vi "ZController.vi"() -> ()   [LabVIEW 2016]
uses:
  controls/FPGAVIreferenceTypeDef.ctl
  controls/Enum.ctl
  <vilib>/event_ctls.llb/lveventtype.ctl
  controls/EnumSM.ctl
  Course Project/support/Message Queue/Message Cluster.ctl
  <vilib>/FPGAPlugInAG/USB-7856R OEM/niLvFpga_Close_USB-7856R OEM.vi
  <vilib>/FPGAPlugInAG/USB-7856R OEM/niLvFpga_Reset_USB-7856R OEM.vi
  <vilib>/rvi/errors/niLvFpgaAdjustHostInterfaceError.vi
  <vilib>/RVI Host/nirviSupport.llb/nirviErrorClusterFromErrorCode.vi
  <vilib>/Utility/config.llb/Read Key (Boolean).vi
  <vilib>/Utility/config.llb/Read Key (Double).vi
  <vilib>/Utility/config.llb/Read Key (String).vi
  <vilib>/Utility/config.llb/Read Key (U32).vi
  <vilib>/Utility/config.llb/Write Key (String).vi
  <vilib>/Utility/config.llb/Write Key (U32).vi
  <vilib>/Utility/config.llb/Write Key (Double).vi
  <vilib>/Utility/config.llb/Write Key (Boolean).vi
  <vilib>/rvi/interface/nirviCloseFPGA/nirviCloseFPGA.xnode
  FPGA Bitfiles/qnmController797_usbRIO_controllerFPGAmu.lvbitx
  <vilib>/rvi/interface/nirviMethod/nirviMethod.xnode
  <vilib>/rvi/interface/nirviReadWriteControl/nirviReadWriteControl.xnode
  controls/FPGAVIreferenceTypeDefScanEngine.ctl
  <vilib>/regexp/Match Regular Expression.xnode
  Course Project/support/Message Queue/Message Queue.lvlib
  Course Project/support/User Event - Stop/User Event - Stop.lvlib
  NiFpgaLv.dll
  <vilib>/Utility/config.llb/NI_LVConfig.lvlib
  <vilib>/FPGAPlugInAG/USB-7856R OEM/niLvFpga_AcknowledgeIrq_USB-7856R OEM.vi
  <vilib>/rvi/interface/nirviMethod/StockFPGA_InlinedMethodWaitForSingleIRQ.vi
  <vilib>/FPGAPlugInAG/USB-7856R OEM/niLvFpga_WaitOnIrq_USB-7856R OEM.vi
panel:
  in  "ms":u32=50 format="%.0fms"
  in  "ZControllerThumbnail":enum32{"Z controller", "Other Config"}(tab)
  out "Surface reached":bool
  in  "Steps":u32=16 format="%#.0p"
  out "Approaching?":bool
  in  "Mode":enum16{"Contact", "OR Tapping", "Aux"}(ring)
  in  "Feedback On":bool caption="Enable"
  in  "liftHeight":dbl=1e-07 format="%.2pm"
  in  "Lift":bool
  in  "Motor":cluster{"Up":bool, "Down":bool}
  in  "Z (m)":dbl(slide) scale=1.75e-06..-1.75e-06 scale format="%#.2p"
  in  "PID":T1={"Setpoint"=0.05, "P Gain"=0.0001, "I Gain"=0.0003} {"I Gain" max=20.0 format="%.3p"; "P Gain" format="%.3p"; "Setpoint" format="%_4pV"}
  in  "Withdraw":bool
  in  "AutoApproach":cluster{"Stop":bool, "Start":bool}
  in  "Wait":u32=1 format="%.0fms"
  in  "DCVoltage":sgl=1.2 format="%#_3pV"
  in  "IO Frequency":u32=1000000 format="%.1p"
  in  "Relative Setpoint":bool
  in  "SafeTip":T2 {"SafeTipSignal" items=["AI0", "AI1", "AI2", "AI3", "AI4", "AI5", "AI6", "AI7"]; "SafeTipValue" format="%_3p"}
  in  "Slow":bool
  in  "Beep when finished":bool=TRUE
  in  "Withdraw/landed":bool=TRUE
  in  "Ztreshold":dbl=0.949999988079071
  in  "zMoveTresh":fxp<+/-,29,2>=0.009999997913837433 format="%#_4g"
  in  "InvertHeight":bool=TRUE
  in  "Type":T3(ring)
  in  "Decimations":cluster{"Withdraw":u16, "ManualMove":u16}={"Withdraw"=5, "ManualMove"=5}
  in  "Step Up":enum16{"Z+", "Z-"}(ring)=enum."Z-"
  out "Display Z":bool=TRUE
  in  "WaveSize":u16=101
  out "Zstep":i32
  # "Mode"
  # "Z (m)"
  # "Motor"
  # "Feedback"
  # "Approach"
  # "Motor"
  # "SetPoint"
  # "Manual PID"
  # "Auto approach"
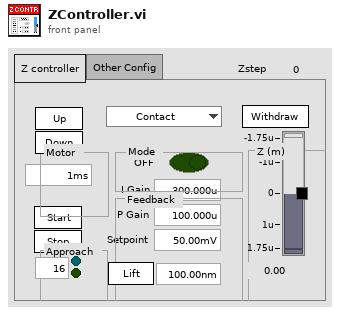
[diagram p1: front panel]
types:
  T1 = cluster{"Setpoint":dbl, "P Gain":dbl, "I Gain":dbl}
  T2 = cluster{"SafeTipValue":dbl, ">/<":enum16{">", "<"}, "SafeTipOn":bool, "SafeTipSignal":u16}
  T3 = enum16{"Step motor", "DC motor", "Stepper Motor Driver", "Stick-Slip"}
  T4 = typedef "FPGAVIreferenceTypeDef.ctl" = refnum<k20>
  T5 = typedef "Enum.ctl" = enum16{"Init", "Read", "Write"}
  T6 = enum16{"fractional", "engineering", "exponential"}
  T7 = enum16{"Vert. Deflection", "Horiz. Deflection", "Amplitude", "..."}
  T8 = cluster{"inverseDecimation":fxp<+,22,0>, "decimation":u16, "waveSize":u16, "pixelDecimation":u16}
  T9 = cluster{"enableManualMotion":bool, "doMove":bool, "integratorTarget":fxp<+/-,22,2>, "clocks":cluster{"inverseDecimation":fxp<+,22,0>, "decimation":u16, "waveSize":u16, "pixelDecimation":u16}}
  T10 = typedef "EnumSM.ctl" = enum16{"Init.Calibrations", "Init.Excitation", "Init.StepMotor", "Init.FeedbackMotion", "Init.Scan", "Init.Signals", "Init.System", "Init.Waveform", "Init.ZController", "Send.Waveform", "Correct.Hysteresis"}
  T11 = cluster{"Width":dbl, "Height":dbl, "X Offset":dbl, "Y Offset":dbl, "Angle":dbl, "Pixels/Line":u16, "Lines":u16, "Time/Line":dbl, "Scan Rate":dbl}
  T12 = enum8{"Enabled", "Disabled", "Disabled and Grayed Out"}
  T13 = cluster{"setPoint":fxp<+/-,17,1>, "pGain":dbl, "iGain":dbl, "setPointAlt":fxp<+/-,17,1>}
  T14 = enum16{"Contact", "OR Tapping", "Aux", "Intermittent Contact"}
  T15 = cluster{"enableManualMotion":bool, "doMove":bool, "liftHeight":dbl}
  T16 = typedef "Message Queue.lvlib/Message Cluster.ctl" = cluster{"Message":string, "Données de message":variant}
  T17 = enum32{"Invalid", "Standard", "Closed", "Hidden", "Minimized", "Maximized"}
  T18 = enum32{"Bad", "Idle", "Run top level", "Running"}
  T19 = typedef "lveventtype.ctl" = enum32{"Null", "Timeout", "Annotation Menu Selection", "Annotation Menu Selection?", "App Instance Close", "App Instance Close?", "Autoscale Range Change", "Bookmark Info Change", "Cell Edit", "Cell Edit?", "Cursor Grab", "Cursor Grab?", "Cursor Menu Selection", "Cursor Menu Selection?", "Cursor Move", "Cursor Release", "Data Change", "Direction Change", "Display State Change", "Drag Ended", "Drag Enter", "Drag Leave", "Drag Over", "Drag Source Update", "Drag Starting", "Drag Starting?", "Drop", "Exec State Change", "Key Down", "Key Down?", "Key Repeat", "Key Repeat?", "Key Up", "Listbox Double Click", "Menu Activation?", "Menu Selection (App)", "Menu Selection? (App)", "Menu Selection (User)", "Mouse Down", "Mouse Down?", "Mouse Enter", "Mouse Leave", "Mouse Move", "Mouse Up", "Mouse Wheel", "NI Security User Change (App)", "Pane Size", "Panel Close", "Panel Close?", "Panel Resize", "Plot Attribute Change", "Scale Range Change", "Shortcut Menu Activation?", "Shortcut Menu Selection (App)", "Shortcut Menu Selection? (App)", "Shortcut Menu Selection (User)", "Tree Double Click", "Tree Drag", "Tree Drag?", "Tree Drop", "Tree Drop?", "Tree Item Close", "Tree Item Close?", "Tree Item Open", "Tree Item Open?", "User Event", "Value Change"}
  T20 = typedef "Message Queue.lvlib/All Message Queues.ctl" = cluster{"IU":refnum<queue>}
  T21 = typedef "NI_LVConfig.lvlib/Config Data RefNum.ctl" = refnum<k1>
  T22 = cluster{"calibName":string[], "calibParameters":cluster{"Sensitivity":cluster{"Sens X":dbl, "Sens Y":dbl, "Sens Z":dbl}, "Range":cluster{"Range X":dbl, "Range Y":dbl, "Range Z":dbl}, "HV gain":cluster{"HV gain X":dbl, "HV gain Y":dbl, "HV gain Z":dbl}}[], "calibIndex":i32}
  T23 = cluster{"Sensitivity":cluster{"Sens X":dbl, "Sens Y":dbl, "Sens Z":dbl}, "Range":cluster{"Range X":dbl, "Range Y":dbl, "Range Z":dbl}, "HV gain":cluster{"HV gain X":dbl, "HV gain Y":dbl, "HV gain Z":dbl}}[]
  T24 = cluster{"Sensitivity":cluster{"Sens X":dbl, "Sens Y":dbl, "Sens Z":dbl}, "Range":cluster{"Range X":dbl, "Range Y":dbl, "Range Z":dbl}, "HV gain":cluster{"HV gain X":dbl, "HV gain Y":dbl, "HV gain Z":dbl}}
  T25 = typedef "FPGAVIreferenceTypeDefScanEngine.ctl" = refnum<k20>
  T26 = cluster{"liftHeight":fxp<+/-,15,4>, "disengagePos":fxp<+/-,22,1>}
  T27 = cluster{"upperLimit":fxp<+/-,28,4>, "lowerLimit":fxp<+/-,28,4>}
  T28 = cluster{"Width":bool, "Height":bool, "X Offset":bool, "Y Offset":bool, "Angle":bool, "Pixels/Line":bool, "Lines":bool, "Time/Line":bool, "Scan Rate":bool}
  T29 = cluster{"target ":i16, "increment":i16, "ClockDivider":i16, "axis":enum16{"none", "x", "y", "z"}}
  T30 = cluster{"sicm.p.enable":bool, "sicm.p.adaptiveStepDown":bool, "sicm.p.relSetpoint":bool}
  T31 = cluster{"ort.p.winSizeP2":u16, "ort.p.syncPoint":u16, "ort.p.useSyncPoint":bool, "ort.p.bypassAvg":bool, "ort.p.searchBounds":cluster{"maxSearchLower":u16, "maxSearchUpper":u16}}
  T32 = cluster{"scanEngineHz":u32, "feedbackHz":u32, "sicmHz":u32, "rampHz":u32}
  T33 = cluster{"SafeTipValue":dbl, ">/<":enum16{">", "<"}, "SafeTipSignal":u16}
  T34 = cluster{"enableManualMotion":bool, "doMove":bool, "HeightTarget(0-2)":dbl}
  T35 = cluster{"enableManualMotion":bool, "doMove":bool, "Height Lift":dbl, "Caption.Text":string}
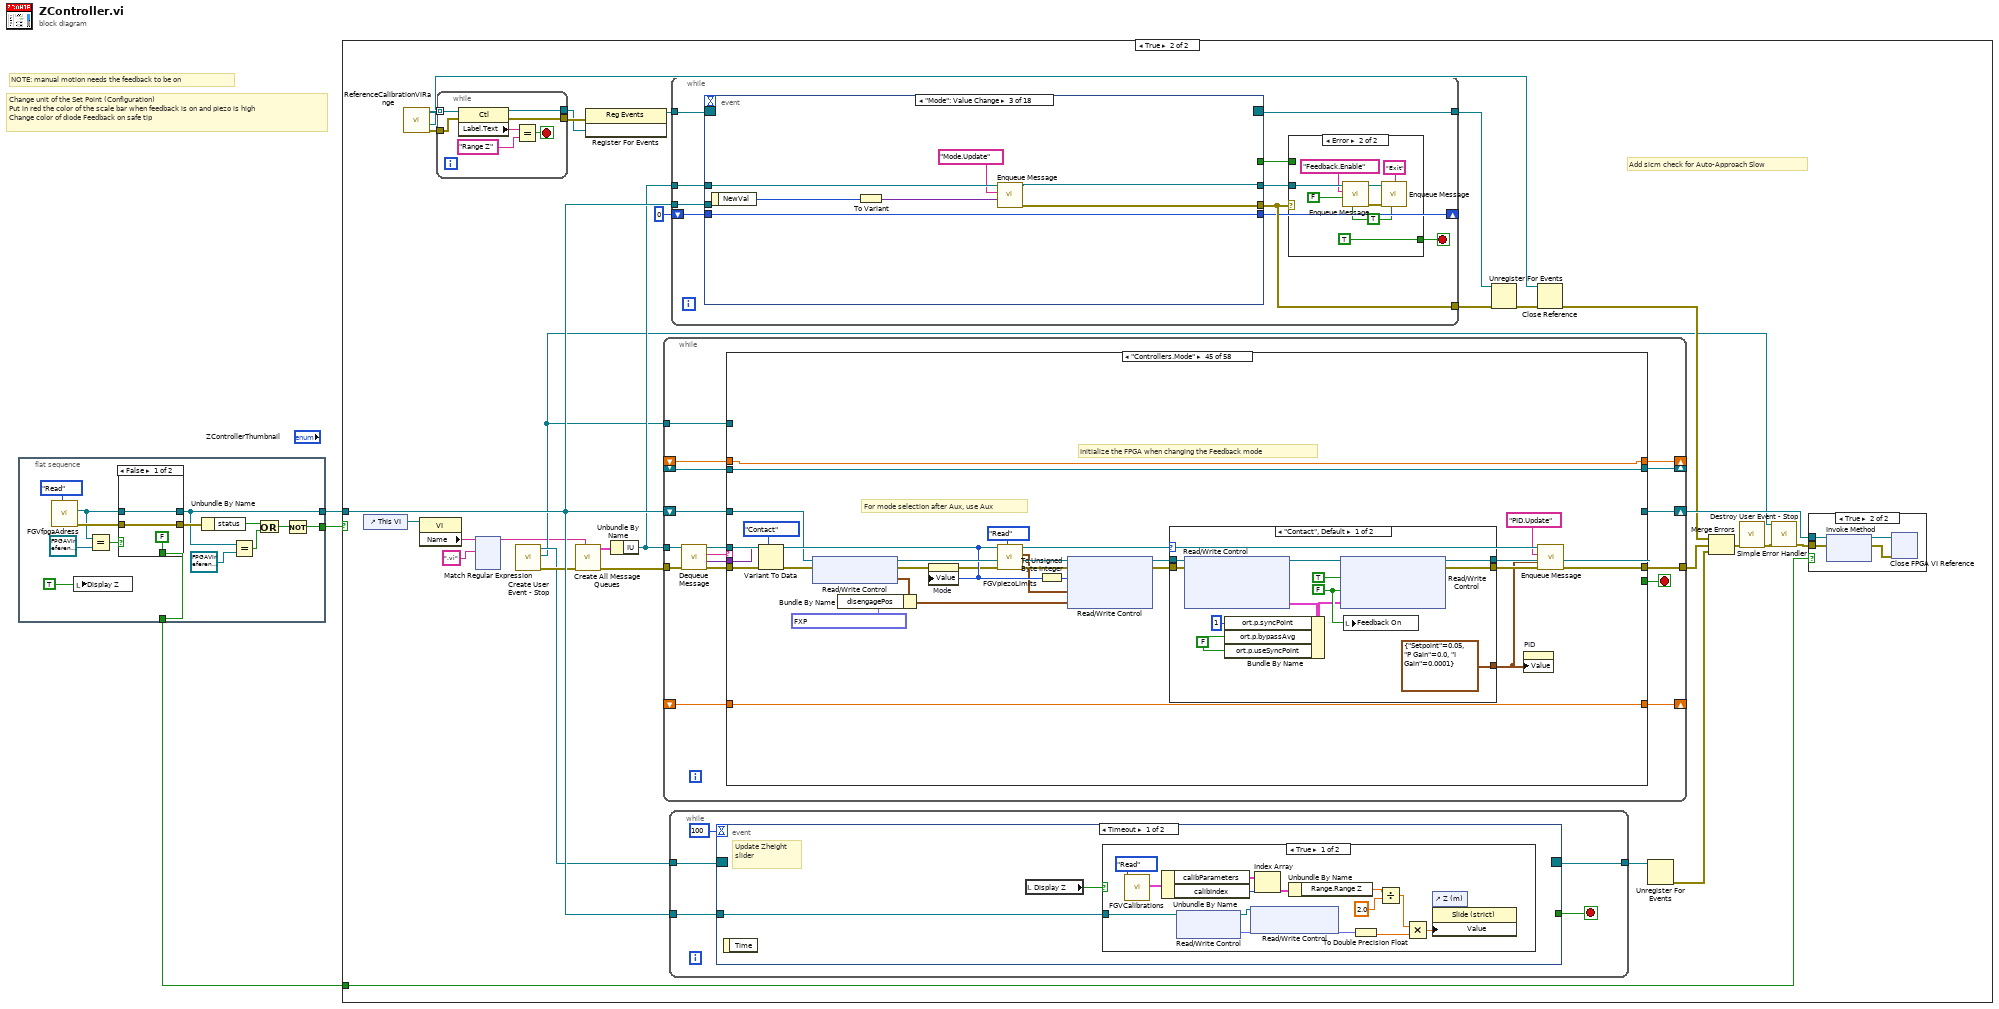
[diagram p0: block diagram]
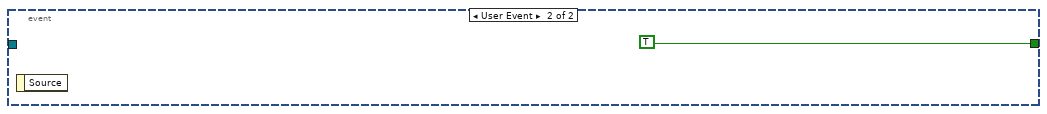
[diagram p5: hidden frame]
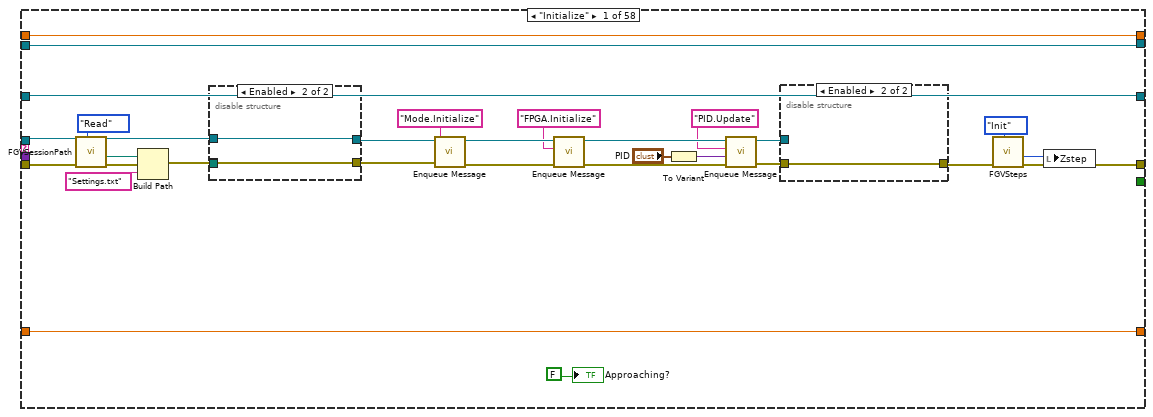
[diagram p6: hidden frame]
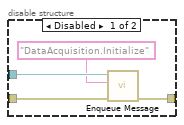
[diagram p7: hidden frame]
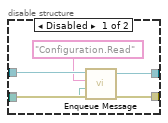
[diagram p8: hidden frame]
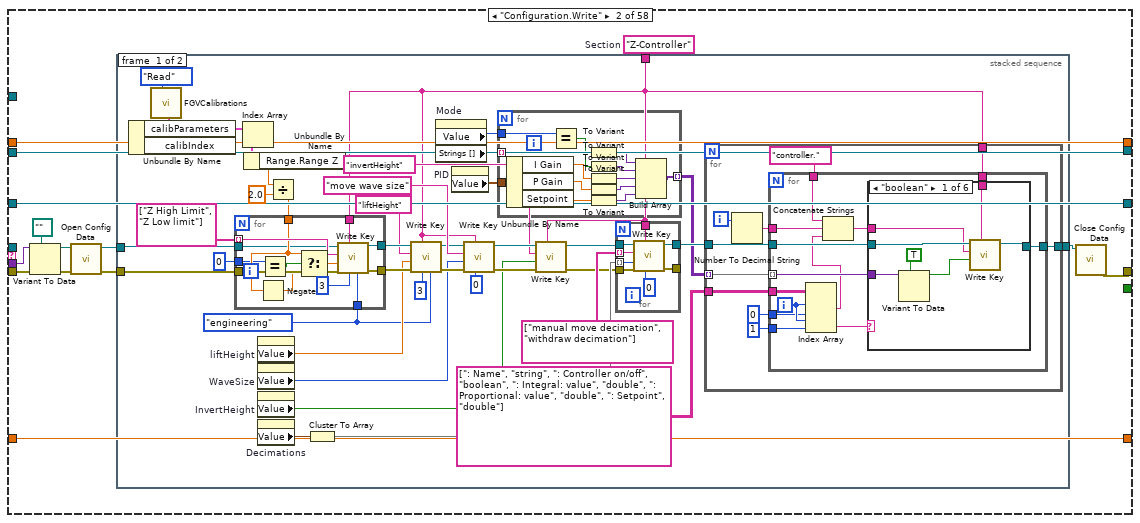
[diagram p9: hidden frame]
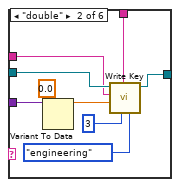
[diagram p10: hidden frame]
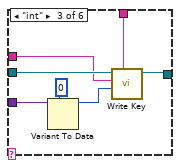
[diagram p11: hidden frame]
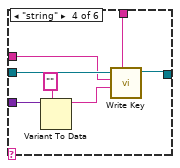
[diagram p12: hidden frame]
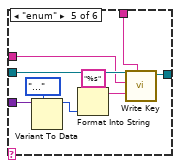
[diagram p13: hidden frame]
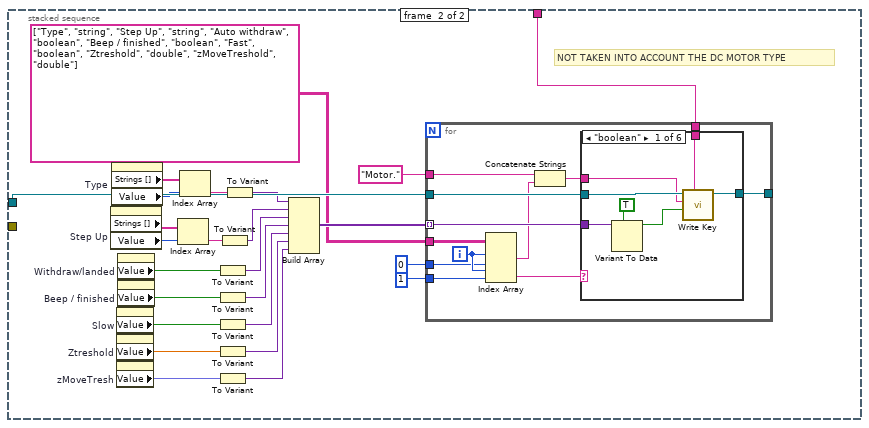
[diagram p15: hidden frame]
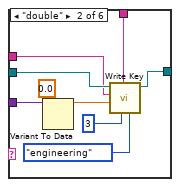
[diagram p16: hidden frame]
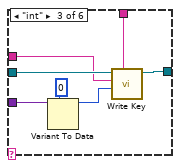
[diagram p17: hidden frame]
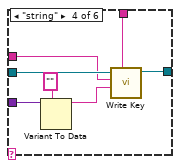
[diagram p18: hidden frame]
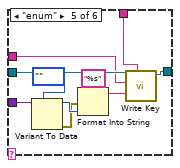
[diagram p19: hidden frame]
diagram:
  # "Change unit of the Set Point (Configuration)\nPut in red the color of the scale bar when feedback is on and piezo is high\nChange color of diode Feedback on safe tip"
  # "NOTE: manual motion needs the feedback to be on"
  n1 = flat-sequence {
    tunnel: [w6] -> w3
    tunnel: [w5] -> w2
    tunnel: [w4] -> _
    tunnel: [w4] -> w1
    frame #0 {
      n2 = call "FGVfpgaAdress.vi"("Enum"=Enum."Read") -> ("error out"=w17:errorcluster, "FPGA VI Reference Out"=w10:T4)  [unwired: 5 in, 4 out]
      n3 = local write "Display Z"(TRUE ("display height")) -> ()
      n4 = Equal?(x=w10, y=T4 refnum ("FPGA VI Reference Out")) -> (x = y?=w15:bool)
      n5 = case shown="False" w15 {
        tunnel: [w20 w26] -> w6
        tunnel: [w19 w25] -> w7
        tunnel: w17 -> [w19 w24]
        tunnel: w10 -> [w20 w23]
        tunnel: [FALSE TRUE] -> w4
        frame False {
        }
        frame True {
          n6 = call "FGVfpgaAdress.vi"("Enum"=Enum."Init", "error in"=w24, "FPGA VI Reference In"=w23) -> ("error out"=w25:errorcluster, "FPGA VI Reference Out"=w26:T4)  [unwired: 3 in, 4 out]
        }
      }
      n7 = Unbundle By Name(w7) -> ("status"=w12:bool)
      n8 = Equal?(x=w6, y=T4 refnum ("FPGA VI Reference Out")) -> (x = y?=w13:bool)
      n9 = Or(x=w12, y=w13) -> (x .or. y?=w14:bool)
      n10 = Not(x=w14) -> (.not. x?=w5:bool)
    }
  }
  n11 = case shown="True" w2 {
    tunnel: w3 -> [_ w55]
    tunnel: w1 -> [_ w41]
    frame False {
    }
    frame True {
      # "Add sicm check for Auto-Approach Slow"
      n12 = control-ref of="This VI"() -> (w31:refnum<vi>)
      n13 = call "ReferenceCalibrationViRange.vi"() -> ("error out"=w45:errorcluster, "vi reference"=w39:refnum<vi>, "Ranges"=w46:refnum<vi>[])  [unwired: 8 in, 1 out]
      n14 = property class="VI"(reference=w31) -> ("Name"=w30:string)  [unwired: 1 in, 2 out]
      n15 = while {
        tunnel: w46 -> [w180] mode=indexing
        tunnel: [w181] -> w44
        tunnel: w45 -> [w179]
        tunnel: [w175] -> w43
        stop <- w176 stop-if-true
        n16 = property class="Ctl"(reference=w180, error in=w179) -> (reference out=w175:refnum<vi>, error out=w181:errorcluster, "Label.Text"=w178:string)
        n17 = Equal?(x=w178, y="Range Z") -> (x = y?=w176:bool)
      }
      n18 = xnode "Match Regular Expression"("input string"=w30, "regular expression"=".vi") -> ("before match"=w28:string)  [unwired: 4 in, 4 out]
      n19 = call "Create User Event - Stop.vi"() -> ("sortie d'erreur"=w38:errorcluster, "Événement utilisateur - Arrêt"=w32:refnum<user-event>, "Refnum Enregistrement à l'événement Arrêt"=w37:refnum<event-registration>)  [unwired: 9 in]
      n20 = call "Create All Message Queues.vi"("QueueName"=w28, "ErrorIn"=w38) -> ("ErrorOut"=w49:errorcluster, "MessageQueueOut"=w51:T20)  [unwired: 8 in]
      n21 = register-events(error in=w44, w43) -> (reference out=w47:refnum<event-registration>)  [unwired: 1 in, 1 out]
      n22 = Unbundle By Name(w51) -> ("IU"=w50:refnum<queue>)
      n23 = while {
        tunnel: w50 -> [w214]
        tunnel: w49 -> [w218]
        tunnel: [w219] -> w48
        shift-right: [w213] -> w56
        shift-left: w55 -> [w212]
        shift-right: [w210] -> _
        shift-left: _ -> [w209]
        shift-right: [w207] -> _
        shift-left: _ -> [w208]
        tunnel: w32 -> [w206]
        shift-right: [w204] -> _
        shift-left: _ -> [w205]
        stop <- w220 stop-if-true
        n24 = call "Dequeue Message.vi"("entrée d'erreur (pas d'erreur)"=w218, "File d'attente de messages"=w214) -> ("sortie d'erreur"=w217:errorcluster, "Données de message"=w216:variant, "Message"=w211:string, "File d'attente de message dup."=w215:refnum<queue>)  [unwired: 6 in]
        n25 = case "Conditions des messages" shown="\"Controllers.Mode\"" w211 {
          selector: w211 -> [_ _ _ _ _ _ _ _ _ _ _ _ _ _ _ _ _ _ _ _ _ _ _ _ _ _ _ _ _ _ _ _ _ _ _ _ _ _ _ _ _ _ _ _ _ _ _ _ _ _ _ _ _ _ _ _ _ w2503]
          tunnel: w215 -> [w248 _ _ w682 _ _ _ _ w811 w833 w923 _ w937 _ _ w1103 _ _ w1163 _ _ _ _ w1354 _ _ _ w1486 _ _ w1563 _ w1612 w1653 w1733 w1796 _ w1828 w1861 w1962 w2042 w2110 _ w2162 w2187 w2227 _ _ _ _ w2363 _ _ _ w2468 _ w2495 _]
          tunnel: w217 -> [w225 w266 w501 w659 w698 w735 w766 w781 w808 w831 w925 w930 w958 w1045 w1064 w1092 w1147 w1156 w1185 w1258 w1265 w1285 w1320 w1355 w1387 w1400 w1459 w1481 w1528 w1546 w1551 w1593 w1608 w1650 w1725 w1794 w1818 w1829 w1859 w1960 w2041 w2108 w2142 w2144 w2184 w2216 w2242 w2261 w2317 w2341 w2361 w2378 w2386 w2396 w2469 w2477 w2492 _]
          tunnel: [w241 w269 w503 w676 w698 w725 w767 w781 w803 w824 w910 w930 w944 w1053 w1064 w1079 w1146 w1156 w1159 w1257 w1265 w1270 w1322 w1348 w1373 w1418 w1433 w1485 w1521 w1546 w1555 w1590 w1607 w1648 w1728 w1797 w1818 w1830 w1853 w1954 w2038 w2111 w2142 w2145 w2168 w2212 w2242 w2256 w2316 w2342 w2351 w2367 w2386 w2394 w2463 w2478 w2493 w2501] -> w219
          tunnel: [_ _ _ _ _ _ _ _ _ _ _ _ _ _ _ _ _ _ _ _ _ _ _ _ _ _ _ _ _ _ _ _ _ _ _ _ _ _ _ _ _ _ _ _ _ _ _ _ _ _ _ _ _ _ _ _ TRUE _] -> w220
          tunnel: w216 -> [_ w265 w500 _ _ _ _ _ w809 w832 _ _ w957 _ _ w1090 _ _ w1184 _ _ w1284 w1318 _ w1386 w1426 _ _ w1527 _ _ _ _ _ _ _ _ _ _ _ w2040 _ _ w2143 w2185 w2214 _ w2260 _ w2340 _ w2377 _ w2388 _ _ _ _]
          tunnel: w212 -> [w235 w275 w507 w671 w697 w737 w764 w780 w804 w814 w922 w929 w965 w1059 w1063 w1100 w1149 w1155 w1198 w1260 w1264 w1283 w1302 w1349 w1382 w1406 w1458 w1484 w1530 w1545 w1547 w1592 w1602 w1649 w1724 w1791 w1817 w1827 w1858 w1959 w2035 w2109 w2141 w2158 w2181 w2220 w2241 w2278 w2330 w2334 w2360 w2380 w2385 w2398 w2472 w2483 w2491 w2499]
          tunnel: [w235 w275 w507 w681 w697 w726 w763 w780 w804 w814 w922 w929 w965 w1059 w1063 w1100 w1149 w1155 w1198 w1260 w1264 w1287 w1317 w1349 w1375 w1412 w1460 w1484 w1529 w1545 w1552 w1591 w1609 w1647 w1721 w1790 w1817 w1827 w1850 w1951 w2035 w2107 w2141 w2158 w2175 w2211 w2241 w2278 w2330 w2334 w2360 w2380 w2385 w2397 w2472 w2483 w2491 w2499] -> w213
          tunnel: [w232 w274 w506 w664 w683 w751 w776 w779 w784 w816 w907 w928 w964 w1058 w1062 w1099 w1151 w1154 w1197 w1259 w1263 w1273 w1311 w1345 w1364 w1397 w1445 w1483 w1531 w1544 w1561 w1595 w1611 w1652 w1732 w1800 w1816 w1825 w1836 w1938 w2034 w2104 w2140 w2157 w2174 w2226 w2240 w2277 w2329 w2333 w2355 w2366 w2384 w2417 w2471 w2482 w2489 w2498] -> w210
          tunnel: w209 -> [w232 w274 w506 _ _ w751 w776 w779 w784 w816 w907 w928 w964 w1058 w1062 w1099 w1151 w1154 w1197 w1259 w1263 w1273 w1311 w1345 w1364 w1397 w1445 w1483 w1531 w1544 w1561 w1595 w1611 w1652 w1732 w1800 w1816 w1825 w1836 w1938 w2034 w2104 w2140 w2157 w2174 w2226 w2240 w2277 w2329 w2333 w2355 _ w2384 w2417 w2471 w2482 w2489 w2498]
          tunnel: w208 -> [w231 w273 w505 w651 w696 w721 w775 w778 w783 w815 w906 w927 w950 w1052 w1061 w1097 w1145 w1153 w1166 w1256 w1262 w1272 w1301 w1344 w1363 w1395 w1444 w1482 w1525 w1543 w1560 w1594 w1610 w1651 w1731 w1799 w1815 w1824 w1835 w1937 w2033 w2103 w2139 w2156 w2172 w2225 w2239 w2276 w2328 w2332 w2354 w2365 w2383 w2416 w2470 w2481 w2488 w2497]
          tunnel: [w231 w273 w505 w661 w696 w721 w775 w778 w783 w813 w906 w927 w945 w1051 w1061 w1102 w1144 w1153 w1165 w1255 w1262 w1272 w1300 w1344 w1363 w1395 w1444 w1482 w1525 w1543 w1560 w1594 w1610 w1651 w1731 w1799 w1815 w1824 w1835 w1937 w2033 w2103 w2139 w2156 w2172 w2225 w2239 w2276 w2328 w2332 w2354 w2365 w2383 w2416 w2470 w2481 w2488 w2497] -> w207
          tunnel: w206 -> [_ _ _ _ _ _ _ _ _ _ _ _ _ _ _ _ _ _ _ _ _ _ _ _ _ _ _ _ _ _ _ _ _ _ _ _ _ _ _ _ _ _ _ _ _ _ _ _ _ _ _ _ _ _ _ _ w2487 _]
          tunnel: w205 -> [w221 w263 w494 _ w695 w701 w760 w777 w782 w812 w905 w926 w940 w1047 w1060 w1098 w1150 w1152 w1158 w1253 w1261 w1266 w1327 w1343 w1356 w1391 w1437 w1476 w1524 w1542 w1553 w1581 w1603 w1630 w1726 w1795 w1814 w1819 w1833 w1963 w2032 w2102 w2138 w2155 w2171 w2217 w2238 w2275 w2327 w2331 w2353 w2364 w2382 w2387 w2461 w2480 w2485 w2496]
          tunnel: [w221 w263 w494 w648 w695 w701 w760 w777 w782 w812 w905 w926 w940 w1047 w1060 w1098 w1150 w1152 w1158 w1253 w1261 w1266 w1327 w1343 w1356 w1391 w1437 w1476 w1524 w1542 w1553 w1581 w1603 w1630 w1726 w1795 w1814 w1819 w1833 w1963 w2032 w2102 w2138 w2155 w2171 w2217 w2238 w2275 w2327 w2331 w2353 w2364 w2382 w2387 w2461 w2480 w2485 w2496] -> w204
          frame "Initialize" {
            n26 = call "FGVSessionPath.vi"("Enum"=Enum."Read", "error in"=w225) -> ("error out"=w249:errorcluster, "sessionPathOut"=w229:path)  [unwired: 8 in]
            n27 = Build Path(base path=w229, name or relative path="Settings.txt") -> (appended path=w227:path)
            n28 = disable-structure shown="Enabled" {
              disable-tunnel: w249 -> [w260 w261]
              disable-tunnel: w248 -> [w259 w262]
              disable-tunnel: [w258 w262] -> w247
              disable-tunnel: [w257 w261] -> w230
              disable-tunnel: w227 -> [w255 _]
              frame Disabled {
                n29 = call "Enqueue Message.vi"("error in"=w260, "Data"=w255, "Message"="Configuration.Read", "Queue"=w259) -> ("error out"=w257:errorcluster, "Queue dup."=w258:refnum<queue>)  [unwired: 6 in]
              }
              frame Enabled {
              }
            }
            n30 = call "Enqueue Message.vi"("error in"=w230, "Message"="Mode.Initialize", "Queue"=w247) -> ("error out"=w243:errorcluster, "Queue dup."=w245:refnum<queue>)  [unwired: 7 in]
            n31 = call "Enqueue Message.vi"("error in"=w243, "Message"="FPGA.Initialize", "Queue"=w245) -> ("error out"=w237:errorcluster, "Queue dup."=w246:refnum<queue>)  [unwired: 7 in]
            n32 = To Variant(anything="PID") -> (Variant=w233:variant)
            n33 = call "Enqueue Message.vi"("error in"=w237, "Data"=w233, "Message"="PID.Update", "Queue"=w246) -> ("error out"=w223:errorcluster, "Queue dup."=w224:refnum<queue>)  [unwired: 6 in]
            n34 = disable-structure shown="Enabled" {
              disable-tunnel: w224 -> [w253 _]
              disable-tunnel: w223 -> [w252 w254]
              disable-tunnel: [w251 w254] -> w222
              frame Disabled {
                n35 = call "Enqueue Message.vi"("error in"=w252, "Message"="DataAcquisition.Initialize", "Queue"=w253) -> ("error out"=w251:errorcluster)  [unwired: 7 in, 1 out]
              }
              frame Enabled {
              }
            }
            n36 = call "FGVSteps.vi"("Enum"=Enum."Init", "error in"=w222) -> ("error out"=w241:errorcluster, "stepglobalCounterOut"=w239:i32)  [unwired: 6 in, 2 out]
            n37 = local write "Zstep"(w239) -> ()
            "Approaching?" <- FALSE ("Approaching?")
          }
          frame "Configuration.Write" {
            w272 = "Z-Controller"  # Section
            n38 = Variant To Data(error in=w266, type=path "" ("appended path"), Variant=w265) -> (data=w268:path, error out=w267:errorcluster)
            n39 = call <vilib>:"Open Config Data.vi"("error in (no error)"=w267, "configuration file path"=w268) -> ("error out"=w276:errorcluster, "refnum"=w271:T21)  [unwired: 1 in, 7 out]
            n40 = stacked-sequence {
              tunnel: w276 -> [w316 _]
              tunnel: w272 -> [w277 w431]
              tunnel: w271 -> [w293 w440]
              tunnel: [w292 _] -> w270
              frame #0 {
                w308 = T6."engineering" ("format (fractional)")
                n41 = call "FGVCalibrations.vi"("Enum"=Enum."Read") -> ("calibOut"=w297:T22)  [unwired: 9 in, 1 out]
                n42 = Unbundle By Name(w297) -> ("calibParameters"=w296:T23, "calibIndex"=w295:i32)
                n43 = Index Array(array=w296, index=w295) -> (element=w305:T24)
                n44 = Unbundle By Name(w305) -> ("Range.Range Z"=w306:dbl)
                n45 = property on="liftHeight" class="DigNum (strict)"() -> ("Value"=w313:dbl)  [unwired: 2 in, 2 out]
                n46 = property on="WaveSize" class="DigNum (strict)"() -> ("Value"=w286:u16)  [unwired: 2 in, 2 out]
                n47 = property on="InvertHeight" class="Bool (strict)"() -> ("Value"=w278:bool)  [unwired: 2 in, 2 out]
                n48 = property on="Decimations" class="Clust (strict)"() -> ("Value"=w310:cluster{"Withdraw":u16, "ManualMove":u16})  [unwired: 2 in, 2 out]
                n49 = Divide(x=w306, y=2.0) -> (x/y=w294:dbl)
                n50 = for {
                  tunnel: string[] ["Z High Limit", "Z Low limit"] -> [w411] mode=indexing
                  tunnel: w294 -> [w409]
                  tunnel: w277 -> [w408]
                  tunnel: [w407] -> w301
                  tunnel: w293 -> [w406]
                  tunnel: [w405] -> w315
                  tunnel: w308 -> [w404]
                  tunnel: 0 ("x") -> [w403]
                  tunnel: w316 -> [w415]
                  i -> [w412]
                  n51 = Negate(x=w409) -> (-x=w410:dbl)
                  n52 = Equal?(x=w403, y=w412) -> (x = y?=w413:bool)
                  n53 = Select(t=w409, s=w413, f=w410) -> (s? t:f=w414:dbl)
                  n54 = call-poly <vilib>:"Write Key.vi"("format (fractional)"=w404, "precision (6)"=i16 3, "section"=w408, "error in (no error)"=w415, "value"=w414, "key"=w411, "refnum"=w406) -> ("error out"=w405:errorcluster, "refnum out"=w407:T21)  [unwired: 1 in, 2 out]
                }
                n55 = Cluster To Array(cluster=w310) -> (array=w289:u16[])
                n56 = call-poly <vilib>:"Write Key.vi"("format (fractional)"=w308, "precision (6)"=i16 3, "section"=w277, "error in (no error)"=w315, "value"=w313, "key"="liftHeight", "refnum"=w301) -> ("error out"=w288:errorcluster, "refnum out"=w285:T21)  [unwired: 1 in, 2 out]
                n57 = property on="Mode" class="Enum (strict)"() -> ("Value"=w309:enum16{"Contact", "OR Tapping", "Aux"}, "Strings []"=w311:string[])  [unwired: 2 in, 2 out]
                n58 = property on="PID" class="Clust (strict)"() -> ("Value"=w312:T1)  [unwired: 2 in, 2 out]
                n59 = call-poly <vilib>:"Write Key.vi"("precision (6)"=i16 0, "section"=w277, "error in (no error)"=w288, "value"=w286, "key"="move wave size", "refnum"=w285) -> ("error out"=w283:errorcluster, "refnum out"=w281:T21)  [unwired: 2 in, 2 out]
                n60 = for {
                  tunnel: w309 -> [w322]
                  tunnel: [w319] -> w299 mode=indexing
                  tunnel: w311 -> [w318] mode=indexing
                  tunnel: w312 -> [w317]
                  i -> [w323]
                  n61 = Unbundle By Name(w317) -> ("I Gain"=w330:dbl, "P Gain"=w329:dbl, "Setpoint"=w328:dbl)
                  n62 = Equal?(x=w322, y=w323) -> (x = y?=w321:bool)
                  n63 = To Variant(anything=w318) -> (Variant=w327:variant)
                  n64 = To Variant(anything=w321) -> (Variant=w320:variant)
                  n65 = To Variant(anything=w330) -> (Variant=w326:variant)
                  n66 = To Variant(anything=w329) -> (Variant=w325:variant)
                  n67 = To Variant(anything=w328) -> (Variant=w324:variant)
                  n68 = Build Array(w327, w320, w326, w325, w324) -> (w319:variant[])
                }
                n69 = call-poly <vilib>:"Write Key.vi"("section"=w277, "error in (no error)"=w283, "value"=w278, "key"="invertHeight", "refnum"=w281) -> ("error out"=w282:errorcluster, "refnum out"=w280:T21)  [unwired: 5 out]
                n70 = for {
                  tunnel: w277 -> [w338]
                  tunnel: w280 -> [w337]
                  tunnel: w282 -> [w336]
                  tunnel: string[] ["manual move decimation", "withdraw decimation"] -> [w335] mode=indexing
                  tunnel: w289 -> [w334] mode=indexing
                  tunnel: [w333] -> _
                  tunnel: [w332] -> w307
                  n71 = call-poly <vilib>:"Write Key.vi"("precision (6)"=i16 0, "section"=w338, "error in (no error)"=w336, "value"=w334, "key"=w335, "refnum"=w337) -> ("error out"=w333:errorcluster, "refnum out"=w332:T21)  [unwired: 2 in, 2 out]
                }
                n72 = for {
                  tunnel: string[][] [[": Name", "string"], [": Controller on/off", "boolean"], [": Integral: value", "double"], [": Proportional: value", "double"], [": Setpoint", "double"]] ("appended array") -> [w341]
                  tunnel: w299 -> [w347] mode=indexing
                  tunnel: w277 -> [w348]
                  tunnel: w307 -> [w346]
                  tunnel: [w345] -> w292
                  i -> [w344]
                  n73 = Number To Decimal String(number=w344) -> (decimal integer string=w342:string)  [unwired: 1 in]
                  n74 = for {
                    tunnel: w348 -> [w361]
                    tunnel: w347 -> [w360] mode=indexing
                    tunnel: w346 -> [w359]
                    tunnel: [w358] -> w345
                    tunnel: "controller." -> [w357]
                    tunnel: w342 -> [w356]
                    tunnel: w341 -> [w355]
                    tunnel: 0 ("disabled index (col)") -> [w352]
                    tunnel: 1 ("disabled index (col)") -> [w351]
                    i -> [w354]
                    n75 = Index Array(array=w355, index (row) #1=w354, index (col) #1=w352, index (row) #2=w354, index (col) #2=w351) -> (element #1=w350:string, element #2=w353:string)
                    n76 = Concatenate Strings(w357, w356, w350) -> (w349:string)
                    n77 = case shown="\"boolean\"" w353 {
                      tunnel: w361 -> [w365 w374 w381 w391 w400 _]
                      tunnel: w349 -> [w362 w370 w378 w385 w392 _]
                      tunnel: w360 -> [w368 w376 w383 w388 w399 _]
                      tunnel: w359 -> [w364 w373 w380 w387 w395 w401]
                      tunnel: [w363 w371 w379 w386 w394 w401] -> w358
                      frame "boolean" {
                        n78 = Variant To Data(type=TRUE, Variant=w368) -> (data=w366:bool)  [unwired: 1 in, 1 out]
                        n79 = call-poly <vilib>:"Write Key.vi"("section"=w365, "value"=w366, "key"=w362, "refnum"=w364) -> ("refnum out"=w363:T21)  [unwired: 1 in, 6 out]
                      }
                      frame "double" {
                        n80 = Variant To Data(type=0.0 ("Signal"), Variant=w376) -> (data=w375:dbl)  [unwired: 1 in, 1 out]
                        n81 = call-poly <vilib>:"Write Key.vi"("format (fractional)"=T6."engineering", "precision (6)"=i16 3, "section"=w374, "value"=w375, "key"=w370, "refnum"=w373) -> ("refnum out"=w371:T21)  [unwired: 2 in, 3 out]
                      }
                      frame "int" {
                        n82 = Variant To Data(type=u16 0 ("Signal"), Variant=w383) -> (data=w382:u16)  [unwired: 1 in, 1 out]
                        n83 = call-poly <vilib>:"Write Key.vi"("section"=w381, "value"=w382, "key"=w378, "refnum"=w380) -> ("refnum out"=w379:T21)  [unwired: 1 in, 6 out]
                      }
                      frame "string" {
                        n84 = Variant To Data(type="", Variant=w388) -> (data=w389:string)  [unwired: 1 in, 1 out]
                        n85 = call-poly <vilib>:"Write Key.vi"("section"=w391, "value"=w389, "key"=w385, "refnum"=w387) -> ("refnum out"=w386:T21)  [unwired: 2 in, 5 out]
                      }
                      frame "enum" {
                        n86 = Variant To Data(type=T7."..." ("Signal"), Variant=w399) -> (data=w397:T7)  [unwired: 1 in, 1 out]
                        n87 = Format Into String(format string="%s", w397) -> (resulting string=w393:string)  [unwired: 2 in, 1 out]
                        n88 = call-poly <vilib>:"Write Key.vi"("section"=w400, "value"=w393, "key"=w392, "refnum"=w395) -> ("refnum out"=w394:T21)  [unwired: 2 in, 5 out]
                      }
                      frame Default {
                      }
                    }
                  }
                }
              }
              frame #1 {
                # "NOT TAKEN INTO ACCOUNT THE DC MOTOR TYPE"
                n89 = property on="Step Up" class="Enum (strict)"() -> ("Strings []"=w418:string[], "Value"=w417:enum16{"Z+", "Z-"})  [unwired: 2 in, 2 out]
                n90 = property on="Type" class="Enum (strict)"() -> ("Strings []"=w420:string[], "Value"=w421:T3)  [unwired: 2 in, 2 out]
                n91 = property on="Slow" class="Bool (strict)"() -> ("Value"=w430:bool)  [unwired: 2 in, 2 out]
                n92 = property on="Ztreshold" class="DigNum (strict)"() -> ("Value"=w428:dbl)  [unwired: 2 in, 2 out]
                n93 = property on="zMoveTresh" class="DigNum (strict)"() -> ("Value"=w429:fxp<+/-,29,2>)  [unwired: 2 in, 2 out]
                n94 = property on="Withdraw/landed" class="Bool (strict)"() -> ("Value"=w435:bool)  [unwired: 2 in, 2 out]
                n95 = property on="Beep / finished" class="Bool (strict)"() -> ("Value"=w434:bool)  [unwired: 2 in, 2 out]
                n96 = Index Array(array=w418, index=w417) -> (element=w416:string)
                n97 = Index Array(array=w420, index=w421) -> (element=w419:string)
                n98 = To Variant(anything=w435) -> (Variant=w438:variant)
                n99 = To Variant(anything=w434) -> (Variant=w437:variant)
                n100 = To Variant(anything=w430) -> (Variant=w427:variant)
                n101 = To Variant(anything=w428) -> (Variant=w425:variant)
                n102 = To Variant(anything=w429) -> (Variant=w426:variant)
                n103 = To Variant(anything=w416) -> (Variant=w436:variant)
                n104 = To Variant(anything=w419) -> (Variant=w439:variant)
                n105 = Build Array(w439, w436, w438, w437, w427, w425, w426) -> (w433:variant[])
                n106 = for {
                  tunnel: w431 -> [w452]
                  tunnel: w433 -> [w451] mode=indexing
                  tunnel: w440 -> [w450]
                  tunnel: [w449] -> _
                  tunnel: "Motor." -> [w448]
                  tunnel: string[][] [["Type", "string"], ["Step Up", "string"], ["Auto withdraw", "boolean"], ["Beep / finished", "boolean"], ["Fast", "boolean"], ["Ztreshold", "double"], ["zMoveTreshold", "double"]] ("appended array") -> [w447]
                  tunnel: 0 ("disabled index (col)") -> [w444]
                  tunnel: 1 ("disabled index (col)") -> [w443]
                  i -> [w446]
                  n107 = Index Array(array=w447, index (row) #1=w446, index (col) #1=w444, index (row) #2=w446, index (col) #2=w443) -> (element #1=w442:string, element #2=w445:string)
                  n108 = Concatenate Strings(w448, w442) -> (w441:string)
                  n109 = case shown="\"boolean\"" w445 {
                    tunnel: w452 -> [w456 w465 w472 w482 w492 _]
                    tunnel: w441 -> [w453 w461 w469 w476 w485 _]
                    tunnel: w451 -> [w459 w467 w474 w479 w491 _]
                    tunnel: w450 -> [w455 w464 w471 w478 w488 w493]
                    tunnel: [w454 w462 w470 w477 w487 w493] -> w449
                    frame "boolean" {
                      n110 = Variant To Data(type=TRUE, Variant=w459) -> (data=w457:bool)  [unwired: 1 in, 1 out]
                      n111 = call-poly <vilib>:"Write Key.vi"("section"=w456, "value"=w457, "key"=w453, "refnum"=w455) -> ("refnum out"=w454:T21)  [unwired: 1 in, 6 out]
                    }
                    frame "double" {
                      n112 = Variant To Data(type=0.0 ("Signal"), Variant=w467) -> (data=w466:dbl)  [unwired: 1 in, 1 out]
                      n113 = call-poly <vilib>:"Write Key.vi"("format (fractional)"=T6."engineering", "precision (6)"=i16 3, "section"=w465, "value"=w466, "key"=w461, "refnum"=w464) -> ("refnum out"=w462:T21)  [unwired: 2 in, 3 out]
                    }
                    frame "int" {
                      n114 = Variant To Data(type=u16 0 ("Signal"), Variant=w474) -> (data=w473:u16)  [unwired: 1 in, 1 out]
                      n115 = call-poly <vilib>:"Write Key.vi"("section"=w472, "value"=w473, "key"=w469, "refnum"=w471) -> ("refnum out"=w470:T21)  [unwired: 1 in, 6 out]
                    }
                    frame "string" {
                      n116 = Variant To Data(type="", Variant=w479) -> (data=w480:string)  [unwired: 1 in, 1 out]
                      n117 = call-poly <vilib>:"Write Key.vi"("section"=w482, "value"=w480, "key"=w476, "refnum"=w478) -> ("refnum out"=w477:T21)  [unwired: 2 in, 5 out]
                    }
                    frame "enum" {
                      n118 = Variant To Data(type=enum16{""}."" ("Type"), Variant=w491) -> (data=w490:enum16{""}, error out=w483:errorcluster)  [unwired: 1 in]
                      n119 = Format Into String(format string="%s", error in=w483, w490) -> (resulting string=w486:string)  [unwired: 1 in, 1 out]
                      n120 = call-poly <vilib>:"Write Key.vi"("section"=w492, "value"=w486, "key"=w485, "refnum"=w488) -> ("refnum out"=w487:T21)  [unwired: 2 in, 5 out]
                    }
                    frame Default {
                    }
                  }
                }
              }
            }
            n121 = call <vilib>:"Close Config Data.vi"("refnum"=w270) -> ("error out"=w269:errorcluster)  [unwired: 2 in, 8 out]
          }
          frame "Configuration.Read" {
            w499 = "Z-Controller"  # Section
            n122 = Variant To Data(error in=w501, type=path "" ("appended path"), Variant=w500) -> (data=w498:path, error out=w495:errorcluster)
            n123 = call <vilib>:"Open Config Data.vi"("error in (no error)"=w495, "configuration file path"=w498) -> ("error out"=w496:errorcluster, "refnum"=w497:T21)  [unwired: 1 in, 7 out]
            n124 = stacked-sequence {
              tunnel: [w524 _] -> w504
              tunnel: w496 -> [w508 _]
              tunnel: w497 -> [w531 w616]
              tunnel: w499 -> [w512 w615]
              frame #0 {
                w517 = 3  # Nomber of modes
                n125 = call-poly <vilib>:"Read Key.vi"("section"=w512, "error in (no error)"=w508, "key"="liftHeight", "refnum"=w531) -> ("error out"=w514:errorcluster, "value"=w523:dbl, "refnum out"=w527:T21)  [unwired: 4 in, 1 out]
                n126 = call-poly <vilib>:"Read Key.vi"("section"=w512, "error in (no error)"=w514, "key"="move wave size", "refnum"=w527) -> ("error out"=w510:errorcluster, "value"=w515:u32, "refnum out"=w530:T21)  [unwired: 4 in, 1 out]
                n127 = call-poly <vilib>:"Read Key.vi"("section"=w512, "error in (no error)"=w510, "key"="invertHeight", "refnum"=w530) -> ("error out"=w528:errorcluster, "value"=w511:bool, "refnum out"=w529:T21)  [unwired: 4 in, 1 out]
                n128 = property on="InvertHeight" class="Bool (strict)"("Value"=w511) -> ()  [unwired: 2 in, 2 out]
                n129 = property on="WaveSize" class="DigNum (strict)"("Value"=w515) -> ()  [unwired: 2 in, 2 out]
                n130 = property on="liftHeight" class="DigNum (strict)"("Value"=w523) -> ()  [unwired: 2 in, 2 out]
                n131 = for {
                  tunnel: w512 -> [w538]
                  tunnel: w529 -> [w537]
                  tunnel: w528 -> [w536]
                  tunnel: string[] ["manual move decimation", "withdraw decimation"] -> [w535] mode=indexing
                  tunnel: [w534] -> _
                  tunnel: [w533] -> w509
                  tunnel: [w532] -> w521 mode=indexing
                  n132 = call-poly <vilib>:"Read Key.vi"("section"=w538, "error in (no error)"=w536, "key"=w535, "refnum"=w537) -> ("error out"=w534:errorcluster, "value"=w532:u32, "refnum out"=w533:T21)  [unwired: 4 in, 1 out]
                }
                n133 = Index Array(array=w521) -> (element #1=w519:u32, element #2=w518:u32)  [unwired: 2 in]
                n134 = for {
                  N: w517 -> [w547]
                  tunnel: string[][] [[": Name", "string"], [": Controller on/off", "boolean"], [": Integral: value", "double"], [": Proportional: value", "double"], [": Setpoint", "double"]] ("appended array") -> [w553]
                  tunnel: w512 -> [w549]
                  tunnel: w509 -> [w554]
                  tunnel: [w552] -> w524
                  i -> [w548]
                  stop <- w544 stop-if-true
                  w543 = "controller."
                  n135 = Number To Decimal String(number=w548) -> (decimal integer string=w542:string)  [unwired: 1 in]
                  n136 = Index Array(array=w553, index (row)=1 ("y"), index (col)=0 ("disabled index (col)")) -> (element=w546:string)
                  n137 = Concatenate Strings(w543, w542, w546) -> (w545:string)
                  n138 = call-poly <vilib>:"Read Key.vi"("section"=w549, "key"=w545, "refnum"=w554) -> ("value"=w540:bool, "refnum out"=w555:T21)  [unwired: 5 in, 2 out]
                  n139 = Equal?(x=w540, y=TRUE) -> (x = y?=w544:bool)
                  n140 = case shown="True" w544 {
                    tunnel: [w556 w571] -> w552
                    tunnel: w549 -> [_ w570]
                    tunnel: w555 -> [w556 w569]
                    tunnel: w548 -> [_ w568]
                    tunnel: w547 -> [_ w566]
                    tunnel: w543 -> [_ w565]
                    tunnel: w542 -> [_ w564]
                    tunnel: w553 -> [_ w563]
                    tunnel: 2 ("y") -> [_ w562]
                    frame False {
                    }
                    frame True {
                      n141 = property on="Mode" class="Enum (strict)"("Value"=w568) -> ()  [unwired: 2 in, 2 out]
                      n142 = for {
                        N: w566 -> [_]
                        tunnel: w570 -> [w584]
                        tunnel: w569 -> [w583]
                        tunnel: [w582] -> w571
                        tunnel: [w581] -> w567 mode=indexing
                        tunnel: w565 -> [w580]
                        tunnel: w564 -> [w579]
                        tunnel: w563 -> [w577]
                        tunnel: w562 -> [w576]
                        i -> [w575]
                        n143 = Add(x=w575, y=w576) -> (x+y=w574:i32)
                        n144 = Index Array(array=w577, index (row)=w574, index (col)=0 ("disabled index (col)")) -> (element=w578:string)
                        n145 = Concatenate Strings(w580, w579, w578) -> (w572:string)
                        n146 = call-poly <vilib>:"Read Key.vi"("section"=w584, "key"=w572, "refnum"=w583) -> ("value"=w581:dbl, "refnum out"=w582:T21)  [unwired: 5 in, 2 out]
                      }
                      n147 = Index Array(array=w567) -> (element #1=w560:dbl, element #2=w558:dbl, element #3=w557:dbl)  [unwired: 3 in]
                      n148 = property on="PID" class="Clust (strict)"() -> ("Value"=w561:T1)  [unwired: 2 in, 2 out]
                      n149 = Bundle By Name(cluster=w561, "I Gain"=w560, "P Gain"=w558, "Setpoint"=w557) -> (w559:T1)
                      n150 = property on="PID" class="Clust (strict)"("Value"=w559) -> ()  [unwired: 2 in, 2 out]
                    }
                  }
                }
                n151 = Bundle("value"=w519, "value"=w518) -> (w520:cluster{"value":u32, "value":u32})  [unwired: 1 in]
                n152 = property on="Decimations" class="Clust (strict)"("Value"=w520) -> ()  [unwired: 2 in, 2 out]
              }
              frame #1 {
                w602 = TRUE
                w612 = ""
                w587 = string[][] [["Type", "string"], ["Step Up", "string"], ["Auto withdraw", "boolean"], ["Beep / finished", "boolean"], ["Fast", "boolean"], ["Ztreshold", "double"], ["zMoveTreshold", "double"]] ("appended array")
                n153 = Array Size(array=w587) -> (size(s)=w586:i32[])
                n154 = Index Array(array=w586) -> (element=w585:i32)  [unwired: 1 in]
                n155 = for {
                  N: w585 -> [_]
                  tunnel: w615 -> [w620]
                  tunnel: w616 -> [w624]
                  tunnel: "Motor." -> [w630]
                  tunnel: w587 -> [w629]
                  tunnel: 0 ("disabled index (col)") -> [w627]
                  tunnel: 1 ("disabled index (col)") -> [w626]
                  tunnel: [w621] -> w594 mode=indexing
                  i -> [w628]
                  n156 = Index Array(array=w629, index (row) #1=w628, index (col) #1=w627, index (row) #2=w628, index (col) #2=w626) -> (element #1=w625:string, element #2=w622:string)
                  n157 = Concatenate Strings(w630, w625) -> (w623:string)
                  n158 = case shown="\"boolean\"" w622 {
                    tunnel: w624 -> [w635 w640 w645]
                    tunnel: w623 -> [w634 w639 w644]
                    tunnel: [w632 w636 w641] -> w621
                    tunnel: w620 -> [w631 w638 w643]
                    frame "string", Default {
                      n159 = call-poly <vilib>:"Read Key.vi"("section"=w631, "key"=w634, "refnum"=w635) -> ("value"=w633:string)  [unwired: 5 in, 3 out]
                      n160 = To Variant(anything=w633) -> (Variant=w632:variant)
                    }
                    frame "double" {
                      n161 = call-poly <vilib>:"Read Key.vi"("section"=w638, "key"=w639, "refnum"=w640) -> ("value"=w637:dbl)  [unwired: 5 in, 3 out]
                      n162 = To Variant(anything=w637) -> (Variant=w636:variant)
                    }
                    frame "boolean" {
                      n163 = call-poly <vilib>:"Read Key.vi"("section"=w643, "key"=w644, "refnum"=w645) -> ("value"=w642:bool)  [unwired: 5 in, 3 out]
                      n164 = To Variant(anything=w642) -> (Variant=w641:variant)
                    }
                  }
                }
                n165 = Index Array(array=w594) -> (element #1=w614:variant, element #2=w613:variant)  [unwired: 2 in]
                n166 = Index Array(array=w594, index #1=2 ("index"), index #2=3 ("index"), index #3=4 ("index")) -> (element #1=w603:variant, element #2=w601:variant, element #3=w600:variant)
                n167 = Index Array(array=w594, index #1=5 ("index"), index #2=6 ("index")) -> (element #1=w590:variant, element #2=w591:variant)
                n168 = property on="Type" class="Enum (strict)"() -> ("Strings []"=w609:string[])  [unwired: 2 in, 2 out]
                n169 = Variant To Data(type=w612, Variant=w614) -> (data=w611:string)  [unwired: 1 in, 1 out]
                n170 = Variant To Data(type=w612, Variant=w613) -> (data=w608:string)  [unwired: 1 in, 1 out]
                n171 = Variant To Data(type=w602, Variant=w603) -> (data=w599:bool)  [unwired: 1 in, 1 out]
                n172 = Variant To Data(type=w602, Variant=w601) -> (data=w598:bool)  [unwired: 1 in, 1 out]
                n173 = Variant To Data(type=w602, Variant=w600) -> (data=w597:bool)  [unwired: 1 in, 1 out]
                n174 = Variant To Data(type=fxp<+/-,29,2> 0.0 ("zMoveTresh"), Variant=w591) -> (data=w589:fxp<+/-,29,2>)  [unwired: 1 in, 1 out]
                n175 = Variant To Data(type=0.0 ("Ztreshold"), Variant=w590) -> (data=w588:dbl)  [unwired: 1 in, 1 out]
                n176 = Search 1D Array(1D array=w609, element=w611) -> (index of element=w610:i32)  [unwired: 1 in]
                n177 = Search 1D Array(1D array=w609, element=w608) -> (index of element=w607:i32)  [unwired: 1 in]
                n178 = property on="Step Up" class="Enum (strict)"("Value"=w607) -> ()  [unwired: 2 in, 2 out]
                n179 = property on="Withdraw/landed" class="Bool (strict)"("Value"=w599) -> ()  [unwired: 2 in, 2 out]
                n180 = property on="Beep / finished" class="Bool (strict)"("Value"=w598) -> ()  [unwired: 2 in, 2 out]
                n181 = property on="Slow" class="Bool (strict)"("Value"=w597) -> ()  [unwired: 2 in, 2 out]
                n182 = property on="Ztreshold" class="DigNum (strict)"("Value"=w588) -> ()  [unwired: 2 in, 2 out]
                n183 = property on="zMoveTresh" class="DigNum (strict)"("Value"=w589) -> ()  [unwired: 2 in, 2 out]
                n184 = property on="Type" class="Enum (strict)"("Value"=w610) -> ()  [unwired: 2 in, 2 out]
              }
            }
            n185 = call <vilib>:"Close Config Data.vi"("refnum"=w504) -> ("error out"=w503:errorcluster)  [unwired: 2 in, 8 out]
          }
          frame "FPGA.Initialize" {
            # "Withdraw"
            # "Scanner Time constant Init"
            # "Initializes the memories for the step Motor Drive"
            n186 = local read "IO Frequency"() -> (w647:u32)
            n187 = To Variant(anything=w647) -> (Variant=w646:variant)
            n188 = call "Enqueue Message.vi"("error in"=w659, "Data"=w646, "Message"="Controllers.IOFrequency", "Queue"=w682) -> ("error out"=w650:errorcluster)  [unwired: 6 in, 1 out]
            n189 = call "FGVfpgaAdressScanEngine.vi"("Enum"=Enum."Read", "error in"=w650, "FPGA.SEin"=w651) -> ("error out"=w649:errorcluster, "FPGA.SEout"=w652:T25, "voltageRange(+/-)Out"=w648:dbl)  [unwired: 4 in, 2 out]
            n190 = call "FGVCalibrations.vi"("Enum"=Enum."Read") -> ("calibOut"=w668:T22)  [unwired: 9 in, 1 out]
            n191 = Unbundle(w668) -> ("calibParameters"=w666:T23, "calibIndex"=w665:i32)  [unwired: 1 out]
            n192 = Index Array(array=w666, index=w665) -> (element=w669:T24)
            n193 = Unbundle By Name(w669) -> ("Range.Range Z"=w664:dbl)
            n194 = call "StateMachineInit.vi"("Enum"=EnumSM."Init.StepMotor", "Error In"=w649, "FPGA.SEin"=w652, "FPGA.FBin"=w671) -> ("error out"=w673:errorcluster, "FPGA.SEout"=w661:T25, "FPGA.FBout"=w670:T4)  [unwired: 5 in]
            n195 = Bundle By Name(cluster=T9 {"enableManualMotion"=FALSE, "doMove"=FALSE, "integratorTarget"=-1.0, "clocks"={"inverseDecimation"=0.0009999275207519531, "decimation"=100, "waveSize"=100, "pixelDecimation"=0}} ("fb.mot.p.params"), "enableManualMotion"=TRUE, "doMove"=TRUE, "clocks"=T8 {"inverseDecimation"=0.09999990463256836, "decimation"=1, "waveSize"=50, "pixelDecimation"=0}) -> (w657:T9)
            n196 = xnode "Read/Write Control"("FPGA VI Reference In"=w670, "error in"=w673, "fb.mot.p.params"=w657, "fb.p.enable"=TRUE, "flt.bypass1"=bool[] [TRUE, TRUE, TRUE, TRUE, TRUE, TRUE, TRUE, TRUE] ("sosBypass"), "flt.bypass2"=bool[] [TRUE, TRUE, TRUE, TRUE], "aio.o.invertHeight"="InvertHeight", "flt.bypassPI"=FALSE, "flt.i.bypassSource"=u8 0) -> ("FPGA VI Reference Out"=w681:T4, "error out"=w677:errorcluster)
            n197 = call "FGVScannerConfig.vi"("Enum"=Enum."Init", "error in"=w677) -> ("error out"=w676:errorcluster)  [unwired: 7 in, 2 out]
          }
          frame "ZRange.Calibration" {
            # "There is duplicated code here, sorry"
            n198 = call "FGVCalibrations.vi"("Enum"=Enum."Read") -> ("calibOut"=w693:T22)  [unwired: 9 in, 1 out]
            n199 = Unbundle(w693) -> ("calibParameters"=w691:T23, "calibIndex"=w690:i32)  [unwired: 1 out]
            n200 = Index Array(array=w691, index=w690) -> (element=w694:T24)
            n201 = Unbundle By Name(w694) -> ("Range.Range Z"=w683:dbl)
            n202 = Divide(x=w683, y=2.0) -> (x/y=w685:dbl)
            n203 = control-ref of="Z (m)"() -> (w689:refnum<vi>)
            n204 = Negate(x=w685) -> (-x=w686:dbl)
            n205 = property class="Slide (strict)"(reference=w689, "Scale.Maximum"=w685, "Scale.Minimum"=w686, "Scale.FormatString"="%#.2p", "Scale.Flipped"=TRUE) -> ()  [unwired: 1 in, 2 out]
          }
          frame "Mode.Initialize" {
            w723 = u8 0 items=["process Variable", "SICM"] ("flt.i.bypassSource")
            w704 = u8 0 items=["PID/ORT", "SICM"] ("hdt.mainOutStreamSelect")
            # "0.5"
            # "1.80"
            # "Open the DataAcquisitionVI corresponding to the Controller mode:\nDataAcquisition.vi: ORT (Fit the Data for the mechanical properties)\nDataAcquisitionAux.vi: Contact, and Aux"
            # "hdt main outstream select"
            n206 = xnode "Read/Write Control"("FPGA VI Reference In"=w737, "error in"=w735) -> ("FPGA VI Reference Out"=w736:T4, "error out"=w750:errorcluster, "fb.loff.p.params"=w734:T26)
            n207 = Bundle By Name(cluster=w734, "disengagePos"=fxp<+/-,22,1> -0.6999998092651367) -> (w702:T26)
            n208 = call "FGVCalibrations.vi"("Enum"=Enum."Read") -> ("calibOut"=w744:T22)  [unwired: 9 in, 1 out]
            n209 = Unbundle By Name(w744) -> ("calibParameters"=w745:T23, "calibIndex"=w746:i32)
            n210 = call "FGVpiezoLimits.vi"("Enum"=Enum."Read") -> ("PiezoLimitsOUT(1;-1)"=w700:T27)  [unwired: 9 in, 1 out]
            n211 = xnode "Read/Write Control"("FPGA VI Reference In"=w736, "error in"=w750, "fb.i.source"="Mode", "fb.p.limits"=w700, "fb.loff.p.params"=w702, "flt.bypassPI"=FALSE, "flt.i.bypassSource"=w723, "hdt.mainOutStreamSelect"=w704) -> ("FPGA VI Reference Out"=w720:T4, "error out"=w703:errorcluster)
            n212 = Index Array(array=w745, index=w746) -> (element=w747:T24)
            n213 = Unbundle By Name(w747) -> ("Range.Range Z"=w748:dbl)
            n214 = Divide(x=w748, y=2.0) -> (x/y=w739:dbl)
            n215 = disable-structure shown="Disabled" {
              frame Disabled {
                w752 = u16 5 ("Value")
                n216 = property on="Withdraw" class="DigNum (strict)"("Value"=w752) -> ()  [unwired: 2 in, 2 out]
                n217 = property on="ManualMove" class="DigNum (strict)"("Value"=w752) -> ()  [unwired: 2 in, 2 out]
              }
              frame Enabled {
              }
            }
            n218 = control-ref of="Z (m)"() -> (w749:refnum<vi>)
            n219 = Negate(x=w739) -> (-x=w740:dbl)
            n220 = property on="Type" class="Enum (strict)"(error in=w703) -> (error out=w717:errorcluster, "Value"=w718:T3)  [unwired: 1 in, 1 out]
            n221 = property class="Slide (strict)"(reference=w749, "Scale.Maximum"=w739, "Scale.Minimum"=w740, "Scale.FormatString"="%#.2p", "Scale.Flipped"=TRUE) -> ()  [unwired: 1 in, 2 out]
            n222 = Equal?(x=w718, y=enum16{"Step motor", "DC motor"}."DC motor") -> (x = y?=w715:bool)
            n223 = Not(x=w715) -> (.not. x?=w714:bool)
            n224 = call "FGVScanParameters.vi"("Enum"=Enum."Read", "error in"=w703) -> ("error out"=w709:errorcluster, "Scan Parameters Out"=w708:T11)  [unwired: 8 in]
            n225 = property on="DCVoltage" class="DigNum (strict)"(error in=w717, "Visible"=w715) -> (error out=w716:errorcluster)  [unwired: 1 in, 1 out]
            n226 = property on="ms" class="DigNum (strict)"("Visible"=w715) -> ()  [unwired: 2 in, 2 out]
            n227 = property on="Steps" class="DigNum (strict)"("Visible"=w714) -> ()  [unwired: 2 in, 2 out]
            n228 = property on="Zstep" class="DigNum (strict)"("Visible"=w714) -> ()  [unwired: 2 in, 2 out]
            n229 = disable-structure shown="Disabled" {
              frame Disabled {
                n230 = property on="Stop" class="Bool (strict)"("DisabledEnum"=T12."Disabled and Grayed Out" ("Disabled")) -> ()  [unwired: 2 in, 2 out]
              }
              frame Enabled {
              }
            }
            n231 = Equal?(x=w708, y=T11 {"Width"=0.0, "Height"=0.0, "X Offset"=0.0, "Y Offset"=0.0, "Angle"=0.0, "Pixels/Line"=0, "Lines"=0, "Time/Line"=0.0, "Scan Rate"=0.0} ("Scan Parameters Out")) -> (x = y?=w706:T28)
            n232 = Unbundle By Name(w706) -> ("Width"=w705:bool)
            n233 = case shown="True" w705 {
              tunnel: [w754 w756] -> w711
              tunnel: w709 -> [w754 w755]
              frame False {
              }
              frame True {
                w758 = Enum."Init" ("Enum")
                n234 = call "FGVScanParameters.vi"("Enum"=w758, "error in"=w755) -> ("error out"=w757:errorcluster)  [unwired: 8 in, 1 out]
                n235 = call "FGVChannels.vi"("Enum"=w758, "error in"=w757) -> ("error out"=w756:errorcluster)  [unwired: 5 in, 4 out]
              }
            }
            n236 = call "bangBangMove.vi"("numRoundingPts"=u16 8, "numPts"="WaveSize") -> ("roundedHalfTriangle"=w731:dbl[])  [unwired: 9 in]
            n237 = To Double Precision Float(number=u16 1 ("numRoundingPts")) -> (double precision float=w724:dbl)
            n238 = Build Array (concatenate)(w731, w724) -> (w727:dbl[])
            n239 = call "StateMachineInit.vi"("ManualMotionWaveform"=w727, "Enum"=EnumSM."Init.FeedbackMotion", "Error In"=w716, "FPGA.FBin"=w720) -> ("error out"=w725:errorcluster, "FPGA.FBout"=w726:T4)  [unwired: 5 in, 1 out]
            n240 = call "FGVImageArray.vi"("Enum"=Enum."Init", "error in"=w711) -> ()  [unwired: 8 in, 2 out]
          }
          frame "DataAcquisition.Initialize" {
            w761 = u8 2 items=["Contact Mode", "ORT", "Aux"] ("fb.i.source")
            w771 = "FrontPanel\\subVIs\\DataAcquisition.vi"
            w770 = "FrontPanel\\subVIs\\DataAcquisitionAux.vi"
            n241 = xnode "Read/Write Control"("FPGA VI Reference In"=w764, "error in"=w766) -> ("FPGA VI Reference Out"=w763:T4, "error out"=w765:errorcluster, "fb.i.source"=w762:u8)
            n242 = Not Equal?(x=w762, y=w761) -> (x != y?=w759:bool)
            n243 = Select(t=w771, s=w759, f=w770) -> (s? t:f=w773:string)
            n244 = call "DataAcquisitionOpenClose.vi"("error in (no error)"=w765, "FilePath (Data Acquisition)"=w773, "Open = true // Close = False"=FALSE) -> ("error out"=w774:errorcluster)  [unwired: 8 in]
            n245 = Select(t=w771, s=w759, f=w770) -> (s? t:f=w769:string)
            n246 = call "DataAcquisitionOpenClose.vi"("error in (no error)"=w774, "FilePath (Data Acquisition)"=w769, "Open = true // Close = False"=TRUE) -> ("error out"=w767:errorcluster)  [unwired: 8 in]
          }
          frame "-------- Step Motor  ---------" {
          }
          frame "StepMotor.DoSteps" {
            w793 = 0  # stepsInInit
            w794 = 20000000  # stepsLeftInInit
            w799 = i8 1  # Up
            w800 = i8 -1  # Down
            n247 = Variant To Data(error in=w808, type=refnum<vi> refnum ("CtlRef"), Variant=w809) -> (data=w806:refnum<vi>, error out=w805:errorcluster)
            n248 = property class="Bool (strict)"(reference=w806, error in=w805) -> (error out=w810:errorcluster, "Label.Text"=w788:string)  [unwired: 1 out]
            n249 = Equal?(x=w788, y="Down" ("x")) -> (x = y?=w801:bool)
            n250 = call "FGVSteps.vi"("Enum"=Enum."Read") -> ("error out"=w796:errorcluster, "stepglobalCounterOut"=w795:i32)  [unwired: 7 in, 2 out]
            n251 = Select(t=w800, s=w801, f=w799) -> (s? t:f=w791:i8)
            n252 = To Long Integer(number=w791) -> (32bit integer=w785:i32)
            n253 = Bundle(cluster=cluster{"DirectionStep":i32, "WaitForStep":bool} {"DirectionStep"=0, "WaitForStep"=TRUE}, "DirectionStep"=w785, "WaitForStep"=TRUE) -> (w790:cluster{"DirectionStep":i32, "WaitForStep":bool})
            n254 = To Variant(anything=w790) -> (Variant=w786:variant)
            n255 = call "FGVSteps.vi"("Enum"=Enum."Write", "error in"=w796, "stepsglobalCounterIn"=w795, "stepsLeftIn"=w794, "stepsIn"=w793) -> ()  [unwired: 3 in, 4 out]
            n256 = call "Enqueue Message.vi"("error in"=w810, "Data"=w786, "Message"="StepMotor.SendSteps", "Queue"=w811) -> ("error out"=w803:errorcluster)  [unwired: 6 in, 1 out]
          }
          frame "StepMotor.SendSteps" {
            # "Add AutoApproch.Piezo in the case if Approaching? is on /blue led\nand StepLeftIn =< 0 (check that the Approaching?  switches on/off at the good time)"
            # "DirectionStep:\n-1 : down\n+1 : up"
            n257 = Variant To Data(error in=w831, type=cluster{"DirectionStep":i32, "WaitForStep":bool} {"DirectionStep"=0, "WaitForStep"=TRUE} ("cluster"), Variant=w832) -> (data=w823:cluster{"DirectionStep":i32, "WaitForStep":bool}, error out=w830:errorcluster)
            n258 = Equal?(x="Step Up", y=enum16{"Z+", "Z-"}."Z+") -> (x = y?=w827:bool)
            n259 = Unbundle(w823) -> ("DirectionStep"=w818:i32, "WaitForStep"=w819:bool)
            n260 = Negate(x=w818) -> (-x=w825:i32)
            n261 = feedback-in #1(w819) -> ()
            n262 = feedback #1(TRUE ("WaitForStep")) -> (w821:bool)
            n263 = Select(t=w818, s=w827, f=w825) -> (s? t:f=w826:i32)
            n264 = And(x=w819, y=w821) -> (x .and. y?=w820:bool)
            n265 = case shown="True" w820 {
              tunnel: w833 -> [_ w847]
              tunnel: w832 -> [_ w846]
              tunnel: [w834 w845] -> w813
              tunnel: w830 -> [w835 w844]
              tunnel: w826 -> [_ w843]
              tunnel: [w835 w842] -> w824
              tunnel: w815 -> [w834 w836]
              frame False {
              }
              frame True {
                n266 = while {
                  tunnel: w843 -> [w865]
                  tunnel: [w864] -> w841
                  tunnel: [w850] -> w837
                  tunnel: w836 -> [w868]
                  tunnel: [w867] -> w845
                  tunnel: w844 -> [w866]
                  tunnel: [w863] -> w839
                  stop <- TRUE stop-if-true
                  n267 = call "FGVSteps.vi"("Enum"=Enum."Read", "error in"=w866) -> ("error out"=w860:errorcluster, "stepglobalCounterOut"=w856:i32, "stepsLeftOut"=w857:i32, "stepsOut"=w853:i32)  [unwired: 6 in]
                  n268 = case shown="-1, Default" w865 {
                    selector: w865 -> [w870 w872]
                    tunnel: [w871 w872] -> w855
                    frame -1, Default {
                      n269 = Add(x=8 ("y"), y=w870) -> (x+y=w871:i32)
                    }
                    frame 1 {
                    }
                  }
                  n270 = Quotient & Remainder(x=w853, y=8) -> (x-y*floor(x/y)=w849:i32)  [unwired: 1 out]
                  n271 = Decrement(x=w857) -> (x-1=w859:i32)
                  n272 = Subtract(x=w856, y=w865) -> (x-y=w858:i32)
                  n273 = To Byte Integer(number=w849) -> (8bit integer=w848:i8)
                  n274 = Add(x=w849, y=w855) -> (x+y=w854:i32)
                  n275 = xnode "Read/Write Control"("FPGA VI Reference In"=w868, "error in"=w860, "smd.address"=w848) -> ("FPGA VI Reference Out"=w867:T25, "error out"=w863:errorcluster)
                  n276 = call "FGVSteps.vi"("Enum"=Enum."Write", "stepsglobalCounterIn"=w858, "stepsLeftIn"=w859, "stepsIn"=w854) -> ("stepglobalCounterOut"=w850:i32, "stepsLeftOut"=w864:i32)  [unwired: 4 in, 2 out]
                }
                "Zstep" <- w837
                n277 = flat-sequence {
                  tunnel: w839 -> [w874]
                  tunnel: [w874] -> w838
                  frame #0 {
                    n278 = Wait (ms)(milliseconds to wait="Wait") -> ()  [unwired: 1 out]
                  }
                }
                n279 = Greater Than 0?(x=w841) -> (x > 0?=w840:bool)
                n280 = case shown="False" w840 {
                  tunnel: w847 -> [w883 w904]
                  tunnel: w846 -> [_ w900]
                  tunnel: w838 -> [w884 w903]
                  tunnel: [w878 w902] -> w842
                  frame False {
                    # "So more step in case \"Approaching\" is on"
                    n281 = local read "Approaching?"() -> (w881:bool)
                    n282 = property on="Stop" class="Bool (strict)"() -> ("Value"=w879:bool)  [unwired: 2 in, 2 out]
                    n283 = local read "Slow"() -> (w875:bool)
                    n284 = Not(x=w879) -> (.not. x?=w880:bool)
                    n285 = And(x=w881, y=w880) -> (x .and. y?=w882:bool)
                    n286 = case shown="True" w882 {
                      tunnel: w884 -> [w887 w898]
                      tunnel: w883 -> [_ w899]
                      tunnel: [w887 w897] -> w878
                      tunnel: [w885 FALSE ("Value")] -> w877
                      tunnel: w879 -> [w885 _]
                      tunnel: [FALSE ("Value") TRUE ("Value")] -> w876
                      tunnel: w875 -> [_ w892]
                      frame False {
                      }
                      frame True {
                        n287 = property on="Relative Setpoint" class="Bool (strict)"() -> ("Value"=w888:bool)  [unwired: 2 in, 2 out]
                        n288 = Select(t="AutoApproach.RelativePiezo" ("Message"), s=w888, f="AutoApproach.Piezo" ("Message")) -> (s? t:f=w889:string)
                        n289 = Select(t=w889, s=w892, f="AutoApproachFast.Piezo" ("Message")) -> (s? t:f=w893:string)
                        n290 = call "Enqueue Message.vi"("error in"=w898, "Message"=w893, "Queue"=w899) -> ("error out"=w897:errorcluster)  [unwired: 7 in, 1 out]
                      }
                    }
                    n291 = local write "Approaching?"(w876) -> ()
                    n292 = property on="Stop" class="Bool (strict)"("Value"=w877) -> ()  [unwired: 2 in, 2 out]
                  }
                  frame True {
                    # "No more steps to do"
                    n293 = call "Enqueue Message.vi"("error in"=w903, "Data"=w900, "Message"="StepMotor.SendSteps", "Queue"=w904) -> ("error out"=w902:errorcluster)  [unwired: 6 in, 1 out]
                  }
                }
              }
            }
          }
          frame "StepMotor.StopSteps" {
            w914 = FALSE  # WaitForStep
            w915 = 0  # DirectionStep
            # "Send 0 steps to do (setting left steps to -1)"
            n294 = Bundle(cluster=cluster{"DirectionStep":i32, "WaitForStep":bool} {"DirectionStep"=0, "WaitForStep"=FALSE}, "DirectionStep"=w915, "WaitForStep"=w914) -> (w913:cluster{"DirectionStep":i32, "WaitForStep":bool})
            n295 = To Variant(anything=w913) -> (Variant=w908:variant)
            n296 = call "Enqueue Message.vi"("Prioritary message"=TRUE ("Message prioritaire ? (F)"), "error in"=w925, "Data"=w908, "Message"="StepMotor.SendSteps", "Queue"=w923) -> ("error out"=w911:errorcluster)  [unwired: 5 in, 1 out]
            n297 = call "FGVSteps.vi"("Enum"=Enum."Read", "error in"=w911) -> ("error out"=w924:errorcluster, "stepglobalCounterOut"=w909:i32, "stepsOut"=w916:i32)  [unwired: 6 in, 1 out]
            n298 = call "FGVSteps.vi"("Enum"=Enum."Write", "error in"=w924, "stepsglobalCounterIn"=w909, "stepsLeftIn"=-1, "stepsIn"=w916) -> ("error out"=w910:errorcluster)  [unwired: 3 in, 3 out]
          }
          frame "---------- DCMotor ----------" {
          }
          frame "DCMotor.SendVoltage" {
            w949 = i16[] [0, 85, 170, 255, 340, 425, 510, 595, 680, 765, 850, 935, 1020, 1105, 1189, 1274, 1359, 1444, 1529, 1614, 1699, 1784, 1869, 1954, 2039, 2124, 2209, 2294, 2379, 2464, 2549, 2634, 2719, 2804, 2889, 2974, 3059, 3144, 3229, 3314, 3399, 3483, 3568, 3653, 3738, 3823, 3908, 3993, 4078, 4163, 4248, 4333, 4418, 4503, 4588, 4673, 4758, 4843, 4928, 5013, 5098, 5183, 5268, 5353, 5438, 5523, 5608, 5693, 5777, 5862, 5947, 6032, 6117, 6202, 6287, 6372, 6457, 6542, 6627, 6712, 6797, 6882, 6967, 7052, 7137, 7222, 7307, 7392, 7477, 7562, 7647, 7732, 7817, 7902, 7987, 8071, 8156, 8241, 8326, 8411, 8496, 8581, 8666, 8751, 8836, 8921, 9006, 9091, 9176, 9261, 9346, 9431, 9516, 9601, 9686, 9771, 9856, 9941, 10026, 10111, 10196, 10280, 10365, 10450, 10535, 10620, 10705, 10790, 10875, 10960, 11045, 11130, 11215, 11300, 11385, 11470, 11555, 11640, 11725, 11810, 11895, 11980, 12065, 12150, 12235, 12320, 12405, 12490, 12574, 12659, 12744, 12829, 12914, 12999, 13084, 13169, 13254, 13339, 13424, 13509, 13594, 13679, 13764, 13849, 13934, 14019, 14104, 14189, 14274, 14359, 14444, 14529, 14614, 14699, 14784, 14868, 14953, 15038, 15123, 15208, 15293, 15378, 15463, 15548, 15633, 15718, 15803, 15888, 15973, 16058, 16143, 16228, 16313, 16398, 16483, 16568, 16653, 16738, 16823, 16908, 16993, 17078, 17162, 17247, 17332, 17417, 17502, 17587, 17672, 17757, 17842, 17927, 18012, 18097, 18182, 18267, 18352, 18437, 18522, 18607, 18692, 18777, 18862, 18947, 19032, 19117, 19202, 19287, 19372, 19456, 19541, 19626, 19711, 19796, 19881, 19966, 20051, 20136, 20221, 20306, 20391, 20476, 20561, 20646, 20731, 20816, 20901, 20986, 21071, 21156, 21241, 21326, 21411, 21496, 21581, 21666, 21750, 21835, 21920, 22005, 22090, 22175, 22260, 22345, 22430, 22515, 22600, 22685, 22770, 22855, 22940, 23025, 23110, 23195, 23280, 23365, 23450, 23535, 23620, 23705, 23790, 23875, 23960, 24044, 24129, 24214, 24299, 24384, 24469, 24554, 24639, 24724, 24809, 24894, 24979, 25064, 25149, 25234, 25319, 25404, 25489, 25574, 25659, 25744, 25829, 25914, 25999, 26084, 26169, 26254, 26338, 26423, 26508, 26593, 26678, 26763, 26848, 26933, 27018, 27103, 27188, 27273, 27358, 27443, 27528, 27613, 27698, 27783, 27868, 27953, 28038, 28123, 28208, 28293, 28378, 28463, 28548, 28632, 28717, 28802, 28887, 28972, 29057, 29142, 29227, 29312, 29397, 29482, 29567, 29652, 29737, 29822, 29907, 29992, 30077, 30162, 30247, 30332, 30417, 30502, 30587, 30672, 30757, 30841, 30926, 31011, 31096, 31181, 31266, 31351, 31436, 31521, 31606, 31691, 31776, 31861, 31946, 32031, 32116, 32201, 32286, 32371, 32456, 32541, 32626, 32711, 32767, 32767, 32767, 32767, 32767, 32767, 32767, 32767, 32767, 32767, 32767, 32767, 32767, 32767, 32767, 32767, 32767, 32767, 32767, 32767, 32767, 32767, 32767, 32767, 32767, 32767, 32767, 32767, 32767, 32767, 32767, 32767, 32767, 32767, 32767, 32767, 32767, 32767, 32767, 32767, 32767, 32767, 32767, 32767, 32767, 32767, 32767, 32767, 32767, 32767, 32767, 32767, 32767, 32767, 32767, 32767, 32767, 32767, 32767, 32767, 32767, 32767, 32767, 32767, 32767, 32767, 32767, 32767, 32767, 32767, 32767, 32767, 32767, 32767, 32767, 32767, 32767, 32767, 32767, 32767, 32767, 32767, 32767, 32767, 32767, 32767, 32767, 32767, 32767, 32767, 32767, 32767, 32767, 32767, 32767, 32767, 32767, 32767, 32767, 32767, 32767, 32767, 32767, 32767, 32767, 32767, 32767, 32767, 32767, 32767, 32767, 32767, 32767, 32767]  # Acceleration
            n299 = Variant To Data(error in=w958, type=refnum<vi> refnum ("Up"), Variant=w957) -> (data=w955:refnum<vi>, error out=w954:errorcluster)
            n300 = property class="Bool (strict)"(reference=w955, error in=w954) -> (reference out=w951:refnum<vi>, "Label.Text"=w953:string, "Value"=w931:bool)  [unwired: 1 out]
            n301 = Subtract(x="DCVoltage", y=0.00035 ("Offset")) -> (x-y=w963:dbl)
            n302 = Multiply(x=w963, y=i16 32678) -> (x*y=w960:dbl)
            n303 = Divide(x=849.6279999999999 ("x*y"), y=w940) -> (x/y=w941:dbl)
            n304 = Divide(x=w960, y=w940) -> (x/y=w932:dbl)
            n305 = Equal?(x=w953, y="Down") -> (x = y?=w935:bool)
            n306 = Reciprocal(x=w941) -> (1/x=w942:dbl)
            n307 = while {
              tunnel: w951 -> [w1038]
              tunnel: w935 -> [w1035]
              tunnel: w950 -> [w1033]
              tunnel: [w1032] -> w948
              tunnel: [w1014] -> w947
              tunnel: w949 -> [w1030] mode=indexing
              tunnel: [w1019] -> w946
              tunnel: w942 -> [w1024]
              tunnel: w932 -> [w1023]
              tunnel: w931 -> [_]
              i -> [w1025]
              stop <- w1020 stop-if-true
              w1027 = i16 4  # ShiftPoints
              n308 = xnode "Read/Write Control"("FPGA VI Reference In"=w1033) -> ("FPGA VI Reference Out"=w1042:T25, "error out"=w1031:errorcluster, "aio.o.outputs"=w1041:i16[])  [unwired: 1 in]
              n309 = Multiply(x=w1023, y=w1024) -> (x*y=w1029:dbl)
              n310 = property class="Bool (strict)"(reference=w1038) -> (reference out=w1019:refnum<vi>, "Value"=w1037:bool)  [unwired: 1 in, 1 out]
              n311 = Negate(x=w1030) -> (-x=w1036:i16)
              n312 = To Word Integer(number=w1029) -> (16bit integer=w1026:i16)
              n313 = local read "Approaching?"() -> (w1017:bool)
              n314 = Select(t=w1030, s=w1035, f=w1036) -> (s? t:f=w1034:i16)
              n315 = Add(x=w1027, y=w1025) -> (x+y=w1028:i32)
              n316 = Greater?(x=w1028, y=w1026) -> (0:w1021:bool)
              n317 = property on="Stop" class="Bool (strict)"() -> ("Value"=w1016:bool)  [unwired: 2 in, 2 out]
              n318 = Replace Array Subset(array=w1041, new element=w1034, index=1) -> (w1040:i16[])
              n319 = Not(x=w1037) -> (.not. x?=w1022:bool)
              n320 = xnode "Read/Write Control"("FPGA VI Reference In"=w1042, "error in"=w1031, "aio.o.outputs"=w1040) -> ("FPGA VI Reference Out"=w1032:T25, "error out"=w1015:errorcluster)
              n321 = Compound Arithmetic op=OR(w1022, w1021, w1016) -> (w1020:bool)
              n322 = And(x=w1016, y=w1017) -> (x .and. y?=w1018:bool)
              n323 = case shown="True" w1018 {
                frame False {
                }
                frame True {
                  n324 = property on="Down" class="Bool (strict)"("Value"=FALSE) -> ()  [unwired: 2 in, 2 out]
                }
              }
              n325 = call "WaitError.vi"("error in (no error)"=w1015, "milliseconds to wait"="ms") -> ("error out"=w1014:errorcluster)  [unwired: 9 in]
            }
            n326 = local read "Approaching?"() -> (w933:bool)
            n327 = property on="Stop" class="Bool (strict)"() -> ("Value"=w939:bool)  [unwired: 2 in, 2 out]
            n328 = Not(x=w939) -> (.not. x?=w938:bool)
            n329 = And(x=w933, y=w938) -> (x .and. y?=w934:bool)
            n330 = while {
              tunnel: w932 -> [w991]
              tunnel: w948 -> [w993]
              tunnel: w947 -> [w980]
              tunnel: w935 -> [w989]
              tunnel: w946 -> [w987]
              tunnel: [w986] -> w945
              tunnel: [w979] -> w944
              tunnel: w940 -> [w985]
              stop <- w982 stop-if-true
              n331 = property class="Bool (strict)"(reference=w987, error in=w980) -> ("Value"=w988:bool)  [unwired: 2 out]
              n332 = xnode "Read/Write Control"("FPGA VI Reference In"=w993, "error in"=w980) -> ("FPGA VI Reference Out"=w992:T25, "error out"=w997:errorcluster, "aio.o.outputs"=w994:i16[])
              n333 = Not(x=w988) -> (.not. x?=w984:bool)
              n334 = property on="Stop" class="Bool (strict)"() -> ("Value"=w983:bool)  [unwired: 2 in, 2 out]
              n335 = local read "Approaching?"() -> (w981:bool)
              n336 = Or(x=w984, y=w983) -> (x .or. y?=w982:bool)
              n337 = case shown="True" w982 {
                tunnel: w991 -> [w1004 _]
                tunnel: [w1003 w1007] -> w990
                tunnel: w989 -> [w1002 _]
                tunnel: w985 -> [_ w1006]
                frame False {
                  n338 = Negate(x=w1004) -> (-x=w1005:dbl)
                  n339 = Select(t=w1004, s=w1002, f=w1005) -> (s? t:f=w1003:dbl)
                }
                frame True {
                  n340 = Subtract(x=0.0, y=0.00035 ("Offset")) -> (x-y=w1012:dbl)
                  n341 = Multiply(x=w1012, y=i16 32678) -> (x*y=w1008:dbl)
                  n342 = Divide(x=w1008, y=w1006) -> (x/y=w1007:dbl)
                }
              }
              n343 = Replace Array Subset(array=w994, new element=w990, index=1) -> (w995:i16[])
              n344 = xnode "Read/Write Control"("FPGA VI Reference In"=w992, "error in"=w997, "aio.o.outputs"=w995) -> ("FPGA VI Reference Out"=w986:T25, "error out"=w977:errorcluster)
              n345 = local read "Wait"() -> (w978:u32)
              n346 = call "WaitError.vi"("error in (no error)"=w977, "milliseconds to wait"=w978) -> ("error out"=w976:errorcluster)  [unwired: 9 in]
              n347 = case shown="True" w981 {
                tunnel: [w998 w1000] -> w979
                tunnel: w976 -> [w998 w999]
                frame False {
                }
                frame True {
                  n348 = property on="Down" class="Bool (strict)"(error in=w999, "Value"=FALSE) -> (error out=w1000:errorcluster)  [unwired: 1 in, 1 out]
                }
              }
            }
            n349 = case shown="True" w934 {
              tunnel: w937 -> [_ w975]
              tunnel: [FALSE TRUE] -> w936
              frame False {
              }
              frame True {
                n350 = property on="Relative Setpoint" class="Bool (strict)"() -> ("Value"=w967:bool)  [unwired: 2 in, 2 out]
                n351 = Select(t="AutoApproach.RelativePiezo" ("Message"), s=w967, f="AutoApproach.Piezo" ("Message")) -> (s? t:f=w968:string)
                n352 = local read "Slow"() -> (w972:bool)
                n353 = Select(t=w968, s=w972, f="AutoApproachFast.Piezo" ("Message")) -> (s? t:f=w974:string)
                n354 = call "Enqueue Message.vi"("Message"=w974, "Queue"=w975) -> ()  [unwired: 8 in, 2 out]
              }
            }
            n355 = local write "Approaching?"(w936) -> ()
          }
          frame "DCMotor.Stop" {
            n356 = xnode "Read/Write Control"("FPGA VI Reference In"=w1052, "error in"=w1045) -> ("FPGA VI Reference Out"=w1046:T25, "error out"=w1054:errorcluster, "aio.o.outputs"=w1057:i16[])
            n357 = Multiply(x=0.0, y=i16 32678) -> (x*y=w1049:dbl)
            n358 = Divide(x=w1049, y=w1047) -> (x/y=w1048:dbl)
            n359 = Replace Array Subset(array=w1057, new element=w1048, index=1) -> (w1056:i16[])
            n360 = xnode "Read/Write Control"("FPGA VI Reference In"=w1046, "error in"=w1054, "aio.o.outputs"=w1056) -> ("FPGA VI Reference Out"=w1051:T25, "error out"=w1053:errorcluster)
          }
          frame "-- Stepper Motor Driver Interface --" {
          }
          frame "SmdInterface.Start" {
            n361 = local read "Approaching?"() -> (w1104:bool)
            n362 = Variant To Data(error in=w1092, type=refnum<vi> refnum ("CtlRef"), Variant=w1090) -> (data=w1089:refnum<vi>, error out=w1095:errorcluster)
            n363 = property class="Bool (strict)"(reference=w1089, error in=w1095) -> (reference out=w1065:refnum<vi>, "Label.Text"=w1094:string)  [unwired: 1 out]
            n364 = property on="Wait" class="DigNum (strict)"() -> ("Value"=w1087:u32)  [unwired: 2 in, 2 out]
            n365 = property on="Steps" class="DigNum (strict)"() -> ("Value"=w1068:u32)  [unwired: 2 in, 2 out]
            n366 = Equal?(x=w1094, y="Down" ("x")) -> (x = y?=w1088:bool)
            n367 = Select(t=w1068, s=w1104, f=u32 32000) -> (s? t:f=w1066:u32)
            n368 = To Unsigned Word Integer(number=w1087) -> (unsigned 16bit integer=w1078:u16)
            n369 = To Unsigned Word Integer(number=w1066) -> (unsigned 16bit integer=w1077:u16)
            n370 = xnode "Read/Write Control"("FPGA VI Reference In"=w1097, "stepmot.enable"=TRUE, "stepmot.dir"=w1088, "stepmot.delay(ms)"=w1078, "stepmot.steps"=w1077, "stepmot.on"=TRUE) -> ("FPGA VI Reference Out"=w1070:T25, "error out"=w1073:errorcluster)  [unwired: 1 in]
            n371 = case shown="True" w1104 {
              tunnel: w1073 -> [w1108 w1116]
              tunnel: [w1105 w1115] -> w1072
              tunnel: [w1106 w1114] -> w1071
              tunnel: w1070 -> [w1106 w1113]
              tunnel: w1065 -> [w1107 _]
              frame False {
                n372 = while {
                  tunnel: w1108 -> [w1111]
                  tunnel: w1107 -> [w1112]
                  tunnel: [w1109] -> w1105
                  stop <- w1110 continue-if-true
                  n373 = property class="Bool (strict)"(reference=w1112, error in=w1111) -> (error out=w1109:errorcluster, "Value"=w1110:bool)  [unwired: 1 out]
                }
              }
              frame True {
                n374 = while {
                  tunnel: [w1124] -> w1114
                  tunnel: w1113 -> [w1123]
                  tunnel: w1116 -> [w1126]
                  tunnel: [w1125] -> w1115
                  stop <- w1120 stop-if-true
                  w1118 = FALSE
                  n375 = xnode "Read/Write Control"("FPGA VI Reference In"=w1123, "error in"=w1126) -> ("FPGA VI Reference Out"=w1124:T25, "error out"=w1125:errorcluster, "stepmot.running"=w1122:bool)
                  n376 = property on="Stop" class="Bool (strict)"() -> ("Value"=w1119:bool)  [unwired: 2 in, 2 out]
                  n377 = Not(x=w1122) -> (.not. x?=w1121:bool)
                  n378 = Select(t=w1118, s=w1119, f=w1118) -> (s? t:f=w1117:bool)
                  n379 = Or(x=w1121, y=w1119) -> (x .or. y?=w1120:bool)
                  n380 = property on="Stop" class="Bool (strict)"("Value"=w1117) -> ()  [unwired: 2 in, 2 out]
                }
              }
            }
            n381 = xnode "Read/Write Control"("FPGA VI Reference In"=w1071, "error in"=w1072, "stepmot.enable"=FALSE, "stepmot.steps"=u16 0, "stepmot.on"=FALSE) -> ("FPGA VI Reference Out"=w1102:T25, "error out"=w1069:errorcluster)
            n382 = property on="Stop" class="Bool (strict)"(error in=w1069) -> (error out=w1101:errorcluster, "Value"=w1080:bool)  [unwired: 1 in, 1 out]
            n383 = local read "Slow"() -> (w1084:bool)
            n384 = Not(x=w1080) -> (.not. x?=w1081:bool)
            n385 = And(x=w1104, y=w1081) -> (x .and. y?=w1085:bool)
            n386 = case shown="True" w1085 {
              tunnel: w1101 -> [w1129 w1140]
              tunnel: w1103 -> [_ w1141]
              tunnel: [w1129 w1139] -> w1079
              tunnel: [w1127 FALSE ("Value")] -> w1082
              tunnel: w1080 -> [w1127 _]
              tunnel: [FALSE ("Value") TRUE ("Value")] -> w1083
              tunnel: w1084 -> [_ w1134]
              frame False {
              }
              frame True {
                n387 = local read "Relative Setpoint"() -> (w1130:bool)
                n388 = Select(t="AutoApproach.RelativePiezo" ("Message"), s=w1130, f="AutoApproach.Piezo" ("Message")) -> (s? t:f=w1131:string)
                n389 = Select(t=w1131, s=w1134, f="AutoApproachFast.Piezo" ("Message")) -> (s? t:f=w1135:string)
                n390 = call "Enqueue Message.vi"("error in"=w1140, "Message"=w1135, "Queue"=w1141) -> ("error out"=w1139:errorcluster)  [unwired: 7 in, 1 out]
              }
            }
            n391 = local write "Approaching?"(w1083) -> ()
            n392 = property on="Stop" class="Bool (strict)"("Value"=w1082) -> ()  [unwired: 2 in, 2 out]
          }
          frame "SmdInterface.Stop" {
            n393 = xnode "Read/Write Control"("FPGA VI Reference In"=w1145, "error in"=w1147, "stepmot.enable"=FALSE, "stepmot.steps"=u16 0, "stepmot.on"=FALSE) -> ("FPGA VI Reference Out"=w1144:T25, "error out"=w1146:errorcluster)
          }
          frame "---- Stick-Slip ----" {
          }
          frame "StickSlip.Move" {
            n394 = Variant To Data(error in=w1185, type=refnum<vi> refnum ("CtlRef"), Variant=w1184) -> (data=w1187:refnum<vi>, error out=w1189:errorcluster)
            n395 = property class="Bool (strict)"(reference=w1187, error in=w1189) -> (reference out=w1199:refnum<vi>, error out=w1183:errorcluster, "Label.Text"=w1186:string)
            n396 = xnode "Read/Write Control"("FPGA VI Reference In"=w1166, "error in"=w1183) -> ("FPGA VI Reference Out"=w1176:T25, "error out"=w1175:errorcluster, "wfm.Parameters"=w1182:T29, "wfm.Parameters.target"=w1181:i16)
            n397 = Equal?(x=w1186, y="Up" ("x")) -> (x = y?=w1180:bool)
            n398 = Equal?(x=w1180, y=TRUE) -> (x = y?=w1193:bool)
            n399 = Greater Than 0?(x=w1181) -> (x > 0?=w1192:bool)
            n400 = Negate(x=w1181) -> (-x=w1196:i16)
            n401 = Equal?(x=w1192, y=w1193) -> (x = y?=w1195:bool)
            n402 = Select(t=w1181, s=w1195, f=w1196) -> (s? t:f=w1194:i16)
            n403 = Bundle By Name(cluster=w1182, "axis"=enum16{"none", "x", "y", "z"}."z", "target"=w1194) -> (w1177:T29)
            n404 = local read "Approaching?"() -> (w1170:bool)
            n405 = local read "Slow"() -> (w1171:bool)
            n406 = property on="Stop" class="Bool (strict)"() -> ("Value"=w1157:bool)  [unwired: 2 in, 2 out]
            n407 = xnode "Read/Write Control"("FPGA VI Reference In"=w1176, "error in"=w1175, "wfm.reset"=cluster{"rampx":bool, "ustepx":bool} {"rampx"=TRUE, "ustepx"=TRUE} ("Reset"), "wfm.Parameters"=w1177) -> ("FPGA VI Reference Out"=w1174:T25, "error out"=w1173:errorcluster)
            n408 = Not(x=w1157) -> (.not. x?=w1160:bool)
            n409 = And(x=w1170, y=w1160) -> (x .and. y?=w1172:bool)
            n410 = case shown="True" w1170 {
              tunnel: w1174 -> [w1219 w1238]
              tunnel: w1173 -> [w1218 w1237]
              tunnel: [w1216 w1235] -> w1168
              tunnel: [w1215 w1234] -> w1167
              tunnel: w1199 -> [w1217 _]
              frame False {
                n411 = while {
                  tunnel: w1219 -> [w1231]
                  tunnel: w1218 -> [w1230]
                  tunnel: w1217 -> [w1229]
                  tunnel: [w1222] -> w1216
                  tunnel: [w1221] -> w1215
                  stop <- w1220 stop-if-true
                  n412 = property class="Bool (strict)"(reference=w1229) -> ("Value"=w1228:bool)  [unwired: 1 in, 2 out]
                  n413 = property on="Stop" class="Bool (strict)"() -> ("Value"=w1227:bool)  [unwired: 2 in, 2 out]
                  n414 = xnode "Read/Write Control"("FPGA VI Reference In"=w1231, "error in"=w1230) -> ("FPGA VI Reference Out"=w1226:T25, "error out"=w1225:errorcluster, "wfm.reset"=w1224:cluster{"rampx":bool, "ustepx":bool})
                  n415 = Not(x=w1228) -> (.not. x?=w1232:bool)
                  n416 = Bundle By Name(cluster=w1224, "rampx"=w1228, "ustepx"=FALSE) -> (w1223:cluster{"rampx":bool, "ustepx":bool})
                  n417 = Compound Arithmetic op=OR(w1232, w1227) -> (w1220:bool)
                  n418 = xnode "Read/Write Control"("FPGA VI Reference In"=w1226, "error in"=w1225, "wfm.reset"=w1223) -> ("FPGA VI Reference Out"=w1222:T25, "error out"=w1221:errorcluster)
                }
              }
              frame True {
                n419 = xnode "Read/Write Control"("FPGA VI Reference In"=w1238, "error in"=w1237, "wfm.reset"=cluster{"rampx":bool, "ustepx":bool} {"rampx"=FALSE, "ustepx"=FALSE} ("Reset")) -> ("FPGA VI Reference Out"=w1239:T25, "error out"=w1240:errorcluster)
                n420 = while {
                  tunnel: w1239 -> [w1245]
                  tunnel: w1240 -> [w1244]
                  tunnel: [w1243] -> w1234
                  tunnel: [w1242] -> w1235
                  stop <- w1246 stop-if-true
                  n421 = xnode "Read/Write Control"("FPGA VI Reference In"=w1245, "error in"=w1244) -> ("FPGA VI Reference Out"=w1242:T25, "error out"=w1243:errorcluster, "wfm.Parameters.target"=w1247:i16, "wfm.rampIndex.NextRamp"=w1248:i16)
                  n422 = Wait (ms)(milliseconds to wait=u32 1) -> ()  [unwired: 1 out]
                  n423 = property on="Stop" class="Bool (strict)"() -> ("Value"=w1252:bool)  [unwired: 2 in, 2 out]
                  n424 = Absolute Value(x=w1247) -> (abs(x)=w1249:i16)
                  n425 = Absolute Value(x=w1248) -> (abs(x)=w1250:i16)
                  n426 = Equal?(x=w1249, y=w1250) -> (x = y?=w1251:bool)
                  n427 = Compound Arithmetic op=OR(w1251, w1252) -> (w1246:bool)
                }
              }
            }
            n428 = xnode "Read/Write Control"("FPGA VI Reference In"=w1168, "error in"=w1167, "wfm.reset"=cluster{"rampx":bool, "ustepx":bool} {"rampx"=TRUE, "ustepx"=TRUE} ("Reset")) -> ("FPGA VI Reference Out"=w1165:T25, "error out"=w1164:errorcluster)
            n429 = case shown="True" w1172 {
              tunnel: w1164 -> [w1202 w1213]
              tunnel: w1163 -> [_ w1214]
              tunnel: [w1202 w1212] -> w1159
              tunnel: [w1200 FALSE ("Value")] -> w1161
              tunnel: w1157 -> [w1200 _]
              tunnel: [FALSE ("Value") TRUE ("Value")] -> w1162
              tunnel: w1171 -> [_ w1207]
              frame False {
              }
              frame True {
                n430 = local read "Relative Setpoint"() -> (w1203:bool)
                n431 = Select(t="AutoApproach.RelativePiezo" ("Message"), s=w1203, f="AutoApproach.Piezo" ("Message")) -> (s? t:f=w1204:string)
                n432 = Select(t=w1204, s=w1207, f="AutoApproachFast.Piezo" ("Message")) -> (s? t:f=w1208:string)
                n433 = call "Enqueue Message.vi"("error in"=w1213, "Message"=w1208, "Queue"=w1214) -> ("error out"=w1212:errorcluster)  [unwired: 7 in, 1 out]
              }
            }
            n434 = local write "Approaching?"(w1162) -> ()
            n435 = property on="Stop" class="Bool (strict)"("Value"=w1161) -> ()  [unwired: 2 in, 2 out]
          }
          frame "StickSlip.Stop" {
            n436 = xnode "Read/Write Control"("FPGA VI Reference In"=w1256, "error in"=w1258, "wfm.reset"=cluster{"rampx":bool, "ustepx":bool} {"rampx"=TRUE, "ustepx"=TRUE} ("Reset")) -> ("FPGA VI Reference Out"=w1255:T25, "error out"=w1257:errorcluster)
          }
          frame "------------- PID -------------" {
          }
          frame "Feedback.Enable" {
            # "If turn on feedback : ManualMotion should be off\nIf feedback was on and we withdraw : then manual motion would have been turned on and piezo put to 0,\nthen the feedback should be disabled"
            n437 = Variant To Data(error in=w1285, type=TRUE, Variant=w1284) -> (data=w1269:bool, error out=w1288:errorcluster)
            n438 = xnode "Read/Write Control"("FPGA VI Reference In"=w1283, "error in"=w1288) -> ("FPGA VI Reference Out"=w1282:T4, "error out"=w1281:errorcluster, "fb.mot.p.params.enableManualMotion"=w1275:bool, "fb.mot.p.params"=w1268:T9)
            n439 = Bundle By Name(cluster=w1268, "enableManualMotion"=FALSE, "doMove"=FALSE) -> (w1276:T9)
            n440 = local read "Surface reached"() -> (w1274:bool)
            n441 = case shown="True" w1275 {
              tunnel: w1282 -> [w1295 w1297]
              tunnel: w1281 -> [w1294 w1296]
              tunnel: [w1293 w1296] -> w1280
              tunnel: [w1292 w1297] -> w1279
              tunnel: w1276 -> [w1291 _]
              frame True {
                n442 = xnode "Read/Write Control"("FPGA VI Reference In"=w1295, "error in"=w1294, "fb.mot.p.params"=w1291) -> ("FPGA VI Reference Out"=w1292:T4, "error out"=w1293:errorcluster)
              }
              frame False {
              }
            }
            n443 = case shown="False" w1274 {
              frame False {
              }
              frame True {
                n444 = local write "Surface reached"(FALSE ("Surface reached")) -> ()
                n445 = local write "Approaching?"(FALSE ("Approaching?")) -> ()
              }
            }
            n446 = xnode "Read/Write Control"("FPGA VI Reference In"=w1279, "error in"=w1280, "flt.bypassPI"=FALSE, "fb.p.enable"=w1269) -> ("FPGA VI Reference Out"=w1287:T4, "error out"=w1271:errorcluster)
            n447 = property on="Feedback On" class="Bool (strict)"(error in=w1271, "Value"=w1269) -> (error out=w1270:errorcluster)  [unwired: 1 in, 1 out]
          }
          frame "PID.Update" {
            # "Maybe connect to ref SE"
            # "In intermittent contact mode, the gains are negative"
            n448 = Variant To Data(error in=w1320, type=T1 {"Setpoint"=0.05, "P Gain"=0.0, "I Gain"=0.0003} ("PID"), Variant=w1318) -> (data=w1319:T1, error out=w1310:errorcluster)
            n449 = xnode "Read/Write Control"("FPGA VI Reference In"=w1301, "error in"=w1310) -> ("FPGA VI Reference Out"=w1300:T25, "error out"=w1328:errorcluster, "aio.s.slowVertical"=w1303:i16)
            n450 = disable-structure shown="FPGA_BUILT==RIO0" {
              disable-tunnel: [10.0 ("voltageRange(+/-)Out") w1341] -> w1298
              frame condition #0 {
              }
              frame condition #1 (active) {
                n451 = call "FGVfpgaAdress.vi"("Enum"=Enum."Read") -> ("voltageRange(+/-)Out"=w1341:dbl)  [unwired: 5 in, 5 out]
              }
            }
            n452 = local read "Relative Setpoint"() -> (w1306:bool)
            n453 = Unbundle By Name(w1319) -> ("Setpoint"=w1308:dbl, "P Gain"=w1313:dbl, "I Gain"=w1312:dbl)
            n454 = disable-structure shown="Disabled" {
              disable-tunnel: [w1337 w1339] -> w1315
              disable-tunnel: [w1336 w1338] -> w1314
              disable-tunnel: w1313 -> [w1331 w1339]
              disable-tunnel: w1312 -> [w1329 w1338]
              frame Disabled {
                n455 = property on="Mode" class="Enum (strict)"() -> ("Value"=w1335:enum16{"Contact", "OR Tapping", "Aux"})  [unwired: 2 in, 2 out]
                n456 = Equal?(x=w1335, y=T14."Intermittent Contact" ("Mode")) -> (x = y?=w1333:bool)
                n457 = Negate(x=w1331) -> (-x=w1332:dbl)
                n458 = Negate(x=w1329) -> (-x=w1330:dbl)
                n459 = Select(t=w1331, s=w1333, f=w1332) -> (s? t:f=w1337:dbl)
                n460 = Select(t=w1329, s=w1333, f=w1330) -> (s? t:f=w1336:dbl)
              }
              frame Enabled {
              }
            }
            n461 = To Double Precision Float(number=w1303) -> (double precision float=w1305:dbl)
            n462 = Scale By Power Of 2(n=i16 -15, x=w1305) -> (x*2^n=w1299:dbl)
            n463 = Compound Arithmetic op=MULTIPLY(w1298, w1299, w1308) -> (w1309:dbl)
            n464 = Select(t=w1309, s=w1306, f=w1308) -> (s? t:f=w1307:dbl)
            n465 = Divide(x=w1307, y=w1298) -> (x/y=w1316:dbl)
            n466 = To Fixed-Point(fixed-point type=fxp<+/-,17,1> 0.0 ("setPoint"), number=w1316) -> (fixed-point=w1325:fxp<+/-,17,1>)
            n467 = Bundle By Name(cluster=T13 {"setPoint"=0.0, "pGain"=0.0, "iGain"=0.0, "setPointAlt"=0.0} ("fbParams"), "setPoint"=w1325, "pGain"=w1315, "iGain"=w1314) -> (w1323:T13)
            n468 = call "PIDParameters.vi"("error in"=w1328, "fbParams"=w1323, "FPGA VI Reference In"=w1302) -> ("error out"=w1322:errorcluster, "FPGA VI Reference Out"=w1317:T4)  [unwired: 7 in]
          }
          frame "Z.Update" {
            w1353 = TRUE ("enableManualMotion")
            n469 = Bundle(cluster=T15 {"enableManualMotion"=FALSE, "doMove"=FALSE, "liftHeight"=0.0} ("output cluster"), "enableManualMotion"=w1353, "doMove"=w1353, "liftHeight"="Z (m)") -> (w1352:T15)
            n470 = To Variant(anything=w1352) -> (Variant=w1346:variant)
            n471 = call "Enqueue Message.vi"("error in"=w1355, "Data"=w1346, "Message"="Z.ManualMotion", "Queue"=w1354) -> ("error out"=w1348:errorcluster)  [unwired: 6 in, 1 out]
          }
          frame "Z.ManualMotion.Lift" {
            # "Is inverted in the case of an inverted height (FPGA controlled)"
            # "ZRange between (-Range/2) and (+Range/2)"
            # "-1..1 : piezo values"
            n472 = Variant To Data(error in=w1387, type=T15 {"enableManualMotion"=FALSE, "doMove"=FALSE, "liftHeight"=0.0} ("output cluster"), Variant=w1386) -> (data=w1385:T15, error out=w1377:errorcluster)
            n473 = Unbundle(w1385) -> ("enableManualMotion"=w1384:bool, "doMove"=w1383:bool, "liftHeight"=w1372:dbl)
            n474 = xnode "Read/Write Control"("FPGA VI Reference In"=w1382, "error in"=w1377) -> ("FPGA VI Reference Out"=w1381:T4, "error out"=w1388:errorcluster, "fb.o.height"=w1368:fxp<+/-,31,4>)
            n475 = Divide(x=w1372, y=w1364) -> (x/y=w1371:dbl)
            n476 = Multiply(x=w1371, y=2.0) -> (x*y=w1369:dbl)
            n477 = To Double Precision Float(number=w1368) -> (double precision float=w1367:dbl)
            n478 = Subtract(x=w1367, y=w1369) -> (x-y=w1357:dbl)
            n479 = In Range and Coerce(upper limit=1.0, x=w1357, lower limit=-1.0) -> (coerced(x)=w1378:dbl)  [unwired: 1 out]
            n480 = property on="ManualMove" class="DigNum (strict)"() -> ("Value"=w1359:u16)  [unwired: 2 in, 2 out]
            n481 = property on="WaveSize" class="DigNum (strict)"() -> ("Value"=w1360:u16)  [unwired: 2 in, 2 out]
            n482 = To Fixed-Point(fixed-point type=fxp<+/-,22,2> 0.0 ("integratorTarget"), number=w1378) -> (fixed-point=w1365:fxp<+/-,22,2>)
            n483 = Reciprocal(x=w1359) -> (1/x=w1358:dbl)
            n484 = Bundle By Name(cluster=T9 {"enableManualMotion"=FALSE, "doMove"=FALSE, "integratorTarget"=0.0, "clocks"={"inverseDecimation"=0.0, "decimation"=0, "waveSize"=0, "pixelDecimation"=0}} ("fb.mot.p.params"), "enableManualMotion"=w1384, "doMove"=w1383, "integratorTarget"=w1365, "clocks.decimation"=w1359, "clocks.inverseDecimation"=w1358, "clocks.waveSize"=w1360) -> (w1361:T9)
            n485 = xnode "Read/Write Control"("FPGA VI Reference In"=w1381, "error in"=w1388, "fb.mot.p.params"=w1361) -> ("FPGA VI Reference Out"=w1375:T4, "error out"=w1374:errorcluster)
            n486 = flat-sequence {
              tunnel: w1374 -> [w1389]
              tunnel: [w1389] -> w1373
              frame #0 {
                n487 = local write "Feedback On"(FALSE ("Feedback On")) -> ()
              }
            }
          }
          frame "Z.ManualMotion" {
            # "Added the 26.09.2017"
            # "-1..1 : piezo values"
            n488 = feedback #2() -> (w1407:bool)  [unwired: 1 in]
            n489 = xnode "Read/Write Control"("FPGA VI Reference In"=w1406, "error in"=w1400, "fb.p.enable"=w1407) -> ("FPGA VI Reference Out"=w1405:T4, "error out"=w1411:errorcluster, "fb.p.enable"=w1410:bool)
            n490 = Select(t=w1410, s=w1410, f=TRUE) -> (s? t:f=w1408:bool)
            n491 = feedback-in #2(w1408) -> ()
            n492 = Variant To Data(error in=w1411, type=T15 {"enableManualMotion"=FALSE, "doMove"=FALSE, "liftHeight"=0.0} ("output cluster"), Variant=w1426) -> (data=w1425:T15, error out=w1401:errorcluster)
            n493 = Unbundle(w1425) -> ("enableManualMotion"=w1424:bool, "doMove"=w1423:bool, "liftHeight"=w1417:dbl)
            n494 = Divide(x=w1417, y=w1397) -> (x/y=w1416:dbl)
            n495 = Multiply(x=w1416, y=2.0) -> (x*y=w1420:dbl)
            n496 = xnode "Read/Write Control"("FPGA VI Reference In"=w1405, "error in"=w1401) -> ("FPGA VI Reference Out"=w1404:T4, "error out"=w1403:errorcluster, "fb.mot.p.params"=w1402:T9)
            n497 = Unbundle By Name("Decimations") -> ("ManualMove"=w1393:u16)
            n498 = In Range and Coerce(upper limit=1.0, x=w1420, lower limit=-1.0) -> (coerced(x)=w1419:dbl)  [unwired: 1 out]
            n499 = property on="WaveSize" class="DigNum (strict)"() -> ("Value"=w1394:u16)  [unwired: 2 in, 2 out]
            n500 = To Fixed-Point(fixed-point type=fxp<+/-,22,2> 0.0 ("integratorTarget"), number=w1419) -> (fixed-point=w1398:fxp<+/-,22,2>)
            n501 = Reciprocal(x=w1393) -> (1/x=w1392:dbl)
            n502 = Bundle By Name(cluster=w1402, "enableManualMotion"=w1424, "doMove"=w1423, "integratorTarget"=w1398, "clocks.decimation"=w1393, "clocks.inverseDecimation"=w1392, "clocks.waveSize"=w1394) -> (w1427:T9)
            n503 = xnode "Read/Write Control"("FPGA VI Reference In"=w1404, "error in"=w1403, "fb.mot.p.params"=w1427) -> ("FPGA VI Reference Out"=w1412:T4, "error out"=w1413:errorcluster)
            n504 = flat-sequence {
              tunnel: w1413 -> [w1429]
              tunnel: [w1429] -> w1418
              frame #0 {
                w1428 = FALSE ("Feedback On")
                n505 = local write "Feedback On"(w1428) -> ()
                n506 = local write "Display Z"(w1428) -> ()
              }
            }
          }
          frame "Z.ManualMotion.Withdraw" {
            w1432 = FALSE ("Withdraw")
            n507 = flat-sequence {
              tunnel: w1459 -> [w1474]
              tunnel: [w1474] -> w1457
              frame #0 {
                "Display Z" <- TRUE ("Boolean")
              }
            }
            n508 = xnode "Read/Write Control"("FPGA VI Reference In"=w1458, "error in"=w1457) -> ("FPGA VI Reference Out"=w1455:T4, "error out"=w1456:errorcluster, "fb.mot.p.params"=w1431:T9, "fb.o.height"=w1454:fxp<+/-,31,4>, "fb.p.limits.lowerLimit"=w1438:fxp<+/-,28,4>)
            n509 = local read "WaveSize"() -> (w1443:u16)
            n510 = property on="Withdraw" class="DigNum (strict)"() -> ("Value"=w1441:u16)  [unwired: 2 in, 2 out]
            n511 = Equal?(x=w1454, y=w1438) -> (x = y?=w1430:bool)
            n512 = To Fixed-Point(fixed-point type=fxp<+/-,22,2> 0.0 ("fb.p.limits.lowerLimit"), number=w1438) -> (fixed-point=w1439:fxp<+/-,22,2>)
            n513 = Not(x=w1430) -> (.not. x?=w1436:bool)
            n514 = Reciprocal(x=w1441) -> (1/x=w1442:dbl)
            n515 = Bundle By Name(cluster=w1431, "enableManualMotion"=w1436, "doMove"=w1436, "integratorTarget"=w1439, "clocks.decimation"=w1441, "clocks.inverseDecimation"=w1442, "clocks.waveSize"=w1443) -> (w1447:T9)
            n516 = xnode "Read/Write Control"("FPGA VI Reference In"=w1455, "error in"=w1456, "fb.mot.p.params"=w1447) -> ("FPGA VI Reference Out"=w1449:T4, "error out"=w1450:errorcluster)
            n517 = case shown="False" w1430 {
              tunnel: [w1465 w1473] -> w1453
              tunnel: [w1464 w1472] -> w1448
              tunnel: w1450 -> [w1463 w1472]
              tunnel: w1449 -> [w1462 w1473]
              frame False {
                n518 = while {
                  tunnel: w1463 -> [w1471]
                  tunnel: w1462 -> [w1470]
                  tunnel: [w1469] -> w1465
                  tunnel: [w1468] -> w1464
                  stop <- w1467 stop-if-true
                  n519 = xnode "Read/Write Control"("FPGA VI Reference In"=w1470, "error in"=w1471) -> ("FPGA VI Reference Out"=w1469:T4, "error out"=w1468:errorcluster, "fb.mot.s.running"=w1466:bool)
                  n520 = Not(x=w1466) -> (.not. x?=w1467:bool)
                }
                n521 = Wait (ms)(milliseconds to wait=u32 20) -> ()  [unwired: 1 out]
              }
              frame True {
              }
            }
            n522 = Bundle By Name(cluster=w1447, "enableManualMotion"=FALSE) -> (w1440:T9)
            n523 = xnode "Read/Write Control"("FPGA VI Reference In"=w1453, "error in"=w1448, "fb.p.enable"=FALSE ("enableFeedback"), "fb.mot.p.params"=w1440) -> ("FPGA VI Reference Out"=w1460:T4, "error out"=w1435:errorcluster)
            n524 = property on="Withdraw" class="Bool (strict)"(error in=w1435, "Value"=w1432) -> (error out=w1434:errorcluster)  [unwired: 1 in, 1 out]
            n525 = property on="Feedback On" class="Bool (strict)"(error in=w1434, "Value"=w1432) -> (error out=w1433:errorcluster)  [unwired: 1 in, 1 out]
          }
          frame "WithdrawAndMove" {
            n526 = call "Enqueue Message.vi"("error in"=w1481, "Message"="Z.ManualMotion.Withdraw", "Queue"=w1486) -> ("error out"=w1479:errorcluster, "Queue dup."=w1480:refnum<queue>)  [unwired: 7 in]
            n527 = local read "Type"() -> (w1477:T3)
            n528 = case shown="\"Step motor\", Default" w1477 {
              tunnel: w1480 -> [w1504 w1514]
              tunnel: w1479 -> [w1499 w1506]
              tunnel: [w1497 w1510] -> w1485
              frame "Step motor", Default {
                w1493 = 1  # Down
                # "The step motor moves up 4 x nStep used for the auto-approach"
                n529 = call "FGVSteps.vi"("Enum"=Enum."Read", "error in"=w1499) -> ("error out"=w1505:errorcluster, "stepglobalCounterOut"=w1496:i32, "stepsOut"=w1498:i32)  [unwired: 6 in, 1 out]
                n530 = local read "Steps"() -> (w1489:u32)
                n531 = Multiply(x=w1489, y=u32 10) -> (x*y=w1488:u32)
                n532 = To Long Integer(number=w1488) -> (32bit integer=w1490:i32)
                n533 = call "FGVSteps.vi"("Enum"=Enum."Write", "error in"=w1505, "stepsglobalCounterIn"=w1496, "stepsLeftIn"=w1490, "stepsIn"=w1498) -> ("error out"=w1500:errorcluster)  [unwired: 3 in, 3 out]
                n534 = Bundle(cluster=cluster{"DirectionStep":i32, "WaitForStep":bool} {"DirectionStep"=0, "WaitForStep"=FALSE}, "DirectionStep"=w1493, "WaitForStep"=TRUE) -> (w1495:cluster{"DirectionStep":i32, "WaitForStep":bool})
                n535 = To Variant(anything=w1495) -> (Variant=w1491:variant)
                n536 = call "Enqueue Message.vi"("error in"=w1500, "Data"=w1491, "Message"="StepMotor.SendSteps", "Queue"=w1504) -> ("error out"=w1497:errorcluster)  [unwired: 6 in, 1 out]
              }
              frame "DC motor" {
                n537 = property on="Up" class="Bool (strict)"(error in=w1506, "Value"=FALSE) -> (error out=w1515:errorcluster)  [unwired: 1 in, 1 out]
                n538 = control-ref of="Up"() -> (w1512:refnum<vi>)
                n539 = call "Enqueue Message.vi"("error in"=w1515, "Data"=w1512, "Message"="DCMotor.SendVoltage", "Queue"=w1514) -> ("error out"=w1511:errorcluster, "Queue dup."=w1509:refnum<queue>)  [unwired: 6 in]
                n540 = call "Enqueue Message.vi"("error in"=w1511, "Message"="DCMotor.Stop", "Queue"=w1509) -> ("error out"=w1510:errorcluster)  [unwired: 7 in, 1 out]
              }
            }
          }
          frame "Height.Invert" {
            n541 = Variant To Data(error in=w1528, type=TRUE, Variant=w1527) -> (data=w1518:bool, error out=w1523:errorcluster)
            n542 = property on="InvertHeight" class="Bool (strict)"(error in=w1523, "Value"=w1518) -> (error out=w1522:errorcluster)  [unwired: 1 in, 1 out]
            n543 = xnode "Read/Write Control"("FPGA VI Reference In"=w1530, "error in"=w1522, "aio.o.invertHeight"=w1518) -> ("FPGA VI Reference Out"=w1529:T4, "error out"=w1520:errorcluster)
            n544 = call "IsVIRunning.vi"("error in (no error)"=w1520, "name or relative path"="FrontPanel\\Analogs.vi") -> ("error out"=w1519:errorcluster, "RunningVI?"=w1516:bool)  [unwired: 8 in]
            n545 = case shown="True" w1516 {
              tunnel: [w1532 w1535] -> w1521
              tunnel: w1519 -> [w1532 w1534]
              tunnel: w1518 -> [_ w1533]
              frame False {
              }
              frame True {
                n546 = Obtain Queue(name (unnamed)="Analogs" ("QueueName"), element data type=T16 {"Message"="", "Données de message"=variant} ("Cluster Message"), error in (no error)=w1534) -> (queue out=w1540:refnum<queue>, error out=w1541:errorcluster)  [unwired: 2 in, 1 out]
                n547 = To Variant(anything=w1533) -> (Variant=w1536:variant)
                n548 = call "Enqueue Message.vi"("error in"=w1541, "Data"=w1536, "Message"="Init.FromFGPA", "Queue"=w1540) -> ("error out"=w1535:errorcluster)  [unwired: 6 in, 1 out]
              }
            }
          }
          frame "------  AutoApproachFast  ------" {
          }
          frame "AutoApproachFast.Init" {
            # "The PID gains should be high enough to move the piezo quickly"
            n549 = call "SICMExperimentOnCheck.vi"("error in (no error)"=w1551, "Refnum in"=w1547) -> ("error out"=w1550:errorcluster, "IsExperimentSICM?"=w1549:bool, "Refnum out"=w1548:T4)  [unwired: 7 in]
            n550 = case shown="True" w1549 {
              tunnel: w1563 -> [w1568 w1579]
              tunnel: [w1567 w1579] -> w1562
              tunnel: [w1566 w1577] -> w1557
              tunnel: [w1569 w1578] -> w1552
              tunnel: w1550 -> [_ w1571]
              tunnel: w1548 -> [w1569 w1570]
              frame False {
                n551 = call "Enqueue Message.vi"("Message"="Z.ManualMotion.Withdraw", "Queue"=w1568) -> ("error out"=w1566:errorcluster, "Queue dup."=w1567:refnum<queue>)  [unwired: 8 in]
              }
              frame True {
                n552 = xnode "Read/Write Control"("FPGA VI Reference In"=w1570, "error in"=w1571) -> ("FPGA VI Reference Out"=w1575:T4, "error out"=w1576:errorcluster, "sicm.p.modes"=w1574:T30)
                n553 = Bundle By Name(cluster=w1574, "sicm.p.enable"=FALSE) -> (w1573:T30)
                n554 = xnode "Read/Write Control"("FPGA VI Reference In"=w1575, "error in"=w1576, "sicm.p.modes"=w1573) -> ("FPGA VI Reference Out"=w1578:T4, "error out"=w1577:errorcluster)
              }
            }
            n555 = local write "Approaching?"(TRUE ("Approaching?")) -> ()
            n556 = disable-structure shown="Enabled" {
              frame Disabled {
                n557 = property on="Stop" class="Bool (strict)"("DisabledEnum"=T12."Enabled" ("Disabled")) -> ()  [unwired: 2 in, 2 out]
              }
              frame Enabled {
              }
            }
            n558 = call "Enqueue Message.vi"("error in"=w1557, "Message"="AutoApproachFast.InitWatchDog", "Queue"=w1562) -> ("error out"=w1556:errorcluster, "Queue dup."=w1564:refnum<queue>)  [unwired: 7 in]
            n559 = call "Enqueue Message.vi"("error in"=w1556, "Message"="AutoApproachFast.Piezo", "Queue"=w1564) -> ("error out"=w1555:errorcluster)  [unwired: 7 in, 1 out]
          }
          frame "AutoApproachFast.InitWatchDog" {
            n560 = xnode "Read/Write Control"("FPGA VI Reference In"=w1592, "error in"=w1593) -> ("FPGA VI Reference Out"=w1589:T4, "error out"=w1588:errorcluster, "fb.p.limits.upperLimit"=w1584:fxp<+/-,28,4>)
            n561 = local read "Ztreshold"() -> (w1583:dbl)
            n562 = Multiply(x=w1584, y=w1583) -> (x*y=w1582:dbl)
            n563 = xnode "Read/Write Control"("FPGA VI Reference In"=w1589, "error in"=w1588, "fb.p.zWatchDogTreshold"=w1582) -> ("FPGA VI Reference Out"=w1587:T4, "error out"=w1585:errorcluster)
            n564 = xnode "Invoke Method"("FPGA VI Reference In"=w1587, "error in"=w1585, "IRQ Number(s)"=8) -> ("FPGA VI Reference Out"=w1591:T4, "error out"=w1590:errorcluster)
          }
          frame "AutoApproachFast.Piezo" {
            n565 = flat-sequence {
              tunnel: w1608 -> [w1628]
              tunnel: [w1628] -> w1601
              frame #0 {
                # "wait for stepper\nmotor to settle"
                n566 = local read "Wait"() -> (w1629:u32)
                n567 = Wait (ms)(milliseconds to wait=w1629) -> ()  [unwired: 1 out]
              }
            }
            n568 = call "SICMExperimentOnCheck.vi"("error in (no error)"=w1601, "Refnum in"=w1602) -> ("error out"=w1597:errorcluster, "IsExperimentSICM?"=w1596:bool, "Refnum out"=w1600:T4)  [unwired: 7 in]
            n569 = case shown="False" w1596 {
              tunnel: w1600 -> [w1618 w1624]
              tunnel: w1597 -> [w1617 w1623]
              tunnel: [w1616 w1620] -> w1599
              tunnel: [w1614 w1619] -> w1598
              frame False {
                w1613 = TRUE ("fb.p.enable")
                n570 = xnode "Read/Write Control"("FPGA VI Reference In"=w1618, "error in"=w1617, "fb.p.enable"=w1613) -> ("FPGA VI Reference Out"=w1616:T4, "error out"=w1615:errorcluster)
                n571 = property on="Feedback On" class="Bool (strict)"(error in=w1615, "Value"=w1613) -> (error out=w1614:errorcluster)  [unwired: 1 in, 1 out]
              }
              frame True {
                n572 = xnode "Read/Write Control"("FPGA VI Reference In"=w1624, "error in"=w1623) -> ("FPGA VI Reference Out"=w1622:T4, "error out"=w1621:errorcluster, "sicm.p.modes"=w1627:T30)
                n573 = Bundle By Name(cluster=w1627, "sicm.p.enable"=TRUE) -> (w1626:T30)
                n574 = xnode "Read/Write Control"("FPGA VI Reference In"=w1622, "error in"=w1621, "sicm.p.modes"=w1626) -> ("FPGA VI Reference Out"=w1620:T4, "error out"=w1619:errorcluster)
              }
            }
            n575 = xnode "Read/Write Control"("FPGA VI Reference In"=w1599, "error in"=w1598, "fb.zWatchdogArm"=TRUE ("fb.p.enable")) -> ("FPGA VI Reference Out"=w1609:T4, "error out"=w1606:errorcluster)
            n576 = call "Enqueue Message.vi"("error in"=w1606, "Message"="AutoApproachFast.CheckWatchDog", "Queue"=w1612) -> ("error out"=w1607:errorcluster)  [unwired: 7 in, 1 out]
          }
          frame "AutoApproachFast.CheckWatchDog" {
            w1646 = 8 ("IRQ Number(s)")
            # "The duration of the piezo extension should last less than 200ms"
            n577 = xnode "Read/Write Control"("FPGA VI Reference In"=w1649, "error in"=w1650) -> ("FPGA VI Reference Out"=w1645:T4, "error out"=w1644:errorcluster, "fb.o.height"=w1633:fxp<+/-,31,4>)
            n578 = xnode "Invoke Method"("FPGA VI Reference In"=w1645, "error in"=w1644, "IRQ Number(s)"=w1646, "Timeout (ms)"=50) -> ("FPGA VI Reference Out"=w1642:T4, "error out"=w1641:errorcluster, "Timed Out"=w1637:bool)  [unwired: 1 out]
            n579 = property on="Stop" class="Bool (strict)"() -> ("Value"=w1631:bool)  [unwired: 2 in, 2 out]
            n580 = Compound Arithmetic op=OR(w1637, w1631) -> (w1638:bool)
            n581 = xnode "Read/Write Control"("FPGA VI Reference In"=w1642, "error in"=w1641) -> ("FPGA VI Reference Out"=w1634:T4, "error out"=w1635:errorcluster, "fb.o.height"=w1632:fxp<+/-,31,4>)
            n582 = Subtract(x=w1632, y=w1633) -> (x-y=w1640:fxp<+/-,32,5>)
            n583 = Greater?(x=w1640, y="zMoveTresh") -> (0:w1636:bool)
            n584 = case shown="True" w1638 {
              tunnel: w1636 -> [_ w1680]
              tunnel: w1635 -> [w1657 w1679]
              tunnel: [w1659 w1678] -> w1648
              tunnel: w1653 -> [w1662 w1677]
              tunnel: w1634 -> [w1658 w1676]
              tunnel: [w1656 w1675] -> w1647
              tunnel: w1646 -> [w1661 _]
              tunnel: w1632 -> [_ w1674]
              tunnel: w1633 -> [_ w1673]
              tunnel: w1631 -> [_ w1672]
              frame False {
                n585 = xnode "Invoke Method"("FPGA VI Reference In"=w1658, "error in"=w1657, "IRQ Number(s)"=w1661) -> ("FPGA VI Reference Out"=w1656:T4, "error out"=w1655:errorcluster)
                n586 = disable-structure shown="Disabled" {
                  disable-tunnel: [w1668 w1670] -> w1663
                  disable-tunnel: w1662 -> [w1667 w1670]
                  disable-tunnel: w1655 -> [w1665 w1669]
                  disable-tunnel: [w1664 w1669] -> w1654
                  frame Disabled {
                    n587 = call "Enqueue Message.vi"("error in"=w1665, "Message"="Z.ManualMotion.Withdraw", "Queue"=w1667) -> ("error out"=w1664:errorcluster, "Queue dup."=w1668:refnum<queue>)  [unwired: 7 in]
                  }
                  frame Enabled {
                  }
                }
                n588 = call "Enqueue Message.vi"("error in"=w1654, "Message"="AutoApproachFast.Motor", "Queue"=w1663) -> ("error out"=w1659:errorcluster)  [unwired: 7 in, 1 out]
              }
              frame True {
                n589 = Compound Arithmetic op=OR(invert w1680, w1672) -> (w1671:bool)
                n590 = case shown="True" w1671 {
                  tunnel: w1679 -> [w1682 w1690]
                  tunnel: [w1681 w1693] -> w1678
                  tunnel: w1677 -> [w1685 w1694]
                  tunnel: w1676 -> [w1684 w1691]
                  tunnel: [w1684 w1687] -> w1675
                  tunnel: w1674 -> [_ _]
                  tunnel: w1673 -> [_ _]
                  frame False {
                    # "z Value still moved appreciably,\n keep going"
                    n591 = call "Enqueue Message.vi"("error in"=w1682, "Message"="AutoApproachFast.CheckWatchDog", "Queue"=w1685) -> ("error out"=w1681:errorcluster)  [unwired: 7 in, 1 out]
                  }
                  frame True {
                    w1696 = FALSE ("Value")
                    # "z value didn't change much,\nlet's stay here!"
                    n592 = local read "Withdraw/landed"() -> (w1695:bool)
                    n593 = property on="Approaching?" class="Bool (strict)"("Value"=w1696) -> ()  [unwired: 2 in, 2 out]
                    n594 = property on="Stop" class="Bool (strict)"("Value"=w1696) -> ()  [unwired: 2 in, 2 out]
                    n595 = call "SICMExperimentOnCheck.vi"("error in (no error)"=w1690, "Refnum in"=w1691) -> ("error out"=w1689:errorcluster, "IsExperimentSICM?"=w1686:bool, "Refnum out"=w1688:T4)  [unwired: 7 in]
                    n596 = case shown="True" w1695 {
                      tunnel: w1694 -> [_ w1705]
                      tunnel: w1689 -> [w1699 w1704]
                      tunnel: [w1699 w1703] -> w1693
                      tunnel: w1688 -> [w1698 w1702]
                      tunnel: [w1698 w1701] -> w1687
                      tunnel: w1686 -> [_ w1700]
                      frame False {
                      }
                      frame True {
                        n597 = case shown="False" w1700 {
                          tunnel: w1705 -> [w1709 _]
                          tunnel: w1704 -> [w1708 w1715]
                          tunnel: [w1707 w1716] -> w1703
                          tunnel: w1702 -> [w1710 w1714]
                          tunnel: [w1710 w1713] -> w1701
                          frame False {
                            n598 = call "Enqueue Message.vi"("error in"=w1708, "Message"="Z.ManualMotion.Withdraw", "Queue"=w1709) -> ("error out"=w1707:errorcluster)  [unwired: 7 in, 1 out]
                          }
                          frame True {
                            n599 = xnode "Read/Write Control"("FPGA VI Reference In"=w1714, "error in"=w1715) -> ("FPGA VI Reference Out"=w1712:T4, "error out"=w1711:errorcluster, "sicm.p.modes"=w1717:T30)
                            n600 = Bundle By Name(cluster=w1717, "sicm.p.enable"=FALSE) -> (w1718:T30)
                            n601 = xnode "Read/Write Control"("FPGA VI Reference In"=w1712, "error in"=w1711, "sicm.p.modes"=w1718) -> ("FPGA VI Reference Out"=w1713:T4, "error out"=w1716:errorcluster)
                          }
                        }
                      }
                    }
                    n602 = local read "Beep when finished"() -> (w1692:bool)
                    n603 = case shown="True" w1692 {
                      selector: w1692 -> [_ w1697]
                      frame False {
                      }
                      frame True {
                        n604 = call <vilib>:"Beep.vi"("use system alert? (T)"=w1697) -> ()  [unwired: 11 in]
                      }
                    }
                  }
                }
              }
            }
          }
          frame "AutoApproachFast.Motor" {
            n605 = call "SICMExperimentOnCheck.vi"("error in (no error)"=w1725, "Refnum in"=w1724) -> ("error out"=w1723:errorcluster, "IsExperimentSICM?"=w1722:bool, "Refnum out"=w1720:T4)  [unwired: 7 in]
            n606 = case shown="True" w1722 {
              tunnel: w1733 -> [w1738 w1748]
              tunnel: [w1737 w1748] -> w1730
              tunnel: [w1736 w1744] -> w1729
              tunnel: w1723 -> [w1734 w1743]
              tunnel: w1720 -> [w1739 w1742]
              tunnel: [w1739 w1740] -> w1721
              frame False {
                n607 = call "Enqueue Message.vi"("error in"=w1734, "Message"="Z.ManualMotion.Withdraw", "Queue"=w1738) -> ("error out"=w1736:errorcluster, "Queue dup."=w1737:refnum<queue>)  [unwired: 7 in]
              }
              frame True {
                n608 = xnode "Read/Write Control"("FPGA VI Reference In"=w1742, "error in"=w1743) -> ("FPGA VI Reference Out"=w1741:T4, "sicm.p.modes"=w1745:T30)  [unwired: 1 out]
                n609 = Bundle By Name(cluster=w1745, "sicm.p.enable"=FALSE) -> (w1746:T30)
                n610 = xnode "Read/Write Control"("FPGA VI Reference In"=w1741, "sicm.p.modes"=w1746) -> ("FPGA VI Reference Out"=w1740:T4, "error out"=w1744:errorcluster)  [unwired: 1 in]
              }
            }
            n611 = local read "Type"() -> (w1727:T3)
            n612 = case shown="\"DC motor\"" w1727 {
              tunnel: w1730 -> [w1764 w1775 w1782 w1786]
              tunnel: w1729 -> [w1759 w1766 w1779 w1788]
              tunnel: [w1749 w1767 w1776 w1787] -> w1728
              frame "Step motor", Default {
                w1754 = -1  # Down
                n613 = local read "Steps"() -> (w1750:u32)
                n614 = call "FGVSteps.vi"("Enum"=Enum."Read", "error in"=w1759) -> ("error out"=w1765:errorcluster, "stepglobalCounterOut"=w1757:i32, "stepsOut"=w1758:i32)  [unwired: 6 in, 1 out]
                n615 = To Long Integer(number=w1750) -> (32bit integer=w1751:i32)
                n616 = call "FGVSteps.vi"("Enum"=Enum."Write", "error in"=w1765, "stepsglobalCounterIn"=w1757, "stepsLeftIn"=w1751, "stepsIn"=w1758) -> ("error out"=w1760:errorcluster)  [unwired: 3 in, 3 out]
                n617 = Bundle(cluster=cluster{"DirectionStep":i32, "WaitForStep":bool} {"DirectionStep"=0, "WaitForStep"=FALSE}, "DirectionStep"=w1754, "WaitForStep"=TRUE) -> (w1756:cluster{"DirectionStep":i32, "WaitForStep":bool})
                n618 = To Variant(anything=w1756) -> (Variant=w1752:variant)
                n619 = call "Enqueue Message.vi"("error in"=w1760, "Data"=w1752, "Message"="StepMotor.SendSteps", "Queue"=w1764) -> ("error out"=w1749:errorcluster)  [unwired: 6 in, 1 out]
              }
              frame "DC motor" {
                n620 = property on="Down" class="Bool (strict)"(error in=w1766, "Value"=TRUE) -> (error out=w1774:errorcluster)  [unwired: 1 in, 1 out]
                n621 = control-ref of="Down"() -> (w1772:refnum<vi>)
                n622 = call "Enqueue Message.vi"("error in"=w1774, "Data"=w1772, "Message"="DCMotor.SendVoltage", "Queue"=w1775) -> ("error out"=w1771:errorcluster, "Queue dup."=w1770:refnum<queue>)  [unwired: 6 in]
                n623 = call "Enqueue Message.vi"("error in"=w1771, "Message"="DCMotor.Stop", "Queue"=w1770) -> ("error out"=w1767:errorcluster)  [unwired: 7 in, 1 out]
              }
              frame "Stepper Motor Driver" {
                n624 = control-ref of="Down"() -> (w1780:refnum<vi>)
                n625 = call "Enqueue Message.vi"("error in"=w1779, "Data"=w1780, "Message"="SmdInterface.Start", "Queue"=w1782) -> ("error out"=w1777:errorcluster, "Queue dup."=w1783:refnum<queue>)  [unwired: 6 in]
                n626 = call "Enqueue Message.vi"("error in"=w1777, "Message"="SmdInterface.Stop", "Queue"=w1783) -> ("error out"=w1776:errorcluster)  [unwired: 7 in, 1 out]
              }
              frame "Stick-Slip" {
                n627 = control-ref of="Down"() -> (w1784:refnum<vi>)
                n628 = call "Enqueue Message.vi"("error in"=w1788, "Data"=w1784, "Message"="StickSlip.Move", "Queue"=w1786) -> ("error out"=w1787:errorcluster)  [unwired: 6 in, 1 out]
              }
            }
          }
          frame "AutoApproachFast.Stop" {
            w1798 = FALSE ("Approaching?")
            n629 = call "SICMExperimentOnCheck.vi"("error in (no error)"=w1794, "Refnum in"=w1791) -> ("error out"=w1793:errorcluster, "IsExperimentSICM?"=w1789:bool, "Refnum out"=w1792:T4)  [unwired: 7 in]
            n630 = case shown="False" w1789 {
              tunnel: [w1804 w1810] -> w1797
              tunnel: w1796 -> [w1803 _]
              tunnel: w1793 -> [w1801 w1811]
              tunnel: w1792 -> [w1805 w1809]
              tunnel: [w1805 w1807] -> w1790
              frame False {
                n631 = call "Enqueue Message.vi"("error in"=w1801, "Message"="Z.ManualMotion.Withdraw", "Queue"=w1803) -> ("error out"=w1804:errorcluster)  [unwired: 7 in, 1 out]
              }
              frame True {
                n632 = xnode "Read/Write Control"("FPGA VI Reference In"=w1809, "error in"=w1811) -> ("FPGA VI Reference Out"=w1808:T4, "sicm.p.modes"=w1812:T30)  [unwired: 1 out]
                n633 = Bundle By Name(cluster=w1812, "sicm.p.enable"=FALSE) -> (w1806:T30)
                n634 = xnode "Read/Write Control"("FPGA VI Reference In"=w1808, "sicm.p.modes"=w1806) -> ("FPGA VI Reference Out"=w1807:T4, "error out"=w1810:errorcluster)  [unwired: 1 in]
              }
            }
            n635 = local write "Approaching?"(w1798) -> ()
            n636 = property on="Stop" class="Bool (strict)"("Value"=w1798) -> ()  [unwired: 2 in, 2 out]
          }
          frame "------  AutoApproach  ------" {
          }
          frame "AutoApproach.Init" {
            n637 = call "Enqueue Message.vi"("error in"=w1829, "Message"="Z.ManualMotion.Withdraw", "Queue"=w1828) -> ("error out"=w1831:errorcluster, "Queue dup."=w1832:refnum<queue>)  [unwired: 7 in]
            n638 = Select(t="AutoApproach.RelativePiezo" ("Message"), s="Relative Setpoint", f="AutoApproach.Piezo" ("Message")) -> (s? t:f=w1820:string)
            n639 = call "Enqueue Message.vi"("error in"=w1831, "Message"=w1820, "Queue"=w1832) -> ("error out"=w1830:errorcluster)  [unwired: 7 in, 1 out]
          }
          frame "AutoApproach.Piezo" {
            # "Changed for ORT"
            # "true if we need to move the Motor"
            # "Feedback enable\n1) if Zheight >=0.95, we need to withdraw and send steps\n2) if Zheight<0.95 AND\n    a) Zheight(N-1) > Zheight(N), we are still looking for surface\n    b) Zheight(N-1) =<Zheight(N), we found the surface"
            # "Wait for Z-Controller\nto be switched on"
            # "Switch Z-Controller ON"
            n640 = xnode "Read/Write Control"("FPGA VI Reference In"=w1858, "error in"=w1859, "fb.p.enable"=TRUE ("enableFeedback")) -> ("FPGA VI Reference Out"=w1857:T4, "error out"=w1856:errorcluster, "fb.p.limits.lowerLimit"=w1842:fxp<+/-,28,4>)
            n641 = property on="Mode" class="Enum (strict)"() -> ("Value"=w1839:enum16{"Contact", "OR Tapping", "Aux"})  [unwired: 2 in, 2 out]
            n642 = To Double Precision Float(number=w1842) -> (double precision float=w1834:dbl)
            n643 = while {
              tunnel: w1857 -> [w1887]
              tunnel: w1856 -> [w1886]
              tunnel: [w1883] -> w1854
              tunnel: [w1882] -> w1851
              tunnel: [TRUE] -> w1849
              stop <- w1885 stop-if-true
              n644 = xnode "Read/Write Control"("FPGA VI Reference In"=w1887, "error in"=w1886) -> ("FPGA VI Reference Out"=w1882:T4, "error out"=w1883:errorcluster, "fb.p.enable"=w1885:bool)
              n645 = Wait (ms)(milliseconds to wait=u32 2) -> ()  [unwired: 1 out]
            }
            n646 = local write "Approaching?"(w1849) -> ()
            n647 = Equal?(x=w1839, y=enum16{"Contact", "OR Tapping", "Aux"}."Aux" ("Mode")) -> (x = y?=w1837:bool)
            n648 = disable-structure shown="Enabled" {
              disable-tunnel: [w1862 1.0 ("voltageRange(+/-)Out")] -> w1840
              frame Enabled {
                n649 = call "FGVfpgaAdress.vi"("Enum"=Enum."Read") -> ("voltageRange(+/-)Out"=w1862:dbl)  [unwired: 5 in, 5 out]
              }
              frame Disabled {
              }
            }
            n650 = Absolute Value(x=w1834) -> (abs(x)=w1841:dbl)
            n651 = Multiply(x=w1841, y="Ztreshold") -> (x*y=w1843:dbl)
            n652 = while {
              shift-right: [w1889] -> _
              shift-left: -inf -> [w1918]
              tunnel: w1843 -> [w1917]
              tunnel: w1854 -> [w1916]
              tunnel: [w1913] -> w1852
              tunnel: [w1909] -> w1848
              tunnel: w1851 -> [w1901]
              tunnel: [w1897] -> w1850
              tunnel: w1840 -> [w1900]
              tunnel: fxp<+/-,17,1> 0.0 ("setPoint") -> [w1899]
              tunnel: T13 {"setPoint"=0.0, "pGain"=0.0, "iGain"=0.0, "setPointAlt"=0.0} ("fbParams") -> [w1898]
              tunnel: w1837 -> [w1893]
              stop <- w1912 stop-if-true
              # "stop"
              n653 = xnode "Read/Write Control"("FPGA VI Reference In"=w1901, "error in"=w1916) -> ("FPGA VI Reference Out"=w1897:T4, "error out"=w1913:errorcluster, "fb.o.height"=w1915:fxp<+/-,31,4>)
              n654 = local read "PID"() -> (w1902:T1)
              n655 = Unbundle By Name(w1902) -> ("Setpoint"=w1903:dbl, "P Gain"=w1894:dbl, "I Gain"=w1892:dbl)
              n656 = To Double Precision Float(number=w1915) -> (double precision float=w1889:dbl)
              n657 = Greater?(x=w1889, y=w1918) -> (0:w1910:bool)
              n658 = Less?(x=w1889, y=w1917) -> (x < y?=w1909:bool)
              n659 = property on="Stop" class="Bool (strict)"() -> ("Value"=w1896:bool)  [unwired: 2 in, 2 out]
              n660 = Divide(x=w1903, y=w1900) -> (x/y=w1904:dbl)
              n661 = Not(x=w1910) -> (.not. x?=w1908:bool)
              "Surface reached" <- w1908
              n662 = And(x=w1910, y=w1909) -> (x .and. y?=w1911:bool)
              n663 = disable-structure shown="Enabled" {
                disable-tunnel: [w1924 w1926] -> w1895
                disable-tunnel: w1894 -> [w1922 w1926]
                disable-tunnel: w1893 -> [w1921 _]
                disable-tunnel: w1892 -> [w1920 w1927]
                disable-tunnel: [w1919 w1927] -> w1891
                frame Disabled {
                  n664 = Negate(x=w1922) -> (-x=w1925:dbl)
                  n665 = Negate(x=w1920) -> (-x=w1923:dbl)
                  n666 = Select(t=w1922, s=w1921, f=w1925) -> (s? t:f=w1924:dbl)
                  n667 = Select(t=w1920, s=w1921, f=w1923) -> (s? t:f=w1919:dbl)
                }
                frame Enabled {
                }
              }
              n668 = To Fixed-Point(fixed-point type=w1899, number=w1904) -> (fixed-point=w1906:fxp<+/-,17,1>)
              n669 = Not(x=w1911) -> (.not. x?=w1907:bool)
              n670 = Or(x=w1907, y=w1896) -> (x .or. y?=w1912:bool)
              n671 = And(x="Beep when finished", y=w1908) -> (x .and. y?=w1914:bool)
              n672 = Bundle By Name(cluster=w1898, "setPoint"=w1906, "pGain"=w1895, "iGain"=w1891) -> (w1905:T13)
              n673 = case shown="False" w1914 {
                selector: w1914 -> [_ w1928]
                frame False {
                }
                frame True {
                  n674 = call <vilib>:"Beep.vi"("use system alert? (T)"=w1928) -> ()  [unwired: 11 in]
                }
              }
              n675 = Wait (ms)(milliseconds to wait=u32 1) -> ()  [unwired: 1 out]
              n676 = call "PIDParameters.vi"("fbParams"=w1905, "FPGA VI Reference In"=w1901) -> ()  [unwired: 8 in, 2 out]
            }
            n677 = Not(x=w1848) -> (.not. x?=w1847:bool)
            n678 = case shown="False" w1847 {
              selector: w1847 -> [_ w1876]
              tunnel: w1861 -> [w1867 w1880]
              tunnel: [w1869 w1878] -> w1853
              tunnel: w1852 -> [w1868 w1877]
              frame False {
                n679 = case shown="True" "Withdraw/landed" {
                  tunnel: [w1870 w1873] -> w1869
                  tunnel: w1868 -> [w1870 w1872]
                  tunnel: w1867 -> [_ w1874]
                  frame False {
                  }
                  frame True {
                    n680 = call "Enqueue Message.vi"("error in"=w1872, "Message"="Z.ManualMotion.Withdraw", "Queue"=w1874) -> ("error out"=w1873:errorcluster)  [unwired: 7 in, 1 out]
                  }
                }
                n681 = local write "Approaching?"(FALSE ("Approaching?")) -> ()
              }
              frame True {
                n682 = To Variant(anything=w1876) -> (Variant=w1875:variant)
                n683 = call "Enqueue Message.vi"("error in"=w1877, "Data"=w1875, "Message"="AutoApproach.Motor", "Queue"=w1880) -> ("error out"=w1878:errorcluster)  [unwired: 6 in, 1 out]
              }
            }
          }
          frame "AutoApproach.RelativePiezo" {
            w1935 = 10.0  # Voltage Range FB
            # "Changed for ORT"
            # "true if we need to move the Motor"
            # "Feedback enable\n1) if Zheight >=0.95, we need to withdraw and send steps\n2) if Zheight<0.95 AND\n    a) Zheight(N-1) > Zheight(N), we are still looking for surface\n    b) Zheight(N-1) =<Zheight(N), we found the surface"
            # "Wait for Z-Controller\nto be switched on"
            # "Switch Z-Controller ON"
            n684 = xnode "Read/Write Control"("FPGA VI Reference In"=w1959, "error in"=w1960, "fb.p.enable"=TRUE ("enableFeedback")) -> ("FPGA VI Reference Out"=w1958:T4, "error out"=w1957:errorcluster, "fb.p.limits.lowerLimit"=w1944:fxp<+/-,28,4>, "aio.s.slowVertical"=w1931:i16)
            n685 = local read "Ztreshold"() -> (w1936:dbl)
            n686 = To Double Precision Float(number=w1944) -> (double precision float=w1929:dbl)
            n687 = To Double Precision Float(number=w1931) -> (double precision float=w1933:dbl)
            n688 = while {
              tunnel: w1958 -> [w1989]
              tunnel: w1957 -> [w1988]
              tunnel: [w1985] -> w1955
              tunnel: [w1984] -> w1952
              tunnel: [TRUE] -> w1950
              stop <- w1987 stop-if-true
              n689 = xnode "Read/Write Control"("FPGA VI Reference In"=w1989, "error in"=w1988) -> ("FPGA VI Reference Out"=w1984:T4, "error out"=w1985:errorcluster, "fb.p.enable"=w1987:bool)
              n690 = Wait (ms)(milliseconds to wait=u32 2) -> ()  [unwired: 1 out]
            }
            n691 = local write "Approaching?"(w1950) -> ()
            n692 = Scale By Power Of 2(n=i16 -15, x=w1933) -> (x*2^n=w1934:dbl)
            n693 = disable-structure shown="Enabled" {
              disable-tunnel: [w1964 1.0 ("voltageRange(+/-)Out")] -> w1942
              frame Enabled {
                n694 = call "FGVfpgaAdress.vi"("Enum"=Enum."Read") -> ("voltageRange(+/-)Out"=w1964:dbl)  [unwired: 5 in, 5 out]
              }
              frame Disabled {
              }
            }
            n695 = Absolute Value(x=w1929) -> (abs(x)=w1943:dbl)
            n696 = property on="Mode" class="Enum (strict)"() -> ("Value"=w1941:enum16{"Contact", "OR Tapping", "Aux"})  [unwired: 2 in, 2 out]
            n697 = Multiply(x=w1935, y=w1934) -> (x*y=w1930:dbl)
            n698 = Multiply(x=w1943, y=w1936) -> (x*y=w1945:dbl)
            n699 = Equal?(x=w1941, y=enum16{"Contact", "OR Tapping", "Aux"}."Aux" ("Mode")) -> (x = y?=w1939:bool)
            n700 = while {
              shift-right: [w1995] -> _
              shift-left: -inf -> [w2021]
              tunnel: w1945 -> [w2020]
              tunnel: w1955 -> [w2019]
              tunnel: [w2016] -> w1953
              tunnel: [w2012] -> w1949
              tunnel: w1952 -> [w2006]
              tunnel: [w2002] -> w1951
              tunnel: w1942 -> [w2005]
              tunnel: fxp<+/-,17,1> 0.0 ("setPoint") -> [w2004]
              tunnel: T13 {"setPoint"=0.0, "pGain"=0.0, "iGain"=0.0, "setPointAlt"=0.0} ("fbParams") -> [w2003]
              tunnel: w1939 -> [w1998]
              tunnel: w1930 -> [w1992]
              stop <- w2015 stop-if-true
              # "stop"
              n701 = local read "PID"() -> (w2007:T1)
              n702 = xnode "Read/Write Control"("FPGA VI Reference In"=w2006, "error in"=w2019) -> ("FPGA VI Reference Out"=w2002:T4, "error out"=w2016:errorcluster, "fb.o.height"=w2018:fxp<+/-,31,4>)
              n703 = Unbundle By Name(w2007) -> ("Setpoint"=w1991:dbl, "P Gain"=w1999:dbl, "I Gain"=w1997:dbl)
              n704 = local read "Beep when finished"() -> (w1994:bool)
              n705 = To Double Precision Float(number=w2018) -> (double precision float=w1995:dbl)
              n706 = Multiply(x=w1992, y=w1991) -> (x*y=w1990:dbl)
              n707 = disable-structure shown="Enabled" {
                disable-tunnel: [w2027 w2029] -> w2000
                disable-tunnel: w1999 -> [w2025 w2029]
                disable-tunnel: w1998 -> [w2024 _]
                disable-tunnel: w1997 -> [w2023 w2030]
                disable-tunnel: [w2022 w2030] -> w1996
                frame Disabled {
                  n708 = Negate(x=w2025) -> (-x=w2028:dbl)
                  n709 = Negate(x=w2023) -> (-x=w2026:dbl)
                  n710 = Select(t=w2025, s=w2024, f=w2028) -> (s? t:f=w2027:dbl)
                  n711 = Select(t=w2023, s=w2024, f=w2026) -> (s? t:f=w2022:dbl)
                }
                frame Enabled {
                }
              }
              n712 = Greater?(x=w1995, y=w2021) -> (0:w2013:bool)
              n713 = Less?(x=w1995, y=w2020) -> (x < y?=w2012:bool)
              n714 = Divide(x=w1990, y=w2005) -> (x/y=w2008:dbl)
              n715 = Not(x=w2013) -> (.not. x?=w1993:bool)
              n716 = And(x=w2013, y=w2012) -> (x .and. y?=w2014:bool)
              n717 = To Fixed-Point(fixed-point type=w2004, number=w2008) -> (fixed-point=w2010:fxp<+/-,17,1>)
              n718 = property on="Stop" class="Bool (strict)"() -> ("Value"=w2001:bool)  [unwired: 2 in, 2 out]
              n719 = Not(x=w2014) -> (.not. x?=w2011:bool)
              n720 = local write "Surface reached"(w1993) -> ()
              n721 = And(x=w1994, y=w1993) -> (x .and. y?=w2017:bool)
              n722 = Bundle By Name(cluster=w2003, "setPoint"=w2010, "pGain"=w2000, "iGain"=w1996) -> (w2009:T13)
              n723 = Or(x=w2011, y=w2001) -> (x .or. y?=w2015:bool)
              n724 = case shown="True" w2017 {
                selector: w2017 -> [_ w2031]
                frame False {
                }
                frame True {
                  n725 = call <vilib>:"Beep.vi"("use system alert? (T)"=w2031) -> ()  [unwired: 11 in]
                }
              }
              n726 = call "PIDParameters.vi"("fbParams"=w2009, "FPGA VI Reference In"=w2006) -> ()  [unwired: 8 in, 2 out]
            }
            n727 = Not(x=w1949) -> (.not. x?=w1948:bool)
            n728 = case shown="False" w1948 {
              selector: w1948 -> [_ w1978]
              tunnel: w1962 -> [w1969 w1982]
              tunnel: [w1971 w1980] -> w1954
              tunnel: w1953 -> [w1970 w1979]
              frame False {
                n729 = local read "Withdraw/landed"() -> (w1967:bool)
                n730 = case shown="False" w1967 {
                  tunnel: [w1972 w1975] -> w1971
                  tunnel: w1970 -> [w1972 w1974]
                  tunnel: w1969 -> [_ w1976]
                  frame False {
                  }
                  frame True {
                    n731 = call "Enqueue Message.vi"("error in"=w1974, "Message"="Z.ManualMotion.Withdraw", "Queue"=w1976) -> ("error out"=w1975:errorcluster)  [unwired: 7 in, 1 out]
                  }
                }
                n732 = local write "Approaching?"(FALSE ("Approaching?")) -> ()
              }
              frame True {
                n733 = To Variant(anything=w1978) -> (Variant=w1977:variant)
                n734 = call "Enqueue Message.vi"("error in"=w1979, "Data"=w1977, "Message"="AutoApproach.Motor", "Queue"=w1982) -> ("error out"=w1980:errorcluster)  [unwired: 6 in, 1 out]
              }
            }
          }
          frame "AutoApproach.Motor" {
            n735 = Variant To Data(error in=w2041, type=TRUE, Variant=w2040) -> (data=w2037:bool, error out=w2036:errorcluster)
            n736 = case shown="True" w2037 {
              tunnel: [w2049 w2060] -> w2038
              tunnel: w2042 -> [w2051 w2064]
              tunnel: w2036 -> [w2050 w2062]
              frame False {
                n737 = control-ref of="Stop"() -> (w2046:refnum<vi>)
                n738 = local read "Withdraw/landed"() -> (w2048:bool)
                n739 = local read "Surface reached"() -> (w2047:bool)
                n740 = property class="Bool (strict)"(reference=w2046) -> ("Value"=w2045:bool)  [unwired: 1 in, 2 out]
                n741 = Compound Arithmetic op=AND(w2047, invert w2048) -> (w2044:bool)
                n742 = Or(x=w2044, y=w2045) -> (x .or. y?=w2043:bool)
                n743 = case shown="False" w2043 {
                  tunnel: w2051 -> [w2056 _]
                  tunnel: w2050 -> [w2054 w2058]
                  tunnel: [w2053 w2058] -> w2049
                  frame True {
                    w2052 = FALSE ("Approaching?")
                    n744 = local write "Surface reached"(w2052) -> ()
                    n745 = local write "Approaching?"(w2052) -> ()
                    n746 = call "Enqueue Message.vi"("error in"=w2054, "Message"="Z.ManualMotion.Withdraw", "Queue"=w2056) -> ("error out"=w2053:errorcluster)  [unwired: 7 in, 1 out]
                    n747 = property on="Stop" class="Bool (strict)"("Value"=w2052) -> ()  [unwired: 2 in, 2 out]
                  }
                  frame False {
                    w2057 = FALSE ("Approaching?")
                    n748 = local write "Surface reached"(w2057) -> ()
                    n749 = local write "Approaching?"(w2057) -> ()
                    n750 = property on="Stop" class="Bool (strict)"("Value"=w2057) -> ()  [unwired: 2 in, 2 out]
                  }
                }
              }
              frame True {
                n751 = call "Enqueue Message.vi"("error in"=w2062, "Message"="Z.ManualMotion.Withdraw", "Queue"=w2064) -> ("error out"=w2063:errorcluster, "Queue dup."=w2065:refnum<queue>)  [unwired: 7 in]
                n752 = local read "Type"() -> (w2059:T3)
                n753 = case shown="\"DC motor\"" w2059 {
                  tunnel: w2065 -> [w2081 w2091 w2094 w2101]
                  tunnel: w2063 -> [w2076 w2083 w2096 w2099]
                  tunnel: [w2074 w2087 w2095 w2098] -> w2060
                  frame "Step motor", Default {
                    w2070 = -1  # Down
                    n754 = call "FGVSteps.vi"("Enum"=Enum."Read", "error in"=w2076) -> ("error out"=w2082:errorcluster, "stepglobalCounterOut"=w2073:i32, "stepsOut"=w2075:i32)  [unwired: 6 in, 1 out]
                    n755 = To Long Integer(number="Steps") -> (32bit integer=w2066:i32)
                    n756 = call "FGVSteps.vi"("Enum"=Enum."Write", "error in"=w2082, "stepsglobalCounterIn"=w2073, "stepsLeftIn"=w2066, "stepsIn"=w2075) -> ("error out"=w2077:errorcluster)  [unwired: 3 in, 3 out]
                    n757 = Bundle(cluster=cluster{"DirectionStep":i32, "WaitForStep":bool} {"DirectionStep"=0, "WaitForStep"=FALSE}, "DirectionStep"=w2070, "WaitForStep"=TRUE) -> (w2072:cluster{"DirectionStep":i32, "WaitForStep":bool})
                    n758 = To Variant(anything=w2072) -> (Variant=w2067:variant)
                    n759 = call "Enqueue Message.vi"("error in"=w2077, "Data"=w2067, "Message"="StepMotor.SendSteps", "Queue"=w2081) -> ("error out"=w2074:errorcluster)  [unwired: 6 in, 1 out]
                  }
                  frame "DC motor" {
                    n760 = property on="Down" class="Bool (strict)"(error in=w2083, "Value"=TRUE) -> (error out=w2092:errorcluster)  [unwired: 1 in, 1 out]
                    n761 = control-ref of="Down"() -> (w2089:refnum<vi>)
                    n762 = call "Enqueue Message.vi"("error in"=w2092, "Data"=w2089, "Message"="DCMotor.SendVoltage", "Queue"=w2091) -> ("error out"=w2088:errorcluster, "Queue dup."=w2086:refnum<queue>)  [unwired: 6 in]
                    n763 = call "Enqueue Message.vi"("error in"=w2088, "Message"="DCMotor.Stop", "Queue"=w2086) -> ("error out"=w2087:errorcluster)  [unwired: 7 in, 1 out]
                  }
                  frame "Stepper Motor Driver" {
                    n764 = call "Enqueue Message.vi"("error in"=w2096, "Message"="SmdInterface.Start", "Queue"=w2094) -> ("error out"=w2095:errorcluster)  [unwired: 7 in, 1 out]
                  }
                  frame "Stick-Slip" {
                    n765 = control-ref of="Down"() -> (w2097:refnum<vi>)
                    n766 = call "Enqueue Message.vi"("error in"=w2099, "Data"=w2097, "Message"="StickSlip.Move", "Queue"=w2101) -> ("error out"=w2098:errorcluster)  [unwired: 6 in, 1 out]
                  }
                }
              }
            }
          }
          frame "AutoApproach.Stop" {
            n767 = xnode "Read/Write Control"("FPGA VI Reference In"=w2109, "error in"=w2108) -> ("FPGA VI Reference Out"=w2107:T4, "error out"=w2106:errorcluster, "fb.p.enable"=w2105:bool)
            n768 = case shown="False" w2105 {
              tunnel: [w2119 w2127] -> w2113
              tunnel: [w2117 w2126] -> w2112
              tunnel: w2110 -> [w2121 w2126]
              tunnel: w2106 -> [w2116 w2127]
              frame False {
                n769 = local read "Type"() -> (w2115:T3)
                n770 = case shown="\"Stepper Motor Driver\"" w2115 {
                  tunnel: ["StepMotor.StopSteps" ("Message") "DCMotor.Stop" ("Message") "SmdInterface.Stop" ("Message") "StickSlip.Stop" ("Message")] -> w2118
                  frame "Step motor", Default {
                  }
                  frame "DC motor" {
                  }
                  frame "Stepper Motor Driver" {
                  }
                  frame "Stick-Slip" {
                  }
                }
                n771 = call "Enqueue Message.vi"("Prioritary message"=TRUE ("Message prioritaire ? (F)"), "error in"=w2116, "Message"=w2118, "Queue"=w2121) -> ("error out"=w2119:errorcluster, "Queue dup."=w2117:refnum<queue>)  [unwired: 6 in]
              }
              frame True {
              }
            }
            n772 = local read "Approaching?"() -> (w2114:bool)
            n773 = case shown="True" w2114 {
              tunnel: w2112 -> [_ w2137]
              tunnel: [w2128 w2133] -> w2111
              tunnel: w2113 -> [w2129 w2132]
              frame False {
                n774 = property on="Stop" class="Bool (strict)"(error in=w2129, "Value"=FALSE) -> (error out=w2128:errorcluster)  [unwired: 1 in, 1 out]
              }
              frame True {
                n775 = To Variant(anything=FALSE ("Message prioritaire ? (F)")) -> (Variant=w2131:variant)
                n776 = call "Enqueue Message.vi"("Prioritary message"=TRUE ("Message prioritaire ? (F)"), "error in"=w2132, "Data"=w2131, "Message"="AutoApproach.Motor", "Queue"=w2137) -> ("error out"=w2133:errorcluster)  [unwired: 5 in, 1 out]
              }
            }
          }
          frame " ---- Controllers Config ----" {
          }
          frame "Mode.Update" {
            n777 = call "Enqueue Message.vi"("error in"=w2144, "Data"=w2143, "Message"="Controllers.Mode", "Queue"=w2162) -> ("error out"=w2161:errorcluster, "Queue dup."=w2150:refnum<queue>)  [unwired: 6 in]
            n778 = To Variant(anything="IO Frequency") -> (Variant=w2154:variant)
            n779 = call "Enqueue Message.vi"("error in"=w2161, "Data"=w2154, "Message"="Controllers.IOFrequency", "Queue"=w2150) -> ("error out"=w2151:errorcluster, "Queue dup."=w2159:refnum<queue>)  [unwired: 6 in]
            n780 = call "Enqueue Message.vi"("error in"=w2151, "Message"="Mode.Initialize", "Queue"=w2159) -> ("error out"=w2149:errorcluster, "Queue dup."=w2160:refnum<queue>)  [unwired: 7 in]
            n781 = call "Enqueue Message.vi"("error in"=w2149, "Message"="PID.Update", "Queue"=w2160) -> ("error out"=w2145:errorcluster)  [unwired: 7 in, 1 out]
          }
          frame "Controllers.Mode" {
            # "For mode selection after Aux, use Aux"
            # "Initialize the FPGA when changing the Feedback mode"
            n782 = Variant To Data(error in=w2184, type=enum16{"Contact", "OR Tapping", "Aux"}."Contact" ("Mode"), Variant=w2185) -> (data=w2167:enum16{"Contact", "OR Tapping", "Aux"}, error out=w2186:errorcluster)
            n783 = xnode "Read/Write Control"("FPGA VI Reference In"=w2181, "error in"=w2186) -> ("FPGA VI Reference Out"=w2182:T4, "error out"=w2189:errorcluster, "fb.loff.p.params"=w2178:T26)
            n784 = Bundle By Name(cluster=w2178, "disengagePos"=fxp<+/-,22,1> -0.6999998092651367) -> (w2179:T26)
            n785 = property on="Mode" class="Enum (strict)"(error in=w2189, "Value"=w2167) -> (error out=w2166:errorcluster)  [unwired: 1 in, 1 out]
            n786 = call "FGVpiezoLimits.vi"("Enum"=Enum."Read", "error in"=w2166) -> ("error out"=w2165:errorcluster, "PiezoLimitsOUT(1;-1)"=w2163:T27)  [unwired: 8 in]
            n787 = To Unsigned Byte Integer(number=w2167) -> (unsigned 8bit integer=w2173:u8)
            n788 = xnode "Read/Write Control"("FPGA VI Reference In"=w2182, "error in"=w2165, "fb.i.source"=w2173, "fb.p.limits"=w2163, "fb.loff.p.params"=w2179) -> ("FPGA VI Reference Out"=w2176:T4, "error out"=w2177:errorcluster)
            n789 = case shown="\"Contact\", Default" w2167 {
              tunnel: w2177 -> [w2195 w2203]
              tunnel: w2176 -> [w2197 w2204]
              tunnel: [w2200 w2203] -> w2188
              tunnel: [w2201 w2204] -> w2175
              tunnel: [T1 {"Setpoint"=0.05, "P Gain"=0.0, "I Gain"=0.0001} ("PID") T1 {"Setpoint"=0.005, "P Gain"=0.0, "I Gain"=0.01} ("PID")] -> w2169
              frame "Contact", Default {
                w2191 = FALSE ("ort.p.bypassAvg")
                w2198 = FALSE ("Feedback On")
                n790 = xnode "Read/Write Control"("FPGA VI Reference In"=w2197, "error in"=w2195) -> ("FPGA VI Reference Out"=w2196:T4, "ort.p.methodParams"=w2194:T31)  [unwired: 3 out]
                n791 = Bundle By Name(cluster=w2194, "ort.p.syncPoint"=u16 1, "ort.p.bypassAvg"=w2191, "ort.p.useSyncPoint"=w2191) -> (w2193:T31)
                n792 = xnode "Read/Write Control"("FPGA VI Reference In"=w2196, "aio.o.disableExc"=TRUE, "fb.p.enable"=w2198, "ort.p.methodParams"=w2193) -> ("FPGA VI Reference Out"=w2201:T4, "error out"=w2200:errorcluster)  [unwired: 1 in]
                n793 = local write "Feedback On"(w2198) -> ()
              }
              frame "OR Tapping" {
              }
            }
            n794 = property on="PID" class="Clust (strict)"("Value"=w2169) -> ()  [unwired: 2 in, 2 out]
            n795 = call "Enqueue Message.vi"("error in"=w2188, "Data"=w2169, "Message"="PID.Update", "Queue"=w2187) -> ("error out"=w2168:errorcluster)  [unwired: 6 in, 1 out]
          }
          frame "Controllers.IOFrequency" {
            n796 = Variant To Data(error in=w2216, type=u32 0 ("IO Frequency"), Variant=w2214) -> (data=w2206:u32, error out=w2215:errorcluster)
            n797 = call "FGVfpgaAdress.vi"("Enum"=Enum."Read", "error in"=w2215) -> ("ioFreqHzOut"=w2222:u32)  [unwired: 4 in, 5 out]
            n798 = call "corerceFPGAClock.vi"("baseClock"=w2222, "requestedFrequency"=w2206) -> ("error out"=w2221:errorcluster, "decimation"=w2219:u16, "realFrequency"=w2218:dbl)  [unwired: 7 in]
            n799 = local read "Mode"() -> (w2224:enum16{"Contact", "OR Tapping", "Aux"})
            n800 = To Unsigned Long Integer(number=w2218) -> (unsigned 32bit integer=w2205:u32)
            n801 = case shown="\"Contact\", \"Aux\", Default" w2224 {
              tunnel: w2205 -> [w2234 _]
              frame "Contact", "Aux", Default {
                n802 = call "FGVSamplingRates.vi"("Enum"=Enum."Read") -> ("samplingRatesOut"=w2236:T32)  [unwired: 9 in, 1 out]
                n803 = Bundle By Name(cluster=w2236, "feedbackHz"=w2234) -> (w2235:T32)
                n804 = call "FGVSamplingRates.vi"("Enum"=Enum."Write", "samplingRatesIn"=w2235) -> ()  [unwired: 8 in, 2 out]
              }
              frame "OR Tapping" {
                # "This is controlled from the \nexcitation window"
              }
            }
            n805 = xnode "Read/Write Control"("FPGA VI Reference In"=w2220, "error in"=w2221, "aio.i.samplingDecimation"=w2219) -> ("FPGA VI Reference Out"=w2211:T4, "error out"=w2210:errorcluster)
            n806 = call "IsVIRunning.vi"("error in (no error)"=w2210, "name or relative path"="FrontPanel\\SICM.vi") -> ("error out"=w2209:errorcluster, "RunningVI?"=w2208:bool)  [unwired: 8 in]
            n807 = case shown="True" w2208 {
              tunnel: [w2228 w2232] -> w2212
              tunnel: w2209 -> [w2228 w2231]
              tunnel: w2227 -> [_ w2230]
              frame False {
              }
              frame True {
                n808 = call "Enqueue Message.vi"("error in"=w2231, "Message"="SICM.SamplingDecimationUpdate", "Queue"=w2230) -> ("error out"=w2232:errorcluster)  [unwired: 7 in, 1 out]
              }
            }
          }
          frame "-------- SafeTip --------" {
            # "ALL THE CASES RELATED TO SAFE TIP ARE NOT USED"
          }
          frame "SafeTip.Enable" {
            n809 = Variant To Data(error in=w2261, type=FALSE ("NewVal"), Variant=w2260) -> (data=w2254:bool, error out=w2279:errorcluster)
            n810 = Unbundle By Name("SafeTip") -> ("SafeTipOn"=w2243:bool, "SafeTipValue"=w2244:dbl, ">/<"=w2245:enum16{">", "<"}, "SafeTipSignal"=w2246:u16)
            n811 = call "FGVSafeTip.vi"("Enum"=Enum."Read", "error in"=w2279) -> ("error out"=w2250:errorcluster, "SafeTipParametersOut"=w2249:T33)  [unwired: 7 in, 1 out]
            n812 = Bundle By Name(cluster=w2249, "SafeTipValue"=w2244, ">/<"=w2245, "SafeTipSignal"=w2246) -> (w2248:T33)
            n813 = call <vilib>:"Application Directory.vi"() -> ("Application Directory"=w2273:path)
            n814 = call "FGVSafeTip.vi"("Enum"=Enum."Write", "error in"=w2250, "SafeTipOn?"=w2243, "SafeTipParametersIn"=w2248) -> ("error out"=w2253:errorcluster)  [unwired: 5 in, 2 out]
            n815 = Build Path(base path=w2273, name or relative path="FrontPanel\\SafeTip.vi") -> (appended path=w2272:path)
            n816 = Open VI Reference(vi path=w2272, error in (no error)=w2253) -> (vi reference=w2271:refnum<vi>, error out=w2269:errorcluster)  [unwired: 4 in]
            n817 = property class="VI"(reference=w2271, error in=w2269) -> (reference out=w2270:refnum<vi>, error out=w2268:errorcluster, "Exec.State"=w2263:T18)
            n818 = Equal?(x=T18."Run top level" ("Execution:State"), y=w2263) -> (x = y?=w2265:bool)
            n819 = Equal?(x=w2263, y=T18."Running" ("Execution:State")) -> (x = y?=w2264:bool)
            n820 = Compound Arithmetic op=OR(w2265, w2264) -> (w2255:bool)
            n821 = case shown="False" w2254 {
              tunnel: w2270 -> [w2284 w2302]
              tunnel: w2268 -> [w2283 w2301]
              tunnel: T17."Hidden" ("State") -> [_ w2300]
              tunnel: [w2282 w2299] -> w2258
              tunnel: [w2281 w2298] -> w2257
              tunnel: w2255 -> [w2280 w2297]
              frame False {
                n822 = case shown="True" w2280 {
                  tunnel: [w2285 w2287] -> w2281
                  tunnel: [w2286 w2288] -> w2282
                  tunnel: w2284 -> [w2286 w2290]
                  tunnel: w2283 -> [w2285 w2289]
                  frame False {
                  }
                  frame True {
                    n823 = disable-structure shown="Enabled" {
                      disable-tunnel: w2290 -> [w2294 w2296]
                      disable-tunnel: w2289 -> [w2293 w2295]
                      disable-tunnel: [w2292 w2296] -> w2288
                      disable-tunnel: [w2291 w2295] -> w2287
                      frame Disabled {
                        n824 = invoke class="VI" method="Abort VI"(reference=w2294, error in=w2293) -> (reference out=w2292:refnum<vi>, error out=w2291:errorcluster)  [unwired: 1 in, 1 out]
                      }
                      frame Enabled {
                      }
                    }
                  }
                }
              }
              frame True {
                n825 = case shown="False" w2297 {
                  tunnel: [w2312 w2313] -> w2298
                  tunnel: [w2311 w2314] -> w2299
                  tunnel: w2302 -> [w2310 w2314]
                  tunnel: w2301 -> [w2309 w2313]
                  tunnel: w2300 -> [w2308 _]
                  frame False {
                    n826 = invoke class="VI" method="FP.Open"(reference=w2310, error in=w2309, "Activate"=TRUE ("Activate?"), "State"=w2308) -> (reference out=w2304:refnum<vi>, error out=w2303:errorcluster)  [unwired: 1 in, 3 out]
                    n827 = invoke class="VI" method="Run VI"(reference=w2304, error in=w2303, "Wait until done"=FALSE ("Wait Until Done"), "Auto Dispose Ref"=FALSE ("Auto Dispose Reference")) -> (reference out=w2311:refnum<vi>, error out=w2312:errorcluster)  [unwired: 1 in, 3 out]
                  }
                  frame True {
                  }
                }
              }
            }
            n828 = Close Reference(reference=w2258, error in (no error)=w2257) -> (error out=w2256:errorcluster)
          }
          frame "SafeTip.Update" {
            n829 = local read "SafeTip"() -> (w2315:T2)
            n830 = Unbundle By Name(w2315) -> ("SafeTipOn"=w2319:bool, "SafeTipValue"=w2320:dbl, ">/<"=w2321:enum16{">", "<"}, "SafeTipSignal"=w2322:u16)
            n831 = call "FGVSafeTip.vi"("Enum"=Enum."Read", "error in"=w2317) -> ("error out"=w2325:errorcluster, "SafeTipParametersOut"=w2324:T33)  [unwired: 7 in, 1 out]
            n832 = Bundle By Name(cluster=w2324, "SafeTipValue"=w2320, ">/<"=w2321, "SafeTipSignal"=w2322) -> (w2323:T33)
            n833 = call "FGVSafeTip.vi"("Enum"=Enum."Write", "error in"=w2325, "SafeTipOn?"=w2319, "SafeTipParametersIn"=w2323) -> ("error out"=w2316:errorcluster)  [unwired: 5 in, 2 out]
          }
          frame "SafeTip.UpdateRing" {
            n834 = Variant To Data(error in=w2341, type=refnum<vi> refnum ("CtlRef"), Variant=w2340) -> (data=w2338:refnum<vi>, error out=w2337:errorcluster)
            n835 = property class="Ring (strict)" props=["Label", "Text", "Value"](reference=w2338, error in=w2337) -> (error out=w2336:errorcluster, "Label.Text"=w2335:string)  [unwired: 2 out]
            n836 = case shown="\"SafeTipSignal\"" w2335 {
              tunnel: w2336 -> [w2343 w2347]
              tunnel: [w2343 w2345] -> w2342
              frame "False", Default {
              }
              frame "SafeTipSignal" {
                n837 = call "FGVChannels.vi"("Enum"=Enum."Read", "error in"=w2347) -> ("error out"=w2349:errorcluster, "channelsNamesOut"=w2344:string[])  [unwired: 5 in, 3 out]
                n838 = control-ref of="SafeTipSignal"() -> (w2346:refnum<vi>)
                n839 = property class="Ring (strict)"(reference=w2346, error in=w2349, "Strings []"=w2344) -> (error out=w2345:errorcluster)  [unwired: 1 out]
              }
            }
          }
          frame "SafeTip.Withdraw" {
            # "Change color of the feedback state diode in case SafeTip withdrawn has been activated"
            n840 = local read "Approaching?"() -> (w2359:bool)
            n841 = Select(t="AutoApproach.Stop" ("Message"), s=w2359, f="Z.ManualMotion.Withdraw" ("Message")) -> (s? t:f=w2356:string)
            n842 = call "Enqueue Message.vi"("Prioritary message"=TRUE ("Message prioritaire ? (F)"), "error in"=w2361, "Message"=w2356, "Queue"=w2363) -> ("error out"=w2352:errorcluster)  [unwired: 6 in, 1 out]
            n843 = property on="SafeTipOn" class="Bool (strict)"(error in=w2352, "Val(Sgnl)"=FALSE ("Value (Signaling)")) -> (error out=w2351:errorcluster)  [unwired: 1 in, 1 out]
          }
          frame "UserEvents.Calibration" {
            n844 = Variant To Data(error in=w2378, type=refnum<vi> refnum ("CtlRef"), Variant=w2377) -> (data=w2376:refnum<vi>, error out=w2375:errorcluster)
            n845 = property class="DigNum"(reference=w2376, error in=w2375) -> (error out=w2373:errorcluster, "Value"=w2372:variant)  [unwired: 1 out]
            n846 = Variant To Data(error in=w2373, type=0.0, Variant=w2372) -> (data=w2366:dbl, error out=w2381:errorcluster)
            n847 = Divide(x=w2366, y=2.0) -> (x/y=w2368:dbl)
            n848 = control-ref of="Z (m)"() -> (w2371:refnum<vi>)
            n849 = Negate(x=w2368) -> (-x=w2369:dbl)
            n850 = property class="Slide (strict)"(reference=w2371, error in=w2381, "Scale.Maximum"=w2368, "Scale.Minimum"=w2369) -> (error out=w2367:errorcluster)  [unwired: 1 out]
          }
          frame " ---- From other VIs ---- " {
          }
          frame "ZController.Engage" {
            # "Wait for Z-Controller\nto be switched on"
            # "Switch Z-Controller ON"
            n851 = Variant To Data(error in=w2396, type="", Variant=w2388) -> (data=w2389:string, error out=w2391:errorcluster)
            n852 = xnode "Read/Write Control"("FPGA VI Reference In"=w2398, "error in"=w2391, "fb.p.enable"=TRUE ("enableFeedback")) -> ("FPGA VI Reference Out"=w2413:T4, "error out"=w2412:errorcluster, "fb.p.limits.lowerLimit"=w2405:fxp<+/-,28,4>)
            n853 = while {
              tunnel: w2413 -> [w2436]
              tunnel: w2412 -> [w2435]
              tunnel: [w2432] -> w2410
              tunnel: [w2431] -> w2409
              stop <- w2434 stop-if-true
              n854 = xnode "Read/Write Control"("FPGA VI Reference In"=w2436, "error in"=w2435) -> ("FPGA VI Reference Out"=w2431:T4, "error out"=w2432:errorcluster, "fb.p.enable"=w2434:bool)
              n855 = Wait (ms)(milliseconds to wait=u32 2) -> ()  [unwired: 1 out]
            }
            n856 = local read "Ztreshold"() -> (w2414:dbl)
            n857 = To Double Precision Float(number=w2405) -> (double precision float=w2403:dbl)
            n858 = disable-structure shown="FPGA_BUILT==RIO0" {
              disable-tunnel: [w2428 10.0 ("voltageRange(+/-)Out")] -> w2402
              frame condition #0 (active) {
                n859 = call "FGVfpgaAdress.vi"("Enum"=Enum."Read") -> ("voltageRange(+/-)Out"=w2428:dbl)  [unwired: 5 in, 5 out]
              }
              frame condition #1 {
              }
            }
            n860 = Absolute Value(x=w2403) -> (abs(x)=w2404:dbl)
            n861 = Multiply(x=w2404, y=w2414) -> (x*y=w2406:dbl)
            n862 = while {
              shift-right: [w2438] -> _
              shift-left: -inf -> [w2460]
              tunnel: w2406 -> [w2459]
              tunnel: w2410 -> [w2458]
              tunnel: [w2456] -> w2400
              tunnel: [w2452] -> _
              tunnel: w2409 -> [w2446]
              tunnel: [w2442] -> w2401
              tunnel: w2402 -> [w2445]
              tunnel: fxp<+/-,17,1> 0.0 ("setPoint") -> [w2444]
              tunnel: T13 {"setPoint"=0.0, "pGain"=0.0, "iGain"=0.0, "setPointAlt"=0.0} ("fbParams") -> [w2443]
              tunnel: [w2437] -> w2399
              stop <- w2455 stop-if-true
              # "stop"
              n863 = xnode "Read/Write Control"("FPGA VI Reference In"=w2446, "error in"=w2458) -> ("FPGA VI Reference Out"=w2442:T4, "error out"=w2456:errorcluster, "fb.o.height"=w2457:fxp<+/-,31,4>)
              n864 = local read "PID"() -> (w2447:T1)
              n865 = Unbundle By Name(w2447) -> ("Setpoint"=w2448:dbl, "P Gain"=w2440:dbl, "I Gain"=w2439:dbl)
              n866 = To Double Precision Float(number=w2457) -> (double precision float=w2438:dbl)
              n867 = Greater?(x=w2438, y=w2460) -> (0:w2453:bool)
              n868 = Less?(x=w2438, y=w2459) -> (x < y?=w2452:bool)
              n869 = And(x=w2453, y=w2452) -> (x .and. y?=w2454:bool)
              n870 = property on="Stop" class="Bool (strict)"() -> ("Value"=w2441:bool)  [unwired: 2 in, 2 out]
              n871 = Not(x=w2454) -> (.not. x?=w2451:bool)
              n872 = Divide(x=w2448, y=w2445) -> (x/y=w2449:dbl)
              n873 = Or(x=w2451, y=w2441) -> (x .or. y?=w2455:bool)
              n874 = To Fixed-Point(fixed-point type=w2444, number=w2449) -> (fixed-point=w2450:fxp<+/-,17,1>)
              n875 = Bundle By Name(cluster=w2443, "setPoint"=w2450, "pGain"=w2440, "iGain"=w2439) -> (w2437:T13)
              n876 = call "PIDParameters.vi"("fbParams"=w2437, "FPGA VI Reference In"=w2446) -> ()  [unwired: 8 in, 2 out]
            }
            n877 = case shown="\"Error\"" w2389 {
              tunnel: w2401 -> [w2418 w2425]
              tunnel: w2400 -> [w2419 w2424]
              tunnel: w2399 -> [_ w2423]
              tunnel: [w2418 w2421] -> w2397
              tunnel: [w2419 w2420] -> w2395
              frame Default {
              }
              frame "Error" {
                n878 = Bundle By Name(cluster=w2423, "pGain"=0.0, "iGain"=1e-05) -> (w2422:T13)
                n879 = call "PIDParameters.vi"("error in"=w2424, "fbParams"=w2422, "FPGA VI Reference In"=w2425) -> ("error out"=w2420:errorcluster, "FPGA VI Reference Out"=w2421:T4)  [unwired: 7 in]
              }
            }
            n880 = call "FGVTriggerQueue.vi"("Enum"=Enum."Write", "error in"=w2395, "Ready IN ?"=TRUE) -> ("error out"=w2394:errorcluster)  [unwired: 7 in, 1 out]
          }
          frame "Feedback.PIDUpdate" {
            n881 = property on="PID" class="Clust (strict)"() -> ("Value"=w2466:T1)  [unwired: 2 in, 2 out]
            n882 = call "Enqueue Message.vi"("error in"=w2469, "Data"=w2466, "Message"="PID.Update", "Queue"=w2468) -> ("error out"=w2464:errorcluster, "Queue dup."=w2473:refnum<queue>)  [unwired: 6 in]
            n883 = call "Enqueue Message.vi"("error in"=w2464, "Data"=TRUE, "Message"="Feedback.Enable", "Queue"=w2473) -> ("error out"=w2463:errorcluster)  [unwired: 6 in, 1 out]
          }
          frame "SICM.SamplingDecimationUpdate" {
            n884 = Obtain Queue(name (unnamed)="SiCM" ("QueueName"), element data type=T16 {"Message"="", "Données de message"=variant} ("Cluster Message"), error in (no error)=w2477) -> (queue out=w2484:refnum<queue>, error out=w2476:errorcluster)  [unwired: 2 in, 1 out]
            n885 = call "Enqueue Message.vi"("error in"=w2476, "Message"="ZController.IOFrequency", "Queue"=w2484) -> ("error out"=w2478:errorcluster)  [unwired: 7 in, 1 out]
          }
          frame "Exit" {
            n886 = call "Fire User Event - Stop.vi"("Événement utilisateur - Arrêt"=w2487) -> ("sortie d'erreur"=w2486:errorcluster)  [unwired: 10 in]
            n887 = Release Queue(queue=w2495, error in (no error)=w2492) -> (error out=w2494:errorcluster)  [unwired: 1 in, 2 out]
            n888 = Merge Errors(w2486, w2494) -> (w2493:errorcluster)
          }
          frame Default {
            n889 = Format Into String(format string="The message\"%s\" received in the gestion loop is not valid" ("Texte de message d'erreur inconnu"), w2503) -> (resulting string=w2500:string)  [unwired: 2 in, 1 out]
            n890 = call <vilib>:"Error Cluster From Error Code.vi"("error message (\"\")"=w2500, "error code (0)"=1 ("code d'erreur (0)")) -> ("error out"=w2501:errorcluster)  [unwired: 7 in]
          }
        }
      }
      n891 = while {
        tunnel: w55 -> [w186]
        tunnel: w37 -> [w184]
        tunnel: [w183] -> w36
        stop <- w182 stop-if-true
        n892 = event shown="[0] Timeout" {
          selector: w184 -> [_ _]
          dyn-events: [_ _] -> w183
          timeout: 100 -> [_ _]
          tunnel: w186 -> [w187 _]
          tunnel: [_ TRUE] -> w182
          event Timeout {
            # "Update Zheight slider"
            n893 = event-data() -> ()  [unwired: 1 in, 1 out]
            n894 = local read "Display Z"() -> (w188:bool)
            n895 = case shown="True" w188 {
              tunnel: w187 -> [w191 _]
              frame True {
                n896 = call "FGVCalibrations.vi"("Enum"=Enum."Read") -> ("calibOut"=w201:T22)  [unwired: 9 in, 1 out]
                n897 = Unbundle By Name(w201) -> ("calibParameters"=w200:T23, "calibIndex"=w190:i32)
                n898 = xnode "Read/Write Control"("FPGA VI Reference In"=w191) -> ("FPGA VI Reference Out"=w189:T4, "fb.o.height"=w202:fxp<+/-,31,4>)  [unwired: 1 in, 1 out]
                n899 = xnode "Read/Write Control"("FPGA VI Reference In"=w189) -> ()  [unwired: 1 in, 3 out]
                n900 = Index Array(array=w200, index=w190) -> (element=w199:T24)
                n901 = Unbundle By Name(w199) -> ("Range.Range Z"=w197:dbl)
                n902 = To Double Precision Float(number=w202) -> (double precision float=w198:dbl)
                n903 = Divide(x=w197, y=2.0) -> (x/y=w195:dbl)
                n904 = Multiply(x=w195, y=w198) -> (x*y=w193:dbl)
                n905 = control-ref of="Z (m)"() -> (w194:refnum<vi>)
                n906 = property class="Slide (strict)"(reference=w194, "Value"=w193) -> ()  [unwired: 1 in, 2 out]
              }
              frame False {
              }
            }
          }
          event User Event {
            n907 = event-data() -> ()  [unwired: 1 in, 1 out]
          }
        }
      }
      n908 = while {
        tunnel: w50 -> [w2514]
        tunnel: [w2510] -> w54
        tunnel: w55 -> [w2507]
        tunnel: w47 -> [w2509]
        tunnel: [w2508] -> w53
        shift-right: [w2506] -> _
        shift-left: u32 0 ("Time") -> [w2505]
        stop <- w2512 stop-if-true
        n909 = event shown="[2] \"Mode\": Value Change" {
          selector: w2509 -> [_ _ _ _ _ _ _ _ _ _ _ _ _ _ _ _ _ _]
          dyn-events: [_ _ _ _ _ _ _ _ _ _ _ _ _ _ _ _ _ _] -> w2508
          timeout: _ -> [_ _ _ _ _ _ _ _ _ _ _ _ _ _ _ _ _ _]
          tunnel: [_ _ _ _ _ _ _ _ _ _ _ _ _ _ _ _ w2805 _] -> w2513
          tunnel: w2514 -> [w2530 w2558 w2598 w2608 w2630 w2665 w2692 w2710 w2726 w2748 w2754 w2759 w2767 w2773 w2780 w2792 w2806 w2816]
          tunnel: [w2529 w2556 w2593 w2606 w2628 w2663 w2690 w2708 w2727 w2741 _ w2756 w2765 _ w2775 w2785 w2801 w2813] -> w2510
          tunnel: [w2528 w2557 w2597 w2607 w2629 w2664 w2691 w2709 w2725 w2743 w2751 w2758 w2764 w2773 w2779 w2786 w2802 w2814] -> w2511
          tunnel: w2507 -> [_ _ _ _ _ _ _ _ _ _ _ _ _ _ _ _ _ _]
          tunnel: [w2525 w2552 w2592 w2599 w2626 w2658 w2683 w2707 w2720 w2739 w2753 w2760 w2761 w2768 w2774 w2791 w2793 w2810] -> w2506
          tunnel: w2505 -> [w2525 w2552 w2592 w2599 _ w2658 w2683 w2707 w2720 w2739 w2753 w2760 w2761 w2768 w2774 w2791 w2793 w2810]
          event "Motor.Up", "Motor.Down": Value Change {
            n910 = event-data() -> ("CtlRef"=w2527:refnum<vi>, "NewVal"=w2526:bool)  [unwired: 1 in]
            n911 = case shown="True" w2526 {
              tunnel: w2530 -> [w2532 w2547]
              tunnel: [w2533 w2545] -> w2529
              tunnel: [w2534 w2544] -> w2528
              tunnel: w2527 -> [_ w2543]
              tunnel: "Type" -> [w2531 w2542]
              frame False {
                n912 = Flush Queue(queue=w2532) -> (queue out=w2537:refnum<queue>)  [unwired: 1 in, 2 out]
                n913 = case shown="\"DC motor\"" w2531 {
                  tunnel: ["StepMotor.StopSteps" ("Message") "DCMotor.Stop" ("Message") "SmdInterface.Stop" ("Message") "StickSlip.Stop" ("Message")] -> w2536
                  frame "Step motor", Default {
                  }
                  frame "DC motor" {
                  }
                  frame "Stepper Motor Driver" {
                  }
                  frame "Stick-Slip" {
                  }
                }
                n914 = call "Enqueue Message.vi"("Prioritary message"=TRUE ("Message prioritaire ? (F)"), "Message"=w2536, "Queue"=w2537) -> ("error out"=w2533:errorcluster, "Queue dup."=w2534:refnum<queue>)  [unwired: 7 in]
              }
              frame True {
                n915 = case shown="\"Stepper Motor Driver\"" w2542 {
                  tunnel: ["StepMotor.DoSteps" ("Message") "DCMotor.SendVoltage" ("Message") "SmdInterface.Start" ("Message") "StickSlip.Move" ("Message")] -> w2546
                  frame "Step motor", Default {
                  }
                  frame "DC motor" {
                  }
                  frame "Stepper Motor Driver" {
                  }
                  frame "Stick-Slip" {
                  }
                }
                n916 = call "Enqueue Message.vi"("Data"=w2543, "Message"=w2546, "Queue"=w2547) -> ("error out"=w2545:errorcluster, "Queue dup."=w2544:refnum<queue>)  [unwired: 7 in]
              }
            }
          }
          event "AutoApproach.Start", "AutoApproach.Stop": Mouse Down {
            n917 = event-data() -> ("CtlRef"=w2555:refnum<vi>)  [unwired: 1 in]
            n918 = property class="Bool (strict)"(reference=w2555) -> ("Label.Text"=w2554:string)  [unwired: 1 in, 2 out]
            n919 = case shown="\"Stop\", Default" w2554 {
              tunnel: w2558 -> [w2562 w2591]
              tunnel: [w2561 w2590] -> w2557
              tunnel: [w2560 w2589] -> w2556
              tunnel: "Slow" -> [w2559 w2585]
              frame "Stop", Default {
                n920 = Flush Queue(queue=w2562) -> (queue out=w2563:refnum<queue>)  [unwired: 1 in, 2 out]
                n921 = case shown="True" w2559 {
                  tunnel: w2563 -> [w2566 w2584]
                  tunnel: [w2565 w2583] -> w2561
                  tunnel: [w2564 w2582] -> w2560
                  frame False {
                    n922 = disable-structure shown="Enabled" {
                      disable-tunnel: w2566 -> [w2570 w2579]
                      disable-tunnel: [w2569 w2578] -> w2565
                      disable-tunnel: [w2568 w2577] -> w2564
                      frame Disabled {
                        n923 = local read "Approaching?"() -> (w2567:bool)
                        n924 = case shown="False" w2567 {
                          tunnel: w2570 -> [w2574 w2575]
                          tunnel: [w2573 w2575] -> w2569
                          tunnel: [w2572 _] -> w2568
                          frame False {
                            n925 = call "Enqueue Message.vi"("Message"="Z.ManualMotion.Withdraw", "Queue"=w2574) -> ("error out"=w2572:errorcluster, "Queue dup."=w2573:refnum<queue>)  [unwired: 8 in]
                          }
                          frame True {
                          }
                        }
                      }
                      frame Enabled {
                        n926 = call "Enqueue Message.vi"("Message"="AutoApproachFast.Stop", "Queue"=w2579) -> ("error out"=w2577:errorcluster, "Queue dup."=w2578:refnum<queue>)  [unwired: 8 in]
                      }
                    }
                  }
                  frame True {
                    n927 = call "Enqueue Message.vi"("Prioritary message"=TRUE ("Message prioritaire ? (F)"), "Message"="AutoApproach.Stop", "Queue"=w2584) -> ("error out"=w2582:errorcluster, "Queue dup."=w2583:refnum<queue>)  [unwired: 7 in]
                  }
                }
              }
              frame "Start" {
                n928 = Select(t="AutoApproach.Init" ("Message"), s=w2585, f="AutoApproachFast.Init" ("Message")) -> (s? t:f=w2587:string)
                n929 = call "Enqueue Message.vi"("Message"=w2587, "Queue"=w2591) -> ("error out"=w2589:errorcluster, "Queue dup."=w2590:refnum<queue>)  [unwired: 8 in]
              }
            }
          }
          event "Mode": Value Change {
            n930 = event-data() -> ("NewVal"=w2595:enum16{"Contact", "OR Tapping", "Aux"})  [unwired: 1 in]
            n931 = To Variant(anything=w2595) -> (Variant=w2594:variant)
            n932 = call "Enqueue Message.vi"("Data"=w2594, "Message"="Mode.Update", "Queue"=w2598) -> ("error out"=w2593:errorcluster, "Queue dup."=w2597:refnum<queue>)  [unwired: 7 in]
          }
          event "Feedback On": Mouse Down {
            n933 = event-data() -> ("CtlRef"=w2605:refnum<vi>)  [unwired: 1 in]
            n934 = property class="Bool (strict)"(reference=w2605) -> (reference out=w2601:refnum<vi>, error out=w2600:errorcluster, "Value"=w2604:bool, "Caption.Text"=w2603:string)  [unwired: 1 in]
            n935 = case shown="False" w2604 {
              selector: w2604 -> [_ w2620]
              tunnel: w2608 -> [w2614 w2624]
              tunnel: [w2618 w2623] -> w2607
              tunnel: [w2617 w2622] -> w2606
              tunnel: w2603 -> [_ _]
              tunnel: [FALSE ("display height") TRUE ("display height")] -> w2602
              tunnel: w2601 -> [_ _]
              tunnel: w2600 -> [_ _]
              frame False {
                w2612 = -1.0  # HeightTarget(0-2)
                w2616 = FALSE  # doMove
                w2615 = TRUE  # enableManualMotion
                n936 = Bundle("enableManualMotion"=w2615, "doMove"=w2616, "HeightTarget(0-2)"=w2612) -> (w2611:T34)  [unwired: 1 in]
                n937 = To Variant(anything=w2611) -> (Variant=w2609:variant)
                n938 = call "Enqueue Message.vi"("Data"=w2609, "Message"="Z.ManualMotion", "Queue"=w2614) -> ("error out"=w2617:errorcluster, "Queue dup."=w2618:refnum<queue>)  [unwired: 7 in]
              }
              frame True {
                n939 = call "Enqueue Message.vi"("Data"=w2620, "Message"="Feedback.Enable", "Queue"=w2624) -> ("error out"=w2622:errorcluster, "Queue dup."=w2623:refnum<queue>)  [unwired: 7 in]
              }
            }
            n940 = local write "Display Z"(w2602) -> ()
          }
          event "Withdraw": Mouse Down {
            n941 = event-data() -> ("CtlRef"=w2627:refnum<vi>, "Time"=w2625:u32)  [unwired: 1 in]
            n942 = disable-structure shown="Enabled" {
              disable-tunnel: w2630 -> [w2637 w2653]
              disable-tunnel: [w2636 w2653] -> w2629
              disable-tunnel: [w2634 _] -> w2628
              disable-tunnel: w2627 -> [w2633 _]
              disable-tunnel: [_ w2654] -> w2626
              disable-tunnel: w2625 -> [_ w2654]
              frame Disabled {
                n943 = property class="Bool (strict)"(reference=w2633) -> ("Value"=w2632:bool, "Caption.Text"=w2631:string)  [unwired: 1 in, 2 out]
                n944 = case shown="True" w2632 {
                  tunnel: [errorcluster {"status"=FALSE, "code"=0, "source"=""} ("sortie d'erreur") w2644] -> w2635
                  tunnel: w2637 -> [w2641 w2652]
                  tunnel: [w2641 w2645] -> w2636
                  tunnel: w2631 -> [_ w2647]
                  frame False {
                  }
                  frame True {
                    w2648 = 0.0  # Height Lift
                    w2650 = TRUE  # doMove
                    w2649 = TRUE  # enableManualMotion
                    n945 = Bundle("enableManualMotion"=w2649, "doMove"=w2650, "Height Lift"=w2648, "Caption.Text"=w2647) -> (w2646:T35)  [unwired: 1 in]
                    n946 = To Variant(anything=w2646) -> (Variant=w2642:variant)
                    n947 = call "Enqueue Message.vi"("Prioritary message"=TRUE ("Message prioritaire ? (F)"), "Data"=w2642, "Message"="Z.ManualMotion.Withdraw", "Queue"=w2652) -> ("error out"=w2644:errorcluster, "Queue dup."=w2645:refnum<queue>)  [unwired: 6 in]
                  }
                }
                n948 = flat-sequence {
                  tunnel: w2635 -> [w2639]
                  tunnel: [w2639] -> w2634
                  tunnel: [FALSE ("Withdraw")] -> _
                  frame #0 {
                  }
                }
              }
              frame Enabled {
              }
            }
          }
          event "Withdraw": Mouse Up {
            # "If the user clicks for more than 2s on withdraw, the motor will move up !"
            n949 = event-data() -> ("CtlRef"=w2662:refnum<vi>, "Time"=w2659:u32)  [unwired: 1 in]
            n950 = Subtract(x=w2659, y=w2658) -> (x-y=w2657:u32)
            n951 = Less?(x=w2657, y=2000) -> (x < y?=w2655:bool)
            n952 = property class="Bool (strict)"(reference=w2662) -> ("Value"=w2660:bool)  [unwired: 1 in, 2 out]
            n953 = case shown="True" w2660 {
              tunnel: [errorcluster {"status"=FALSE, "code"=0, "source"=""} ("sortie d'erreur") w2671] -> w2661
              tunnel: w2665 -> [w2669 w2673]
              tunnel: [w2669 w2672] -> w2664
              tunnel: w2655 -> [_ w2670]
              frame False {
              }
              frame True {
                n954 = case shown="True" w2670 {
                  tunnel: w2673 -> [w2677 w2682]
                  tunnel: [w2675 w2680] -> w2672
                  tunnel: [w2674 w2679] -> w2671
                  frame False {
                    n955 = call "Enqueue Message.vi"("Message"="WithdrawAndMove", "Queue"=w2677) -> ("error out"=w2674:errorcluster, "Queue dup."=w2675:refnum<queue>)  [unwired: 8 in]
                  }
                  frame True {
                    n956 = call "Enqueue Message.vi"("Prioritary message"=TRUE ("Message prioritaire ? (F)"), "Message"="Z.ManualMotion.Withdraw", "Queue"=w2682) -> ("error out"=w2679:errorcluster, "Queue dup."=w2680:refnum<queue>)  [unwired: 7 in]
                  }
                }
              }
            }
            n957 = flat-sequence {
              tunnel: w2661 -> [w2667]
              tunnel: [w2667] -> w2663
              tunnel: [FALSE ("Withdraw")] -> _
              frame #0 {
              }
            }
          }
          event "Lift": Mouse Down {
            w2688 = TRUE  # enableManualMotion
            w2686 = TRUE  # doMove
            n958 = event-data() -> ()  [unwired: 1 in, 2 out]
            n959 = Bundle("enableManualMotion"=w2688, "doMove"=w2686, "liftHeight"="liftHeight") -> (w2687:T15)  [unwired: 1 in]
            n960 = To Variant(anything=w2687) -> (Variant=w2684:variant)
            n961 = call "Enqueue Message.vi"("Data"=w2684, "Message"="Z.ManualMotion.Lift", "Queue"=w2692) -> ("error out"=w2690:errorcluster, "Queue dup."=w2691:refnum<queue>)  [unwired: 7 in]
          }
          event "PID": Value Change {
            # "If the mouse wheel is used, the value of the I gain can not go from positive to negative"
            n962 = event-data() -> ("OldVal"=w2703:T1, "NewVal"=w2700:T1, "Type"=w2702:T19)  [unwired: 1 in]
            n963 = Unbundle By Name(w2703) -> ("I Gain"=w2698:dbl)
            n964 = Unbundle By Name(w2700) -> ("I Gain"=w2699:dbl)
            n965 = Equal?(x=w2702, y=lveventtype."Mouse Wheel" ("Type")) -> (x = y?=w2695:bool)
            n966 = Sign(1:w2698) -> (0:w2697:dbl)
            n967 = Sign(1:w2699) -> (0:w2696:dbl)
            n968 = Not Equal?(x=w2697, y=w2696) -> (x != y?=w2694:bool)
            n969 = And(x=w2694, y=w2695) -> (x .and. y?=w2693:bool)
            n970 = property on="Approaching?" class="Bool (strict)"() -> ("Value"=w2706:bool)  [unwired: 2 in, 2 out]
            n971 = property on="Slow" class="Bool (strict)"() -> ("Value"=w2705:bool)  [unwired: 2 in, 2 out]
            n972 = Compound Arithmetic op=AND(w2693, w2706, w2705) -> (w2704:bool)
            n973 = case shown="False" w2704 {
              tunnel: w2710 -> [w2717 w2719]
              tunnel: [w2716 w2719] -> w2709
              tunnel: [w2715 errorcluster {"status"=FALSE, "code"=0, "source"=""} ("error out")] -> w2708
              tunnel: w2700 -> [w2714 _]
              frame False {
                n974 = To Variant(anything=w2714) -> (Variant=w2711:variant)
                n975 = call "Enqueue Message.vi"("Prioritary message"=TRUE ("Message prioritaire ? (F)"), "Data"=w2711, "Message"="PID.Update", "Queue"=w2717) -> ("error out"=w2715:errorcluster, "Queue dup."=w2716:refnum<queue>)  [unwired: 6 in]
              }
              frame True {
              }
            }
          }
          event "Z (m)": Mouse Down {
            n976 = event-data() -> ("CtlRef"=w2722:refnum<vi>)  [unwired: 1 in]
            n977 = property class="Slide (strict)"(reference=w2722) -> ("Value"=w2723:dbl)  [unwired: 1 in, 2 out]
            n978 = Not(x="Feedback On") -> (.not. x?=w2724:bool)
            n979 = case shown="True" w2724 {
              tunnel: [errorcluster {"status"=FALSE, "code"=0, "source"=""} ("sortie d'erreur") w2738] -> w2727
              tunnel: w2726 -> [w2729 w2737]
              tunnel: [w2729 w2736] -> w2725
              tunnel: w2723 -> [_ w2731]
              frame False {
              }
              frame True {
                w2732 = TRUE ("enableManualMotion")
                n980 = Bundle(cluster=T15 {"enableManualMotion"=FALSE, "doMove"=FALSE, "liftHeight"=0.0} ("output cluster"), "enableManualMotion"=w2732, "doMove"=w2732, "liftHeight"=w2731) -> (w2733:T15)
                n981 = To Variant(anything=w2733) -> (Variant=w2730:variant)
                n982 = call "Enqueue Message.vi"("Data"=w2730, "Message"="Z.ManualMotion", "Queue"=w2737) -> ("error out"=w2738:errorcluster, "Queue dup."=w2736:refnum<queue>)  [unwired: 7 in]
              }
            }
          }
          event "Z (m)": Value Change {
            w2744 = TRUE ("enableManualMotion")
            n983 = event-data() -> ("NewVal"=w2742:dbl)  [unwired: 1 in]
            n984 = Bundle(cluster=T15 {"enableManualMotion"=FALSE, "doMove"=FALSE, "liftHeight"=0.0} ("output cluster"), "enableManualMotion"=w2744, "doMove"=w2744, "liftHeight"=w2742) -> (w2745:T15)
            n985 = To Variant(anything=w2745) -> (Variant=w2740:variant)
            n986 = call "Enqueue Message.vi"("Data"=w2740, "Message"="Z.ManualMotion", "Queue"=w2748) -> ("error out"=w2741:errorcluster, "Queue dup."=w2743:refnum<queue>)  [unwired: 7 in]
          }
          event "SafeTip.SafeTipOn": Value Change {
            n987 = event-data() -> ("NewVal"=w2750:bool)  [unwired: 1 in]
            n988 = To Variant(anything=w2750) -> (Variant=w2749:variant)
            n989 = call "Enqueue Message.vi"("Data"=w2749, "Message"="SafeTip.Enable", "Queue"=w2754) -> ("Queue dup."=w2751:refnum<queue>)  [unwired: 7 in, 1 out]
          }
          event "SafeTip": Value Change {
            n990 = event-data() -> ("NewVal"=w2755:T2)  [unwired: 1 in]
            n991 = call "Enqueue Message.vi"("Data"=w2755, "Message"="SafeTip.Update", "Queue"=w2759) -> ("error out"=w2756:errorcluster, "Queue dup."=w2758:refnum<queue>)  [unwired: 7 in]
          }
          event "SafeTip.SafeTipSignal": Mouse Down {
            n992 = event-data() -> ("CtlRef"=w2763:refnum<vi>)  [unwired: 1 in]
            n993 = To Variant(anything=w2763) -> (Variant=w2762:variant)
            n994 = call "Enqueue Message.vi"("Data"=w2762, "Message"="SafeTip.UpdateRing", "Queue"=w2767) -> ("error out"=w2765:errorcluster, "Queue dup."=w2764:refnum<queue>)  [unwired: 7 in]
          }
          event "Type": Value Change {
            n995 = event-data() -> ("NewVal"=w2772:T3)  [unwired: 1 in, 2 out]
            n996 = Equal?(x=w2772, y=enum16{"Step motor", "DC motor"}."DC motor") -> (x = y?=w2770:bool)
            n997 = Not(x=w2770) -> (.not. x?=w2769:bool)
            n998 = property on="DCVoltage" class="DigNum (strict)"("Visible"=w2770) -> ()  [unwired: 2 in, 2 out]
            n999 = property on="ms" class="DigNum (strict)"("Visible"=w2770) -> ()  [unwired: 2 in, 2 out]
            n1000 = property on="Steps" class="DigNum (strict)"("Visible"=w2769) -> ()  [unwired: 2 in, 2 out]
            n1001 = property on="Zstep" class="DigNum (strict)"("Visible"=w2769) -> ()  [unwired: 2 in, 2 out]
          }
          event "InvertHeight": Value Change {
            n1002 = event-data() -> ("NewVal"=w2778:bool)  [unwired: 1 in]
            n1003 = To Variant(anything=w2778) -> (Variant=w2777:variant)
            n1004 = call "Enqueue Message.vi"("Data"=w2777, "Message"="Height.Invert", "Queue"=w2780) -> ("error out"=w2775:errorcluster, "Queue dup."=w2779:refnum<queue>)  [unwired: 7 in]
          }
          event "IO Frequency": Value Change {
            n1005 = event-data() -> ("NewVal"=w2784:u32)  [unwired: 1 in]
            n1006 = call "FGVfpgaAdress.vi"("Enum"=Enum."Read") -> ("ioFreqHzOut"=w2789:u32)  [unwired: 5 in, 5 out]
            n1007 = call "corerceFPGAClock.vi"("baseClock"=w2789, "requestedFrequency"=w2784) -> ("error out"=w2787:errorcluster, "realFrequency"=w2783:dbl)  [unwired: 7 in, 1 out]
            n1008 = To Unsigned Long Integer(number=w2783) -> (unsigned 32bit integer=w2782:u32)
            n1009 = local write "IO Frequency"(w2782) -> ()
            n1010 = To Variant(anything=w2784) -> (Variant=w2781:variant)
            n1011 = call "Enqueue Message.vi"("error in"=w2787, "Data"=w2781, "Message"="Controllers.IOFrequency", "Queue"=w2792) -> ("error out"=w2785:errorcluster, "Queue dup."=w2786:refnum<queue>)  [unwired: 6 in]
          }
          event Panel Close? {
            w2805 = TRUE ("Rejeter ?")
            n1012 = event-data() -> ()  [unwired: 1 in, 1 out]
            n1013 = Flush Queue(queue=w2806) -> (queue out=w2808:refnum<queue>)  [unwired: 1 in, 2 out]
            n1014 = call "Enqueue Message.vi"("Message"="Z.ManualMotion.Withdraw", "Queue"=w2808) -> ("error out"=w2798:errorcluster, "Queue dup."=w2807:refnum<queue>)  [unwired: 8 in]
            n1015 = call "FGVSessionPath.vi"("Enum"=Enum."Read") -> ("sessionPathOut"=w2797:path)  [unwired: 9 in, 1 out]
            n1016 = Build Path(base path=w2797, name or relative path="Settings.txt") -> (appended path=w2794:path)
            n1017 = call "Enqueue Message.vi"("error in"=w2798, "Data"=w2794, "Message"="Configuration.Write", "Queue"=w2807) -> ("error out"=w2799:errorcluster, "Queue dup."=w2809:refnum<queue>)  [unwired: 6 in]
            n1018 = call "Enqueue Message.vi"("error in"=w2799, "Message"="Exit", "Queue"=w2809) -> ("error out"=w2801:errorcluster, "Queue dup."=w2802:refnum<queue>)  [unwired: 7 in]
            n1019 = event-data ("Event Filter Node")("Discard?"=w2805) -> ()  [unwired: 1 in, 1 out]
          }
          event Value Change {
            n1020 = event-data() -> ("CtlRef"=w2812:refnum<vi>)  [unwired: 1 in]
            n1021 = To Variant(anything=w2812) -> (Variant=w2811:variant)
            n1022 = call "Enqueue Message.vi"("Data"=w2811, "Message"="UserEvents.Calibration", "Queue"=w2816) -> ("error out"=w2813:errorcluster, "Queue dup."=w2814:refnum<queue>)  [unwired: 7 in]
          }
        }
        n1023 = case shown="Error" w2510 {
          tunnel: [w2515 TRUE ("Rejeter ?")] -> w2512
          tunnel: w2513 -> [w2515 _]
          tunnel: w2511 -> [_ w2523]
          frame No Error {
          }
          frame Error {
            w2516 = TRUE ("Message prioritaire ? (F)")
            n1024 = call "Enqueue Message.vi"("Prioritary message"=w2516, "Data"=FALSE ("Message prioritaire ? (F)"), "Message"="Feedback.Enable", "Queue"=w2523) -> ("error out"=w2517:errorcluster, "Queue dup."=w2522:refnum<queue>)  [unwired: 6 in]
            n1025 = call "Enqueue Message.vi"("Prioritary message"=w2516, "error in"=w2517, "Message"="Exit", "Queue"=w2522) -> ()  [unwired: 6 in, 2 out]
          }
        }
      }
      n1026 = Unregister For Events(event registration refnum=w53, error in=w54) -> (error out=w52:errorcluster)
      n1027 = Close Reference(reference=w39, error in (no error)=w52) -> (error out=w40:errorcluster)
      n1028 = Unregister For Events(event registration refnum=w36) -> (error out=w35:errorcluster)  [unwired: 1 in]
      n1029 = Merge Errors(w40, w48, w35) -> (w42:errorcluster)
      n1030 = call <vilib>:"Simple Error Handler.vi"("error in (no error)"=w42) -> ("error out"=w34:errorcluster)  [unwired: 4 in, 4 out]
      n1031 = call "Destroy User Event - Stop.vi"("entrée d'erreur (pas d'erreur)"=w34, "Événement utilisateur - Arrêt"=w32) -> ("sortie d'erreur"=w33:errorcluster)  [unwired: 9 in]
      n1032 = case shown="True" w41 {
        tunnel: w56 -> [_ w174]
        tunnel: w33 -> [_ w173]
        frame False {
        }
        frame True {
          n1033 = xnode "Invoke Method"("FPGA VI Reference In"=w174, "error in"=w173) -> ("FPGA VI Reference Out"=w171:T4, "error out"=w172:errorcluster)
          n1034 = xnode "Close FPGA VI Reference"("FPGA VI Reference In"=w171, "error in"=w172) -> ()  [unwired: 1 out]
        }
      }
    }
  }
